vi "mainui.vi"() -> ()   [LabVIEW 2011]
uses:
  <vilib>/Platform/TimedLoop/XDataNode/timing_clust.ctl
  <vilib>/Platform/TimedLoop/XDataNode/nitl_modes.ctl
  <vilib>/Platform/TimedLoop/XDataNode/wakeup.ctl
  <vilib>/Utility/config.llb/Read Key (Double).vi
  <vilib>/Utility/config.llb/Read Key (I32).vi
  <vilib>/Utility/config.llb/Read Key (String).vi
  <vilib>/Utility/config.llb/Write Key (Double).vi
  <vilib>/Utility/config.llb/Write Key (I32).vi
  <vilib>/Utility/config.llb/Write Key (String).vi
  <vilib>/Platform/TimedLoop/XDataNode/XDataNode.xnode
  API/API DYM.lvlib
  <vilib>/Platform/TimedLoop/XDataNode/XDNodeRunTimeDep.lvlib
  <vilib>/Utility/config.llb/NI_LVConfig.lvlib
  API/ColorSensorlib.lvlib
panel:
  in  "Color_String":string
  out "Plat2CurrentY_Adv":i32
  out "Plat2CurrentX_Adv":i32
  out "Plat3CurrentY_Adv":i32
  out "Plat3CurrentX_Adv":i32
  out "while-control":bool
  out "Sensor array output":i32[](array[numeric])
  out "Plat2CurrentY":i32
  out "Plat2CurrentX":i32
  out "platformStatue0 output":i32[](array[numeric])
  out "platformStatue1 output":i32[](array[numeric])
  out "platformStatue2 output":i32[](array[numeric])
  out "CurrentPosY":i32
  out "CurrentPosX":i32
  out "motor statue array output":i32[](array[numeric])
  out "solenstatue output":i32[](array[numeric])
  in  "选项卡控件Next":T1(tab)
  in  "BaseBtn":bool
  in  "MotinAdv":bool
  in  "restartbtn":bool
  in  "No1Btn":bool
  in  "No2Btn":bool
  in  "No3Btn":bool
  in  "TogStartBtn":bool
  in  "TogReturnBtn":bool
  in  "TogStopBtn":bool
  in  "Plat1StopBtn":bool
  in  "Plat1ReturnBtn":bool
  in  "Plat1Btn":bool
  in  "Plat2Btn":bool
  in  "Plat2ReturnBtn":bool
  in  "Plat2StopBtn":bool
  in  "Plat3GetMegBtn":bool
  in  "Plat3MulitBtn":bool
  in  "Plat3ReturnBtn":bool
  in  "Plat3StopBtn":bool
  in  "Plat3Btn":bool
  in  "Sensor":bool
  in  "选项卡控件":T2(tab)
  out "Blue":i32
  out "Green":i32
  out "红外计数":dbl
  out "电涡流计数":dbl
  out "红外电平":i32
  out "电涡流电平":i32
  out "电容1":i32
  out "电容2":i32
  out "电容3":i32
  out "电桥电平":dbl
  out "电桥称重":dbl
  out "Waveform Chart":dynamicdata(graph)
  in  "颜色盒":u32(colorbox)
  out "Red":i32
  out "Red_Last":i32
  out "Green_Last":i32
  out "Blue_Last":i32
  in  "Collection_Color":u32(colorbox)
  out "Property_T":string
  out "M1":bool
  out "M2":bool
  out "M3":bool
  out "M4":bool
  out "M5":bool
  out "M6":bool
  out "Plat3IO1":bool
  out "Plat3IO2":bool
  out "Plat3IO3":bool
  out "Plat3IO4":bool
  out "Plat3IO5":bool
  out "Plat3IO6":bool
  out "Plat3IO7":bool
  out "Plat3IO8":bool
  out "Plat2IO1":bool
  out "Plat2IO2":bool
  out "Plat2IO3":bool
  out "Plat2IO4":bool
  out "Plat2IO5":bool
  out "Plat2IO6":bool
  out "Plat2IO7":bool
  out "Plat2IO8":bool
  out "Solen48":bool
  out "Solen47":bool
  out "Solen46":bool
  out "Solen45":bool
  out "Solen44":bool
  out "Solen43":bool
  out "Solen42":bool
  out "Solen41":bool
  out "Solen40":bool
  out "Solen39":bool
  out "Solen38":bool
  out "Solen37":bool
  out "Solen36":bool
  out "Solen35":bool
  out "Solen34":bool
  out "Solen33":bool
  out "Solen32":bool
  out "Solen31":bool
  out "Solen30":bool
  out "Solen29":bool
  out "Solen28":bool
  out "Solen27":bool
  out "Solen26":bool
  out "Solen25":bool
  out "Solen24":bool
  out "Solen23":bool
  out "Solen22":bool
  out "Solen21":bool
  out "Solen20":bool
  out "Solen19":bool
  out "Solen18":bool
  out "Solen17":bool
  out "Solen16":bool
  out "Solen15":bool
  out "Solen14":bool
  out "Solen13":bool
  out "Solen12":bool
  out "Solen11":bool
  out "Solen10":bool
  out "Solen9":bool
  out "Solen8":bool
  out "Solen7":bool
  out "Solen6":bool
  out "Solen5":bool
  out "Solen4":bool
  out "Solen3":bool
  out "Solen2":bool
  out "Solen1":bool
  out "Plat1IO1":bool
  out "Plat1IO2":bool
  out "Plat1IO3":bool
  out "Plat1IO4":bool
  out "Plat1IO5":bool
  out "Plat1IO6":bool
  out "Plat1IO7":bool
  out "Plat1IO8":bool
  in  "SensorWait":i32=1666
  in  "2to3Pos":i32=1666
  in  "1to2pos":i32=1666
  in  "Plat1_FeedMotorSpeed":i32=1666
  in  "Plat1SelectPolic1":string(combo)
  in  "Plat1SelectPolic2":string(combo)
  in  "Plat1SaveConfig":bool
  in  "Plat1SetResetConfig":bool
  in  "Plat2SendY":i32
  in  "Plat2RecvY":i32
  in  "Plat2SendX":i32
  in  "Plat2RecvX":i32
  in  "Plat2SelectPolicy":enum32{"使用最短路径算法", "使用最短时间算法", "使用默认速度算法"}(radio)
  in  "Plat2SaveConfig":bool
  in  "Plat2SetResetConfig":bool
  out "MaxSpeed 2":i32
  out "MinSpeed 2":i32
  in  "FirstPosX":i32
  in  "FirstPosZ":i32
  out "MinSpeed":i32
  out "MaxSpeed":i32
  in  "Horizontal4":i32
  in  "Horizontal3":i32
  in  "Horizontal2":i32
  in  "Horizontal1":i32
  in  "Vax4":i32
  in  "Vax3":i32
  in  "Vax2":i32
  in  "Vax1":i32
  in  "SaveParam":bool
  in  "CalcKB":bool
  out "BCalcd":dbl
  out "KCalcd":dbl
  out "Stog":dbl
  in  "Set2":bool
  in  "Set1":bool
  out "电桥电平_Event":dbl
  out "Volt2":dbl
  out "Volt1":dbl
  in  "X2":dbl
  in  "X1":dbl
  out "BCurrent":dbl
  out "KCurrent":dbl
  in  "SelectPolicy":enum32{"使用最短路径算法", "使用最短时间算法", "使用默认速度算法"}(radio)
  in  "ComboPolicy":string(combo)
  in  "ShowImg":bool
  in  "SaveConfigXZ":bool
  in  "SetReset":bool
  in  "MotorSpeed":i32=1
  in  "MotorSpeedNum":i32=1 min=1 max=6 step=1
  in  "SetMotorSpeed":bool
  out "Motor6Pos":i32
  out "Motor5Pos":i32
  out "Motor4Pos":i32
  out "Motor3Pos":i32
  out "Motor2Pos":i32
  out "Motor1Pos":i32
  in  "ClearPos6":bool
  in  "ClearPos5":bool
  in  "ClearPos4":bool
  in  "ClearPos3":bool
  in  "ClearPos2":bool
  in  "ClearPos1":bool
  in  "StopMotorNum":i32=1 min=1 max=6 step=1
  in  "StepNum":i32=1 min=1 max=20000 step=1
  in  "Directon":string(combo)
  in  "MotorNum":i32=1 min=1 max=6 step=1
  in  "SolenPlatStatue_Event":string(combo)
  in  "SolenPlat_Event":i32 min=0 max=2 step=1
  in  "SolenStatue_Event":string(combo)
  in  "SolenNum_Event":i32 min=0 max=47 step=1
  in  "MotorStop":bool
  in  "MotorStart":bool
  in  "FeedMotorStop":bool
  in  "FeedMotorStart":bool
  in  "SolenAdvance":bool
  in  "SolenAction":bool
  out "指令数":i32
  out "Statue":bool
  in  "start":bool
  in  "stop":bool
  in  "statuebtn":bool
  in  "no3btn":bool
  in  "no2btn":bool
  in  "no1btn":bool
  # "连接状态"
  # "待执行指令"
  # "红外计数"
  # "电涡流计数"
  # "电桥物体称重"
  # "检测到物体属性"
  # "检测到颜色"
  # "红外传感器电平"
  # "电涡流传感器电平"
  # "电容式传感器1电平"
  # "电容式传感器2电平"
  # "电容式传感器3电平"
  # "电桥传感器电平"
  # "颜色传感器"
  # "继电器状态"
  # "输入口状态"
  # "电机运行状态"
  # "进料电机速度"
  # "脉冲/S"
  # "1号选料槽选取性质"
  # "1号传感器→2号传感器相对位移"
  # "步"
  # "2号选料槽选取性质"
  # "2号传感器→3号传感器相对位移"
  # "步"
  # "传感器检测时间"
  # "毫秒"
  # "点位控制参数"
  # "平台接料点定位坐标X"
  # "平台接料点定位坐标Y"
  # "平台捡料点定位坐标X"
  # "平台捡料点定位坐标Y"
  # "电机参数"
  # "电机最大速度"
  # "电机最小速度"
  # "脉冲/S"
  # "脉冲/S"
  # "电机联动算法"
  # "当前电桥传感器矫正参数"
  # "g"
  # "K值"
  # "B值"
  # "当前传感器电压"
  # "mv"
  # "当前转换重量"
  # "电桥传感器参数标定"
  # "K值"
  # "B值"
  # "g"
  # "砝码重量1"
  # "对应电压"
  # "mv"
  # "砝码重量2"
  # "对应电压"
  # "g"
  # "mv"
  # "立体仓库坐标参数"
  # "放料点坐标Z轴"
  # "放料点坐标X轴"
  # "第一行定位坐标Z轴"
  # "第一列定位坐标X轴"
  # "第二行定位坐标Z轴"
  # "第二列定位坐标X轴"
  # "第三行定位坐标Z轴"
  # "第三列定位坐标X轴"
  # "第四行定位坐标Z轴"
  # "第四列定位坐标X轴"
  # "电机参数"
  # "放置策略"
  # "电机最大速度"
  # "电机最小速度"
  # "策略选择"
  # "脉冲/S"
  # "脉冲/S"
  # "电机联动算法"
  # "继电器状态"
  # "继电器编号"
  # "继电器状态"
  # "平台编号"
  # "(进料电机运行)"
  # "电机速度"
  # "电机编号"
  # "脉冲/S"
  # "(进料电机停止)"
  # "电机编号"
  # "方向"
  # "步数"
  # "(1-20000)"
  # "电机编号"
  # "1号电机位置值:"
  # "4号电机位置值:"
  # "2号电机位置值:"
  # "5号电机位置值:"
  # "3号电机位置值:"
  # "6号电机位置值:"
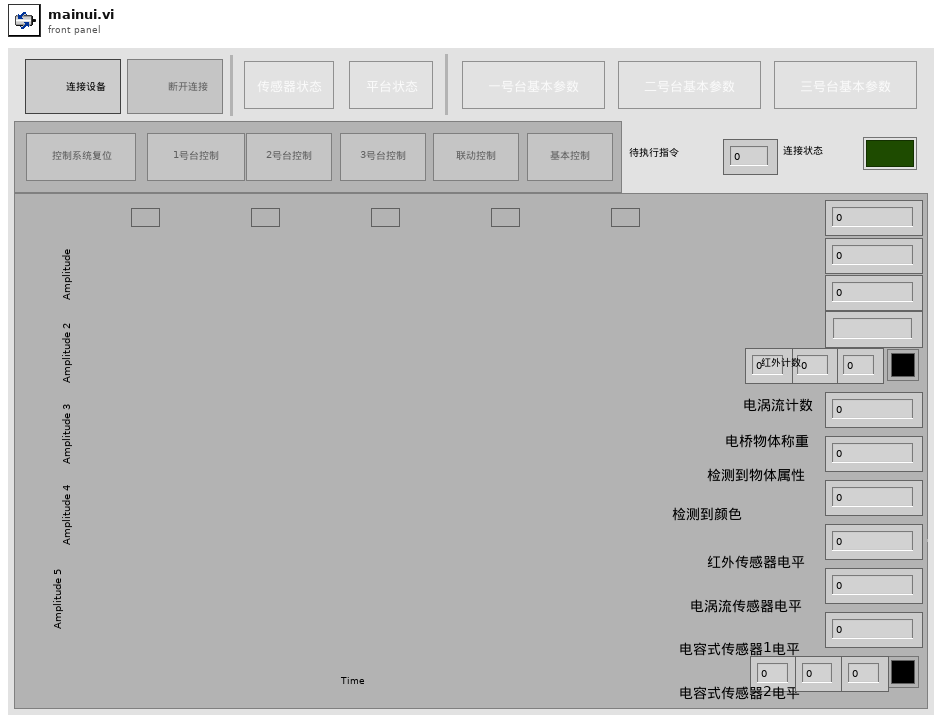
[diagram p1: front panel]
types:
  T1 = enum32{"选项卡 1", "选项卡 2", "选项卡 3", "选项卡 4", "选项卡 5"}
  T2 = enum32{"选项卡 1", "选项卡 2", "选项卡 3", "选项卡 4", "选项卡 5", "选项卡 6"}
  T3 = enum8{"Enabled", "Disabled", "Disabled and Grayed Out"}
  T4 = enum16{"None", "GetSensorStatue", "GetSensorAD", "GetSolenStatue", "GetPaltformStatue", "GetMotorStatue", "FeedMotorStart", "FeedMotorStop", "MotorStart", "MotorRestart", "MotorStop", "SolenAction", "SolenAdv", "RcvDataInit", "SetMotorSpeed", "Delay"}
  T5 = typedef "NI_LVConfig.lvlib/Config Data RefNum.ctl" = refnum<k1>
  T6 = enum32{"选项卡 1", "选项卡 2", "选项卡 3", "选项卡 4", "选项卡 5", "选项卡 6", "选项卡 7"}
  T7 = enum16{"None", "GetSensorStatue", "GetSensorAD", "GetSolenStatue", "GetPaltformStatue", "GetMotorStatue", "FeedMotorStart", "FeedMotorStop", "MotorStart", "MotorRestart", "MotorStop", "SolenAction", "SolenAdv"}
  T8 = enum16{"None", "GetSensorStatue", "GetSensorAD", "GetSolenStatue", "GetPaltformStatue", "GetMotorStatue", "FeedMotorStart", "FeedMotorStop", "MotorStart", "MotorRestart", "MotorStop", "SolenAction", "SolenAdv", "RcvDataInit", "SetMotorSpeed"}
  T9 = enum16{"初始化选择器", "1号料槽选料", "2号料槽选料", "取料动作", "Stop"}
  T10 = enum16{"None", "GetSensorStatue", "GetSensorAD", "GetSolenStatue", "GetPaltformStatue", "GetMotorStatue", "FeedMotorStart", "FeedMotorStop", "MotorStart", "MotorRestart", "MotorStop", "SolenAction", "SolenAdv", "RcvDataInit"}
  T11 = typedef "XDNodeRunTimeDep.lvlib/timing_clust.ctl" = cluster{"Expected End [f-1]":u64, "Actual End [f-1]":u64, "Finished Late? [f-1]":bool, "Expected End [i-1]":u64, "Actual End [i-1]":u64, "Finished Late? [i-1]":bool, "Expected Start [i]":u64, "Actual Start [i]":u64, "Expected Start [f]":u64, "Actual Start [f]":u64, "Source Name":string, "Structure Name":string, "Period":i64, "Deadline":i64, "Offset":i64, "Start":i64, "Priority":i32, "Timeout":i32, "Mode":T12, "Wakeup Reason":T13, "Error":errorcluster, "Source Type":string, "Secondary Source Type":string, "Global End Time":u64, "Global Start Time":u64, "Frame Duration":u64, "Iteration Duration":u64, "Assigned CPU":i32, "I/O Scan Engine Mode":u32}
  T12 = typedef "XDNodeRunTimeDep.lvlib/nitl_modes.ctl" = enum32{"No Change", "Process missed periods, maintain original phase", "Discard missed periods, maintain original phase", "Process missed periods, ignore original phase", "Discard missed periods, ignore original phase"}
  T13 = typedef "XDNodeRunTimeDep.lvlib/wakeup.ctl" = enum32{"Normal", "Aborted", "Asynchronous wakeup", "Timing source error", "Timed loop error", "Timeout"}
  T14 = enum16{"1号台推料检测", "1号台取料", "1号台放料", "检测策略选择", "使能取料槽1", "使能取料槽2"}
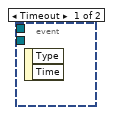
[diagram p2: hidden frame]
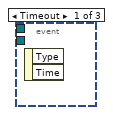
[diagram p3: hidden frame]
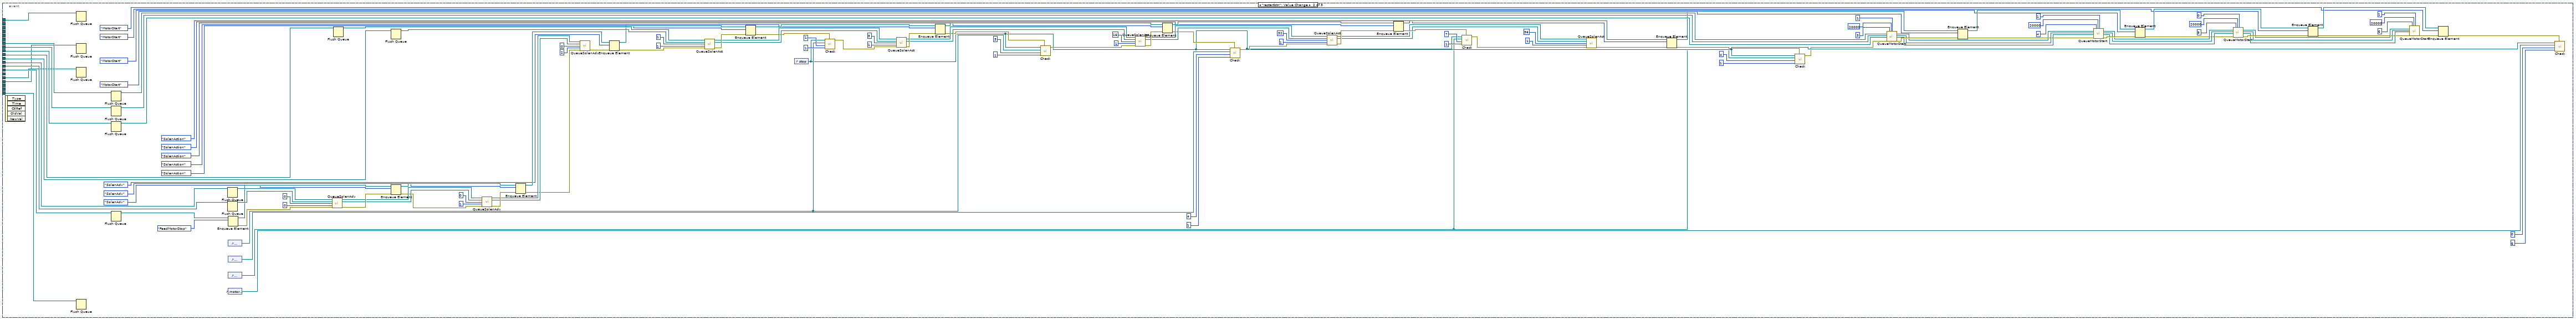
[diagram p4: hidden frame]
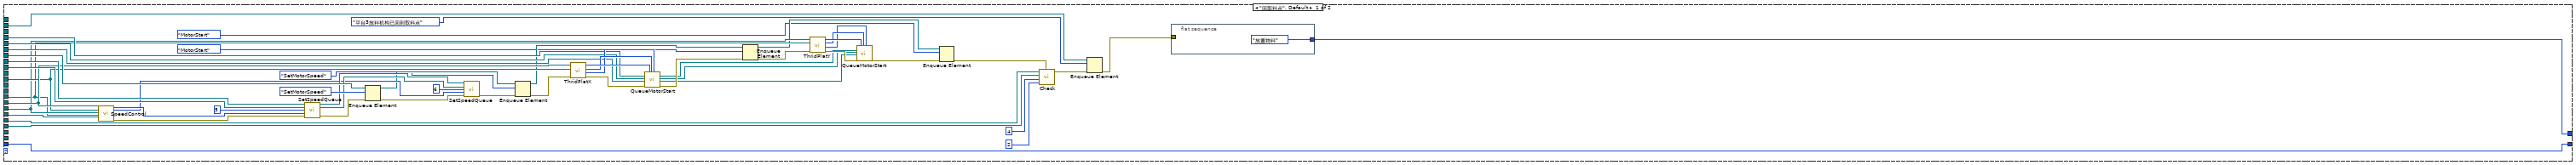
[diagram p5: hidden frame]
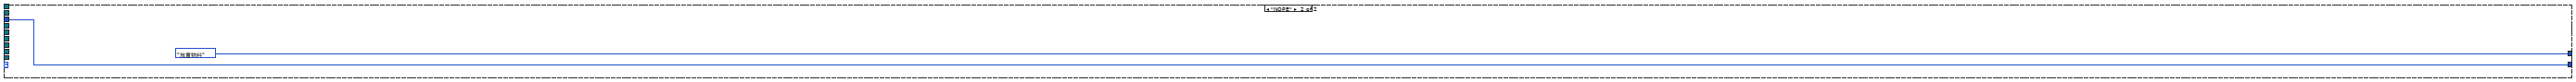
[diagram p7: hidden frame]
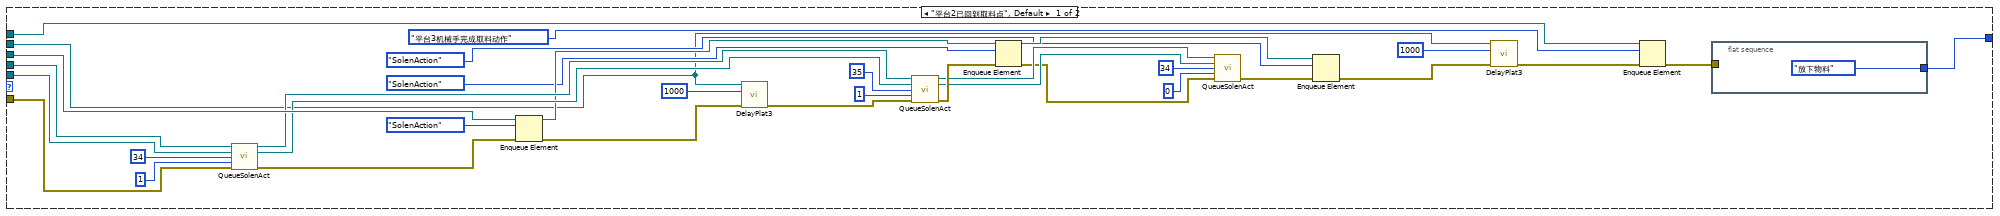
[diagram p8: hidden frame]
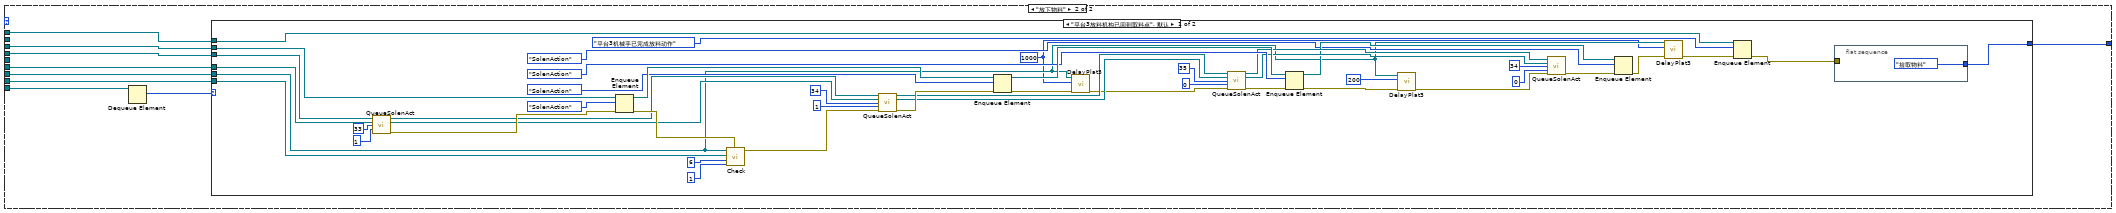
[diagram p9: hidden frame]
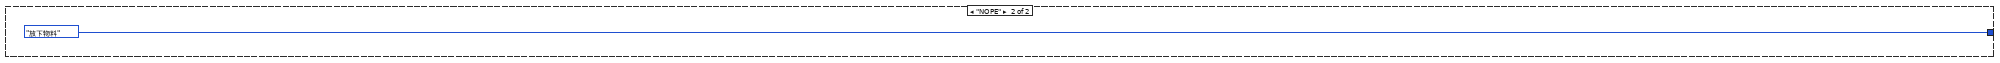
[diagram p10: hidden frame]
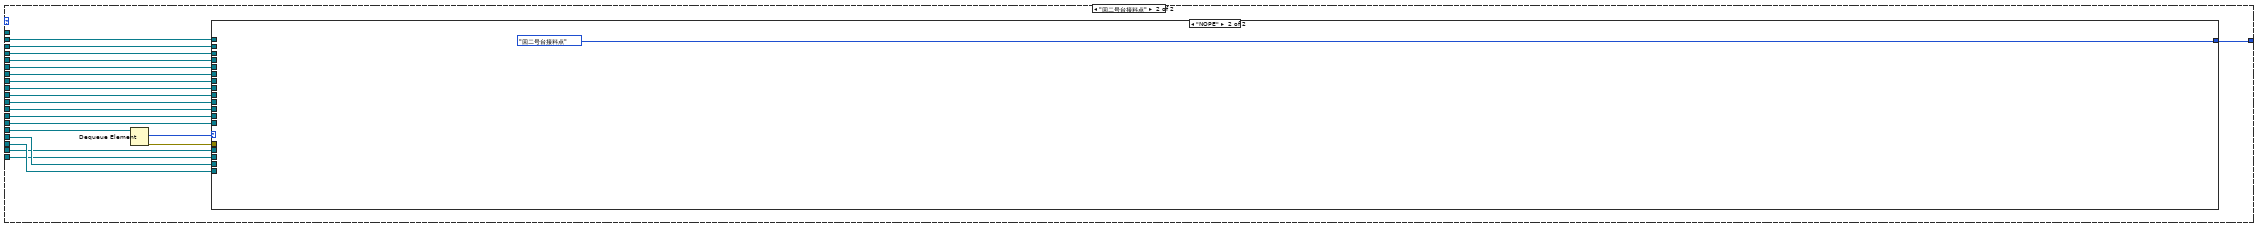
[diagram p11: hidden frame]
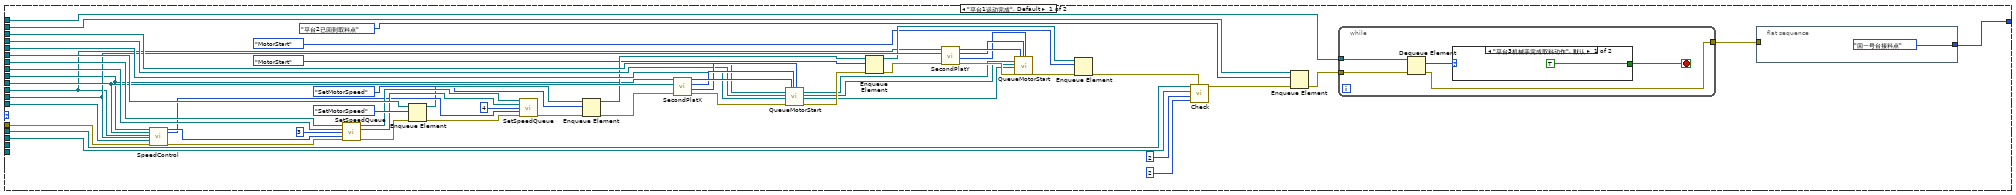
[diagram p12: hidden frame]
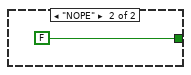
[diagram p13: hidden frame]
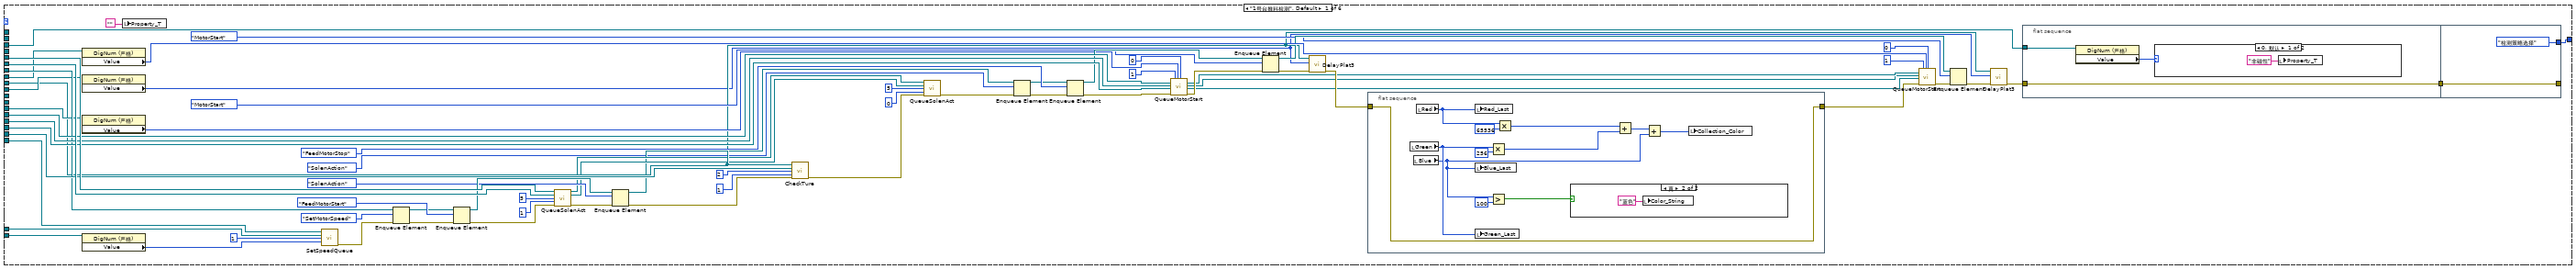
[diagram p14: hidden frame]
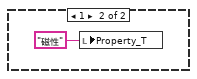
[diagram p15: hidden frame]
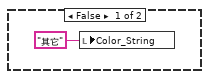
[diagram p16: hidden frame]
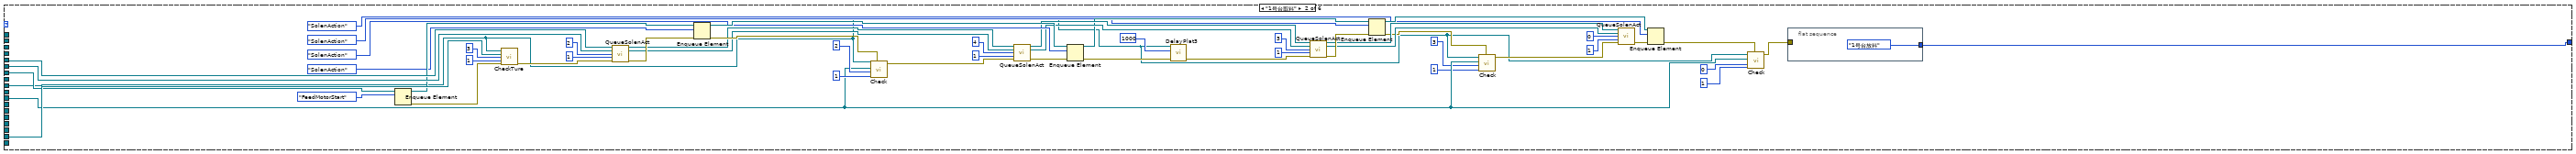
[diagram p17: hidden frame]
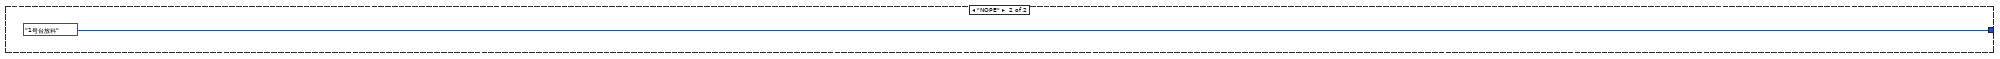
[diagram p18: hidden frame]
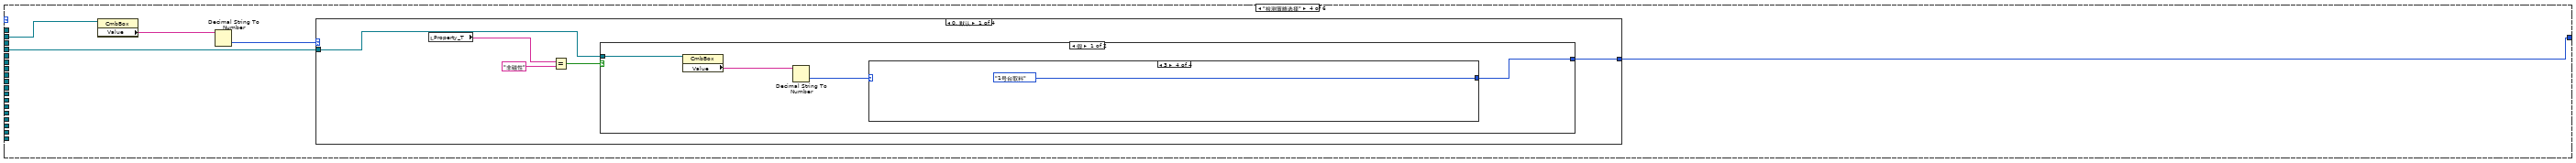
[diagram p19: hidden frame]
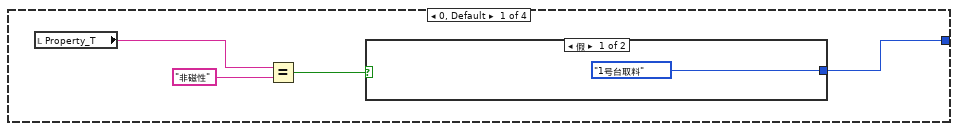
[diagram p20: hidden frame]
diagram:
  w55 = "FirstPlat" ("section")
  w110 = "SecondPlat" ("section")
  w146 = "ThridPlat" ("section")
  w297 = 0 ("Motor1Pos")
  w312 = 0
  w339 = 0
  w358 = 0.0
  n1 = while {
    stop <- FALSE stop-if-true
    n2 = event shown="[6] \"BaseBtn\": 值改变" {
      selector: _ -> [_ _ _ _ _ _ _]
      dyn-events: _ -> [_ _ _ _ _ _ _]
      timeout: _ -> [_ _ _ _ _ _ _]
      event Timeout {
        n3 = event-data() -> ()  [unwired: 1 in, 2 out]
      }
      event "statuebtn": Value Change {
        n4 = event-data() -> ()  [unwired: 1 in, 5 out]
        n5 = property on="选项卡控件" class="TabCtl (严格)"("Value"=T2."选项卡 2" ("选项卡控件")) -> ()  [unwired: 2 in, 2 out]
      }
      event "no1btn": Value Change {
        n6 = event-data() -> ()  [unwired: 1 in, 5 out]
        n7 = property on="选项卡控件" class="TabCtl (严格)"("Value"=T2."选项卡 3" ("选项卡控件")) -> ()  [unwired: 2 in, 2 out]
      }
      event "no2btn": Value Change {
        n8 = event-data() -> ()  [unwired: 1 in, 5 out]
        n9 = property on="选项卡控件" class="TabCtl (严格)"("Value"=T2."选项卡 4" ("选项卡控件")) -> ()  [unwired: 2 in, 2 out]
      }
      event "no3btn": Value Change {
        n10 = event-data() -> ()  [unwired: 1 in, 5 out]
        n11 = property on="选项卡控件" class="TabCtl (严格)"("Value"=T2."选项卡 5" ("选项卡控件")) -> ()  [unwired: 2 in, 2 out]
      }
      event "Sensor": Value Change {
        n12 = event-data() -> ()  [unwired: 1 in, 5 out]
        n13 = property on="选项卡控件" class="TabCtl (严格)"("Value"=T2."选项卡 1" ("选项卡控件")) -> ()  [unwired: 2 in, 2 out]
      }
      event "BaseBtn": Value Change {
        n14 = event-data() -> ()  [unwired: 1 in, 5 out]
        n15 = property on="选项卡控件" class="TabCtl (严格)"("Value"=T2."选项卡 6" ("选项卡控件")) -> ()  [unwired: 2 in, 2 out]
      }
    }
  }
  n16 = property on="MotorNum" class="DigNum (严格)"("Value"=1 ("MotorNum")) -> (error out=w303:errorcluster)  [unwired: 2 in, 1 out]
  n17 = Current VI's Path() -> (path=w291:path)
  n18 = property on="StepNum" class="DigNum (严格)"(error in=w303, "Value"=2000 ("StepNum")) -> (error out=w306:errorcluster)  [unwired: 1 in, 1 out]
  n19 = Build Path(base path=w291, name or relative path="..\\Config.ini" ("名称或相对路径")) -> (appended path=w289:path)
  n20 = call <vilib>:"Open Config Data.vi"("create file if necessary (T)"=TRUE, "configuration file path"=w289) -> ("error out"=w286:errorcluster, "refnum"=w287:T5)  [unwired: 7 in, 1 out]
  n21 = property on="Directon" class="CmbBox"(error in=w306, "Value"="1" ("Directon")) -> (error out=w307:errorcluster)  [unwired: 1 in, 1 out]
  n22 = property on="StopMotorNum" class="DigNum (严格)"(error in=w307, "Value"=1 ("StopMotorNum")) -> (error out=w309:errorcluster)  [unwired: 1 in, 1 out]
  n23 = call-poly <vilib>:"Read Key.vi"("section"=w146, "error in (no error)"=w286, "key"="KValue", "refnum"=w287) -> ("error out"=w282:errorcluster, "value"=w283:dbl, "found?"=w284:bool, "refnum out"=w281:T5)  [unwired: 4 in]
  n24 = case shown="真" w284 {
    tunnel: w283 -> [_ w378]
    tunnel: w282 -> [w373 w377]
    tunnel: [w373 w376] -> w279
    tunnel: [w374 w375] -> w280
    tunnel: w281 -> [w374 w375]
    frame False {
    }
    frame True {
      n25 = property on="KCurrent" class="DigNum (严格)"(error in=w377, "Value"=w378) -> (error out=w376:errorcluster)  [unwired: 1 in, 1 out]
    }
  }
  n26 = property on="SolenPlatStatue_Event" class="CmbBox"(error in=w309, "Value"="1" ("SolenPlatStatue_Event")) -> (error out=w315:errorcluster)  [unwired: 1 in, 1 out]
  n27 = call-poly <vilib>:"Read Key.vi"("section"=w146, "error in (no error)"=w279, "key"="BValue", "refnum"=w280) -> ("error out"=w275:errorcluster, "value"=w274:dbl, "found?"=w277:bool, "refnum out"=w276:T5)  [unwired: 4 in]
  n28 = property on="Motor1Pos" class="DigNum (严格)"("Value"=w297) -> (error out=w301:errorcluster)  [unwired: 2 in, 1 out]
  n29 = case shown="真" w277 {
    tunnel: [w380 w384] -> w273
    tunnel: w276 -> [w380 w384]
    tunnel: w275 -> [w379 w383]
    tunnel: [w379 w382] -> w272
    tunnel: w274 -> [_ w381]
    frame False {
    }
    frame True {
      n30 = property on="BCurrent" class="DigNum (严格)"(error in=w383, "Value"=w381) -> (error out=w382:errorcluster)  [unwired: 1 in, 1 out]
    }
  }
  n31 = property on="SolenPlat_Event" class="DigNum (严格)"(error in=w315, "Value"=0 ("SolenPlat_Event")) -> (error out=w317:errorcluster)  [unwired: 1 in, 1 out]
  n32 = property on="Motor2Pos" class="DigNum (严格)"(error in=w301, "Value"=w297) -> (error out=w302:errorcluster)  [unwired: 1 in, 1 out]
  n33 = property on="Motor3Pos" class="DigNum (严格)"(error in=w302, "Value"=w297) -> (error out=w300:errorcluster)  [unwired: 1 in, 1 out]
  n34 = call-poly <vilib>:"Read Key.vi"("section"=w146, "error in (no error)"=w272, "key"="Z1Pos", "refnum"=w273) -> ("error out"=w268:errorcluster, "value"=w267:i32, "found?"=w270:bool, "refnum out"=w269:T5)  [unwired: 4 in]
  n35 = property on="SolenStatue_Event" class="CmbBox"(error in=w317, "Value"="1" ("SolenStatue_Event")) -> (error out=w321:errorcluster)  [unwired: 1 in, 1 out]
  n36 = case shown="真" w270 {
    tunnel: [w386 w390] -> w266
    tunnel: w269 -> [w386 w390]
    tunnel: w268 -> [w385 w389]
    tunnel: [w385 w388] -> w265
    tunnel: w267 -> [_ w387]
    frame False {
    }
    frame True {
      n37 = property on="Vax1" class="DigNum (严格)"(error in=w389, "Value"=w387) -> (error out=w388:errorcluster)  [unwired: 1 in, 1 out]
    }
  }
  n38 = property on="MotorSpeedNum" class="DigNum (严格)"("Value"=1 ("MotorSpeedNum")) -> (error out=w213:errorcluster)  [unwired: 2 in, 1 out]
  n39 = property on="Motor4Pos" class="DigNum (严格)"(error in=w300, "Value"=w297) -> (error out=w299:errorcluster)  [unwired: 1 in, 1 out]
  n40 = control-ref of="本VI"() -> (w357:refnum<vi>)
  n41 = property on="电桥电平" class="DigNum (严格)"("Value"=w358) -> ()  [unwired: 2 in, 2 out]
  n42 = property on="红外电平" class="DigNum (严格)"("Value"=w358) -> ()  [unwired: 2 in, 2 out]
  n43 = property on="电容1" class="DigNum (严格)"("Value"=w358) -> ()  [unwired: 2 in, 2 out]
  n44 = property on="电容2" class="DigNum (严格)"("Value"=w358) -> ()  [unwired: 2 in, 2 out]
  n45 = property on="电容3" class="DigNum (严格)"("Value"=w358) -> ()  [unwired: 2 in, 2 out]
  n46 = property on="电涡流电平" class="DigNum (严格)"("Value"=w358) -> ()  [unwired: 2 in, 2 out]
  n47 = property on="电涡流计数" class="DigNum (严格)"("Value"=w358) -> ()  [unwired: 2 in, 2 out]
  n48 = call-poly <vilib>:"Read Key.vi"("section"=w146, "error in (no error)"=w265, "key"="Z2Pos", "refnum"=w266) -> ("error out"=w261:errorcluster, "value"=w260:i32, "found?"=w263:bool, "refnum out"=w262:T5)  [unwired: 4 in]
  n49 = property on="Motor5Pos" class="DigNum (严格)"(error in=w299, "Value"=w297) -> (error out=w298:errorcluster)  [unwired: 1 in, 1 out]
  n50 = case shown="真" w263 {
    tunnel: w262 -> [w392 w396]
    tunnel: [w392 w396] -> w259
    tunnel: w261 -> [w391 w394]
    tunnel: w260 -> [_ w395]
    tunnel: [w391 w393] -> w258
    frame False {
    }
    frame True {
      n51 = property on="Vax2" class="DigNum (严格)"(error in=w394, "Value"=w395) -> (error out=w393:errorcluster)  [unwired: 1 in, 1 out]
    }
  }
  n52 = property class="VI"(reference=w357, "Front Panel.Open"=TRUE ("前面板窗口:打开")) -> (reference out=w355:refnum<vi>, error out=w354:errorcluster)  [unwired: 1 in]
  n53 = control-ref of="Vax1"() -> (w160:refnum<vi>)
  n54 = control-ref of="Vax2"() -> (w159:refnum<vi>)
  n55 = control-ref of="Vax3"() -> (w158:refnum<vi>)
  n56 = control-ref of="Vax4"() -> (w157:refnum<vi>)
  n57 = control-ref of="Horizontal1"() -> (w164:refnum<vi>)
  n58 = control-ref of="Horizontal2"() -> (w163:refnum<vi>)
  n59 = control-ref of="Horizontal3"() -> (w162:refnum<vi>)
  n60 = control-ref of="Horizontal4"() -> (w161:refnum<vi>)
  n61 = call-poly <vilib>:"Read Key.vi"("section"=w146, "error in (no error)"=w258, "key"="Z3Pos", "refnum"=w259) -> ("error out"=w254:errorcluster, "value"=w253:i32, "found?"=w256:bool, "refnum out"=w255:T5)  [unwired: 4 in]
  n62 = case shown="真" w256 {
    tunnel: w255 -> [w398 w402]
    tunnel: [w398 w402] -> w252
    tunnel: w254 -> [w397 w400]
    tunnel: w253 -> [_ w401]
    tunnel: [w397 w399] -> w251
    frame False {
    }
    frame True {
      n63 = property on="Vax3" class="DigNum (严格)"(error in=w400, "Value"=w401) -> (error out=w399:errorcluster)  [unwired: 1 in, 1 out]
    }
  }
  n64 = property on="SolenNum_Event" class="DigNum (严格)"(error in=w321, "Value"=0 ("SolenNum_Event")) -> (error out=w323:errorcluster)  [unwired: 1 in, 1 out]
  n65 = property on="Waveform Chart" class="WFChart (严格)"("History Data"=dynamicdata[] [] ("历史数据")) -> (error out=w363:errorcluster)  [unwired: 2 in, 1 out]
  n66 = property on="选项卡控件Next" class="TabCtl (严格)"("Value"=enum32{"选项卡 1", "选项卡 2"}."选项卡 1" ("选项卡控件Next")) -> (error out=w171:errorcluster)  [unwired: 2 in, 1 out]
  n67 = property on="MotorSpeed" class="DigNum (严格)"(error in=w213, "Value"=100 ("MotorSpeed")) -> (error out=w212:errorcluster)  [unwired: 1 in, 1 out]
  n68 = property on="Motor6Pos" class="DigNum (严格)"(error in=w298, "Value"=w297) -> (error out=w296:errorcluster)  [unwired: 1 in, 1 out]
  n69 = property class="VI"(reference=w355, error in=w354, "Front Panel.IsFrontmost"=TRUE ("前面板窗口:在最前")) -> (reference out=w353:refnum<vi>, error out=w352:errorcluster)
  n70 = property on="TogStopBtn" class="Bool (严格)"("Value"=FALSE ("TogStopBtn")) -> (error out=w1:errorcluster)  [unwired: 2 in, 1 out]
  n71 = property on="restartbtn" class="Bool"("DisabledEnum"=T3."Disabled and Grayed Out" ("禁用")) -> (error out=w347:errorcluster)  [unwired: 2 in, 1 out]
  n72 = property on="选项卡控件" class="TabCtl (严格)"("Value"=T2."选项卡 1" ("选项卡控件")) -> (error out=w334:errorcluster)  [unwired: 2 in, 1 out]
  n73 = Build Array(w160, w159, w158, w157) -> (w10:refnum<vi>[])
  n74 = Build Array(w164, w163, w162, w161) -> (w9:refnum<vi>[])
  n75 = property on="start" class="Bool"("DisabledEnum"=T3."Enabled" ("禁用")) -> (error out=w362:errorcluster)  [unwired: 2 in, 1 out]
  n76 = property on="stop" class="Bool (严格)"("DisabledEnum"=T3."Disabled and Grayed Out" ("禁用")) -> (error out=w361:errorcluster)  [unwired: 2 in, 1 out]
  n77 = property on="No1Btn" class="Bool"("DisabledEnum"=T3."Disabled and Grayed Out" ("禁用")) -> (error out=w333:errorcluster)  [unwired: 2 in, 1 out]
  n78 = property on="No2Btn" class="Bool"("DisabledEnum"=T3."Disabled and Grayed Out" ("禁用")) -> (error out=w331:errorcluster)  [unwired: 2 in, 1 out]
  n79 = property on="No3Btn" class="Bool"("DisabledEnum"=T3."Disabled and Grayed Out" ("禁用")) -> (error out=w330:errorcluster)  [unwired: 2 in, 1 out]
  n80 = property on="BaseBtn" class="Bool"("DisabledEnum"=T3."Disabled and Grayed Out" ("禁用")) -> (error out=w327:errorcluster)  [unwired: 2 in, 1 out]
  n81 = property on="MotinAdv" class="Bool"("DisabledEnum"=T3."Disabled and Grayed Out" ("禁用")) -> (error out=w325:errorcluster)  [unwired: 2 in, 1 out]
  n82 = property on="红外计数" class="DigNum (严格)"("Value"=w358) -> (error out=w365:errorcluster)  [unwired: 2 in, 1 out]
  n83 = property on="Statue" class="Bool (严格)"("Value"=FALSE ("Statue")) -> (error out=w349:errorcluster)  [unwired: 2 in, 1 out]
  n84 = property on="stop" class="Bool (严格)"("Value"=FALSE ("stop")) -> (error out=w343:errorcluster)  [unwired: 2 in, 1 out]
  n85 = Obtain Queue(name (unnamed)="3号台_仓库2维运动队列" ("名称（未命名）"), element data type=enum16{"仓库2维运动完成", "NOPE"}."NOPE") -> (queue out=w43:refnum<queue>, error out=w38:errorcluster)  [unwired: 3 in, 1 out]
  n86 = Obtain Queue(name (unnamed)="3号台_机械手队列" ("名称（未命名）"), element data type=enum16{"机械手动作完成", "NOPE"}."NOPE") -> (queue out=w42:refnum<queue>, error out=w39:errorcluster)  [unwired: 3 in, 1 out]
  n87 = Obtain Queue(name (unnamed)="平台2与平台3机械手通讯" ("名称（未命名）"), element data type=enum16{"平台2已回到取料点", "NOPE"}."NOPE") -> (queue out=w6:refnum<queue>)  [unwired: 3 in, 2 out]
  n88 = Obtain Queue(name (unnamed)="平台3机械手与平台2通讯" ("名称（未命名）"), element data type=enum16{"平台3机械手完成取料动作", "NOPE"}."NOPE") -> (queue out=w5:refnum<queue>)  [unwired: 3 in, 2 out]
  n89 = Obtain Queue(name (unnamed)="平台1与平台2通讯" ("名称（未命名）"), element data type=enum16{"平台1运动完成", "NOPE"}."NOPE") -> (queue out=w8:refnum<queue>)  [unwired: 3 in, 2 out]
  n90 = Obtain Queue(name (unnamed)="平台2与平台1通讯" ("名称（未命名）"), element data type=enum16{"平台2已回到接料点", "NOPE"}."NOPE") -> (queue out=w7:refnum<queue>)  [unwired: 3 in, 2 out]
  n91 = Obtain Queue(name (unnamed)="平台3放料机构与平台3机械手通讯" ("名称（未命名）"), element data type=enum16{"平台3放料机构已回到取料点", "NOPE"}."NOPE") -> (queue out=w3:refnum<queue>)  [unwired: 3 in, 2 out]
  n92 = Obtain Queue(name (unnamed)="平台3机械手与平台3放料机构通讯" ("名称（未命名）"), element data type=enum16{"平台3机械手已完成放料动作", "NOPE"}."NOPE") -> (queue out=w4:refnum<queue>)  [unwired: 3 in, 2 out]
  n93 = Obtain Queue(name (unnamed)="SolenAction_Num" ("名称（未命名）"), element data type=w312) -> (queue out=w33:refnum<queue>, error out=w319:errorcluster)  [unwired: 3 in, 1 out]
  n94 = Obtain Queue(name (unnamed)="SolenAction_Statue" ("名称（未命名）"), element data type=w312) -> (queue out=w32:refnum<queue>, error out=w318:errorcluster)  [unwired: 3 in, 1 out]
  n95 = Obtain Queue(name (unnamed)="MotorNum" ("名称（未命名）"), element data type=w339) -> (queue out=w36:refnum<queue>, error out=w311:errorcluster)  [unwired: 3 in, 1 out]
  n96 = Obtain Queue(name (unnamed)="StopMotor_Num" ("名称（未命名）"), element data type=w312) -> (queue out=w37:refnum<queue>, error out=w165:errorcluster)  [unwired: 3 in, 1 out]
  n97 = Obtain Queue(name (unnamed)="SolenAdv_PlatNum" ("名称（未命名）"), element data type=w312) -> (queue out=w30:refnum<queue>, error out=w169:errorcluster)  [unwired: 3 in, 1 out]
  n98 = Obtain Queue(name (unnamed)="SolenAdv_Statue" ("名称（未命名）"), element data type=w312) -> (queue out=w31:refnum<queue>, error out=w168:errorcluster)  [unwired: 3 in, 1 out]
  n99 = Obtain Queue(name (unnamed)="Direction" ("名称（未命名）"), element data type=w339) -> (queue out=w34:refnum<queue>, error out=w166:errorcluster)  [unwired: 3 in, 1 out]
  n100 = Obtain Queue(name (unnamed)="Delay_Time" ("名称（未命名）"), element data type=u32 0) -> (queue out=w26:refnum<queue>, error out=w139:errorcluster)  [unwired: 3 in, 1 out]
  n101 = Obtain Queue(name (unnamed)="SetSpeed_MotorNum" ("名称（未命名）"), element data type=0) -> (queue out=w28:refnum<queue>, error out=w205:errorcluster)  [unwired: 3 in, 1 out]
  n102 = Obtain Queue(name (unnamed)="SetSpeed_SpeedValue" ("名称（未命名）"), element data type=0) -> (queue out=w27:refnum<queue>, error out=w204:errorcluster)  [unwired: 3 in, 1 out]
  n103 = Obtain Queue(name (unnamed)="Step" ("名称（未命名）"), element data type=w339) -> (queue out=w35:refnum<queue>, error out=w167:errorcluster)  [unwired: 3 in, 1 out]
  n104 = Obtain Queue(name (unnamed)="Cmd" ("名称（未命名）"), element data type=T4."None") -> (queue out=w29:refnum<queue>, error out=w170:errorcluster)  [unwired: 3 in, 1 out]
  n105 = call-poly <vilib>:"Read Key.vi"("section"=w146, "error in (no error)"=w251, "key"="Z4Pos", "refnum"=w252) -> ("error out"=w247:errorcluster, "value"=w246:i32, "found?"=w249:bool, "refnum out"=w248:T5)  [unwired: 4 in]
  n106 = case shown="真" w249 {
    tunnel: w248 -> [w404 w408]
    tunnel: w247 -> [w403 w406]
    tunnel: [w404 w408] -> w245
    tunnel: w246 -> [_ w407]
    tunnel: [w403 w405] -> w244
    frame False {
    }
    frame True {
      n107 = property on="Vax4" class="DigNum (严格)"(error in=w406, "Value"=w407) -> (error out=w405:errorcluster)  [unwired: 1 in, 1 out]
    }
  }
  n108 = call-poly <vilib>:"Read Key.vi"("section"=w146, "error in (no error)"=w244, "key"="X1Pos", "refnum"=w245) -> ("error out"=w241:errorcluster, "value"=w240:i32, "found?"=w239:bool, "refnum out"=w242:T5)  [unwired: 4 in]
  n109 = case shown="真" w239 {
    tunnel: w242 -> [w410 w414]
    tunnel: w241 -> [w409 w412]
    tunnel: [w410 w414] -> w238
    tunnel: w240 -> [_ w413]
    tunnel: [w409 w411] -> w237
    frame False {
    }
    frame True {
      n110 = property on="Horizontal1" class="DigNum (严格)"(error in=w412, "Value"=w413) -> (error out=w411:errorcluster)  [unwired: 1 in, 1 out]
    }
  }
  n111 = call-poly <vilib>:"Read Key.vi"("section"=w146, "error in (no error)"=w237, "key"="X2Pos", "refnum"=w238) -> ("error out"=w231:errorcluster, "value"=w230:i32, "found?"=w233:bool, "refnum out"=w232:T5)  [unwired: 4 in]
  n112 = while {
    tunnel: w170 -> [w431]
    tunnel: w29 -> [w432]
    tunnel: w35 -> [w430]
    tunnel: w167 -> [w429]
    tunnel: w34 -> [w428]
    tunnel: w166 -> [w427]
    tunnel: w36 -> [w426]
    tunnel: w311 -> [w425]
    tunnel: w33 -> [w424]
    tunnel: w32 -> [w423]
    tunnel: w30 -> [w422]
    tunnel: w31 -> [w421]
    tunnel: w319 -> [w420]
    tunnel: w318 -> [w419]
    tunnel: w169 -> [w418]
    tunnel: w168 -> [w417]
    tunnel: w37 -> [w416]
    tunnel: w165 -> [w415]
    stop <- FALSE stop-if-true
    n113 = event shown="[4] \"MotinAdv\": 值改变" {
      selector: _ -> [_ _ _ _ _ _ _ _ _]
      dyn-events: _ -> [_ _ _ _ _ _ _ _ _]
      timeout: _ -> [_ _ _ _ _ _ _ _ _]
      tunnel: w432 -> [_ _ _ _ _ _ _ _ _]
      tunnel: w431 -> [_ _ _ _ _ _ _ _ _]
      tunnel: w430 -> [_ _ _ _ _ _ _ _ _]
      tunnel: w429 -> [_ _ _ _ _ _ _ _ _]
      tunnel: w428 -> [_ _ _ _ _ _ _ _ _]
      tunnel: w427 -> [_ _ _ _ _ _ _ _ _]
      tunnel: w426 -> [_ _ _ _ _ _ _ _ _]
      tunnel: w425 -> [_ _ _ _ _ _ _ _ _]
      tunnel: w424 -> [_ _ _ _ _ _ _ _ _]
      tunnel: w423 -> [_ _ _ _ _ _ _ _ _]
      tunnel: w422 -> [_ _ _ _ _ _ _ _ _]
      tunnel: w421 -> [_ _ _ _ _ _ _ _ _]
      tunnel: w420 -> [_ _ _ _ _ _ _ _ _]
      tunnel: w419 -> [_ _ _ _ _ _ _ _ _]
      tunnel: w418 -> [_ _ _ _ _ _ _ _ _]
      tunnel: w417 -> [_ _ _ _ _ _ _ _ _]
      tunnel: w416 -> [_ _ _ _ _ _ _ _ _]
      tunnel: w415 -> [_ _ _ _ _ _ _ _ _]
      event Timeout {
        n114 = event-data() -> ()  [unwired: 1 in, 2 out]
      }
      event "No1Btn": Value Change {
        n115 = event-data() -> ()  [unwired: 1 in, 5 out]
        n116 = property on="选项卡控件Next" class="TabCtl (严格)"("Value"=T2."选项卡 3" ("选项卡控件Next")) -> ()  [unwired: 2 in, 2 out]
      }
      event "No2Btn": Value Change {
        n117 = event-data() -> ()  [unwired: 1 in, 5 out]
        n118 = property on="选项卡控件Next" class="TabCtl (严格)"("Value"=T2."选项卡 4" ("选项卡控件Next")) -> ()  [unwired: 2 in, 2 out]
      }
      event "No3Btn": Value Change {
        n119 = event-data() -> ()  [unwired: 1 in, 5 out]
        n120 = property on="选项卡控件Next" class="TabCtl (严格)"("Value"=T2."选项卡 5" ("选项卡控件Next")) -> ()  [unwired: 2 in, 2 out]
      }
      event "MotinAdv": Value Change {
        n121 = event-data() -> ()  [unwired: 1 in, 5 out]
        n122 = property on="选项卡控件Next" class="TabCtl (严格)"("Value"=T2."选项卡 2" ("选项卡控件Next")) -> ()  [unwired: 2 in, 2 out]
      }
      event "TogReturnBtn": Value Change {
        n123 = event-data() -> ()  [unwired: 1 in, 5 out]
        n124 = property on="选项卡控件Next" class="TabCtl (严格)"("Value"=T6."选项卡 1" ("选项卡控件Next")) -> ()  [unwired: 2 in, 2 out]
      }
      event "Plat3ReturnBtn": Value Change {
        n125 = event-data() -> ()  [unwired: 1 in, 5 out]
        n126 = property on="选项卡控件Next" class="TabCtl (严格)"("Value"=T2."选项卡 1" ("选项卡控件Next")) -> ()  [unwired: 2 in, 2 out]
      }
      event "Plat2ReturnBtn": Value Change {
        n127 = event-data() -> ()  [unwired: 1 in, 5 out]
        n128 = property on="选项卡控件Next" class="TabCtl (严格)"("Value"=T2."选项卡 1" ("选项卡控件Next")) -> ()  [unwired: 2 in, 2 out]
      }
      event "Plat1ReturnBtn": Value Change {
        n129 = event-data() -> ()  [unwired: 1 in, 5 out]
        n130 = property on="选项卡控件Next" class="TabCtl (严格)"("Value"=T2."选项卡 1" ("选项卡控件Next")) -> ()  [unwired: 2 in, 2 out]
      }
    }
  }
  n131 = while {
    tunnel: w8 -> [w447]
    tunnel: w7 -> [w446]
    tunnel: w6 -> [w445]
    tunnel: w5 -> [w444]
    tunnel: w4 -> [w443]
    tunnel: w3 -> [w442]
    tunnel: w1 -> [_]
    stop <- FALSE stop-if-true
    n132 = event shown="[1] \"TogStopBtn\": 值改变" {
      selector: _ -> [_ _]
      dyn-events: _ -> [_ _]
      timeout: _ -> [_ _]
      tunnel: w447 -> [_ w455]
      tunnel: w446 -> [_ w454]
      tunnel: w445 -> [_ w453]
      tunnel: w444 -> [_ w452]
      tunnel: w443 -> [_ w451]
      tunnel: w442 -> [_ w450]
      event Timeout {
        n133 = event-data() -> ()  [unwired: 1 in, 2 out]
      }
      event "TogStopBtn": Value Change {
        n134 = event-data() -> ()  [unwired: 1 in, 5 out]
        n135 = Stop(stop? (T)=TRUE ("停止？(T)")) -> ()
        n136 = Enqueue Element(queue=w451, element=enum16{"平台3机械手已完成放料动作", "NOPE"}."NOPE" ("元素")) -> ()  [unwired: 2 in, 3 out]
        n137 = Enqueue Element(queue=w453, element=enum16{"平台2已回到取料点", "NOPE"}."NOPE" ("元素")) -> ()  [unwired: 2 in, 3 out]
        n138 = Enqueue Element(queue=w454, element=enum16{"平台2已回到接料点", "NOPE"}."NOPE" ("元素")) -> ()  [unwired: 2 in, 3 out]
        n139 = Enqueue Element(queue=w452, element=enum16{"平台3机械手完成取料动作", "NOPE"}."NOPE" ("元素")) -> ()  [unwired: 2 in, 3 out]
        n140 = Enqueue Element(queue=w455, element=enum16{"平台1运动完成", "NOPE"}."NOPE" ("元素")) -> ()  [unwired: 2 in, 3 out]
        n141 = Enqueue Element(queue=w450, element=enum16{"平台3放料机构已回到取料点", "NOPE"}."NOPE" ("元素")) -> ()  [unwired: 2 in, 3 out]
      }
    }
  }
  n142 = while {
    tunnel: w323 -> [_]
    tunnel: w29 -> [w483]
    tunnel: w170 -> [w482]
    tunnel: w33 -> [w481]
    tunnel: w319 -> [w480]
    tunnel: w32 -> [w479]
    tunnel: w318 -> [w478]
    tunnel: w30 -> [w477]
    tunnel: w169 -> [w476]
    tunnel: w31 -> [w475]
    tunnel: w168 -> [w474]
    tunnel: w37 -> [w473]
    tunnel: w165 -> [w472]
    tunnel: w35 -> [w471]
    tunnel: w167 -> [w470]
    tunnel: w34 -> [w469]
    tunnel: w166 -> [w468]
    tunnel: w36 -> [w467]
    tunnel: w311 -> [w466]
    tunnel: w296 -> [_]
    tunnel: w212 -> [_]
    tunnel: w28 -> [w465]
    tunnel: w205 -> [w464]
    tunnel: w27 -> [w463]
    tunnel: w204 -> [w462]
    stop <- FALSE stop-if-true
    n143 = event shown="[2] \"MotorStart\": 值改变" {
      selector: _ -> [_ _ _ _ _ _ _ _ _ _ _ _ _ _]
      dyn-events: _ -> [_ _ _ _ _ _ _ _ _ _ _ _ _ _]
      timeout: _ -> [_ _ _ _ _ _ _ _ _ _ _ _ _ _]
      tunnel: w483 -> [_ w500 w527 w556 w573 w582 w587 _ _ _ _ _ _ w608]
      tunnel: w482 -> [_ w499 w526 w555 w572 w581 w586 _ _ _ _ _ _ w607]
      tunnel: w481 -> [_ w498 _ _ _ _ _ _ _ _ _ _ _ _]
      tunnel: w480 -> [_ w497 _ _ _ _ _ _ _ _ _ _ _ _]
      tunnel: w479 -> [_ w496 _ _ _ _ _ _ _ _ _ _ _ _]
      tunnel: w478 -> [_ w495 _ _ _ _ _ _ _ _ _ _ _ _]
      tunnel: w477 -> [_ _ _ _ w577 _ _ _ _ _ _ _ _ _]
      tunnel: w476 -> [_ _ _ _ w576 _ _ _ _ _ _ _ _ _]
      tunnel: w475 -> [_ _ _ _ w575 _ _ _ _ _ _ _ _ _]
      tunnel: w474 -> [_ _ _ _ w574 _ _ _ _ _ _ _ _ _]
      tunnel: w473 -> [_ _ _ w561 _ _ _ _ _ _ _ _ _ _]
      tunnel: w472 -> [_ _ _ w560 _ _ _ _ _ _ _ _ _ _]
      tunnel: w471 -> [_ _ w525 _ _ _ _ _ _ _ _ _ _ _]
      tunnel: w470 -> [_ _ w524 _ _ _ _ _ _ _ _ _ _ _]
      tunnel: w469 -> [_ _ w523 _ _ _ _ _ _ _ _ _ _ _]
      tunnel: w468 -> [_ _ w522 _ _ _ _ _ _ _ _ _ _ _]
      tunnel: w467 -> [_ _ w521 _ _ _ _ _ _ _ _ _ _ _]
      tunnel: w466 -> [_ _ w520 _ _ _ _ _ _ _ _ _ _ _]
      tunnel: w465 -> [_ _ _ _ _ _ _ _ _ _ _ _ _ w606]
      tunnel: w464 -> [_ _ _ _ _ _ _ _ _ _ _ _ _ w605]
      tunnel: w463 -> [_ _ _ _ _ _ _ _ _ _ _ _ _ w604]
      tunnel: w462 -> [_ _ _ _ _ _ _ _ _ _ _ _ _ w603]
      event Timeout {
        n144 = event-data() -> ()  [unwired: 1 in, 2 out]
      }
      event "SolenAction": Value Change {
        n145 = event-data() -> ()  [unwired: 1 in, 5 out]
        n146 = Flush Queue(queue=w500, error in (no error)=w499) -> (queue out=w491:refnum<queue>)  [unwired: 2 out]
        n147 = Flush Queue(queue=w498, error in (no error)=w497) -> (queue out=w490:refnum<queue>)  [unwired: 2 out]
        n148 = Flush Queue(queue=w496, error in (no error)=w495) -> (queue out=w489:refnum<queue>, error out=w494:errorcluster)  [unwired: 1 out]
        n149 = property on="SolenNum_Event" class="DigNum (严格)"() -> ("Value"=w486:i32)  [unwired: 2 in, 2 out]
        n150 = property on="SolenStatue_Event" class="CmbBox"() -> ("Value"=w488:string)  [unwired: 2 in, 2 out]
        n151 = Decimal String To Number(string=w488) -> (number=w487:i32)  [unwired: 2 in, 1 out]
        n152 = Enqueue Element(queue=w489, element=w487, error in (no error)=w494) -> (error out=w493:errorcluster)  [unwired: 1 in, 2 out]
        n153 = Enqueue Element(queue=w490, element=w486, error in (no error)=w493) -> (error out=w492:errorcluster)  [unwired: 1 in, 2 out]
        n154 = Enqueue Element(queue=w491, element=T7."SolenAction" ("元素"), error in (no error)=w492) -> ()  [unwired: 1 in, 3 out]
      }
      event "MotorStart": Value Change {
        n155 = event-data() -> ()  [unwired: 1 in, 5 out]
        n156 = Flush Queue(queue=w527, error in (no error)=w526) -> (queue out=w512:refnum<queue>)  [unwired: 2 out]
        n157 = Flush Queue(queue=w525, error in (no error)=w524) -> (queue out=w516:refnum<queue>)  [unwired: 2 out]
        n158 = Flush Queue(queue=w523, error in (no error)=w522) -> (queue out=w515:refnum<queue>)  [unwired: 2 out]
        n159 = Flush Queue(queue=w521, error in (no error)=w520) -> (queue out=w514:refnum<queue>, error out=w519:errorcluster)  [unwired: 1 out]
        n160 = property on="Motor1Pos" class="DigNum (严格)"() -> ("Value"=w507:i32)  [unwired: 2 in, 2 out]
        n161 = property on="Motor2Pos" class="DigNum (严格)"() -> ("Value"=w506:i32)  [unwired: 2 in, 2 out]
        n162 = property on="Motor3Pos" class="DigNum (严格)"() -> ("Value"=w505:i32)  [unwired: 2 in, 2 out]
        n163 = property on="Motor4Pos" class="DigNum (严格)"() -> ("Value"=w504:i32)  [unwired: 2 in, 2 out]
        n164 = property on="Motor5Pos" class="DigNum (严格)"() -> ("Value"=w503:i32)  [unwired: 2 in, 2 out]
        n165 = property on="Directon" class="CmbBox"() -> ("Value"=w501:string)  [unwired: 2 in, 2 out]
        n166 = property on="Motor6Pos" class="DigNum (严格)"() -> ("Value"=w502:i32)  [unwired: 2 in, 2 out]
        n167 = property on="StepNum" class="DigNum (严格)"() -> ("Value"=w508:i32)  [unwired: 2 in, 2 out]
        n168 = property on="MotorNum" class="DigNum (严格)"() -> ("Value"=w509:i32)  [unwired: 2 in, 2 out]
        n169 = case shown="1, 默认" w509 {
          tunnel: w508 -> [w530 w534 w537 w540 w545 w548]
          tunnel: w507 -> [w531 _ _ _ _ _]
          tunnel: w506 -> [_ w533 _ _ _ _]
          tunnel: w505 -> [_ _ w536 _ _ _]
          tunnel: w504 -> [_ _ _ w541 _ _]
          tunnel: w503 -> [_ _ _ _ w546 _]
          tunnel: w502 -> [_ _ _ _ _ w549]
          tunnel: w501 -> [w529 w535 w539 w543 w547 w551]
          frame 1, Default {
            n170 = call "calcupposfunc.vi"("Step"=w530, "Pos"=w531, "Directon"=w529) -> ("Pos_Out"=w528:i32)  [unwired: 8 in]
            n171 = property on="Motor1Pos" class="DigNum (严格)"("Value"=w528) -> ()  [unwired: 2 in, 2 out]
          }
          frame 2 {
            n172 = call "calcupposfunc.vi"("Step"=w534, "Pos"=w533, "Directon"=w535) -> ("Pos_Out"=w532:i32)  [unwired: 8 in]
            n173 = property on="Motor2Pos" class="DigNum (严格)"("Value"=w532) -> ()  [unwired: 2 in, 2 out]
          }
          frame 3 {
            n174 = call "calcupposfunc.vi"("Step"=w537, "Pos"=w536, "Directon"=w539) -> ("Pos_Out"=w538:i32)  [unwired: 8 in]
            n175 = property on="Motor3Pos" class="DigNum (严格)"("Value"=w538) -> ()  [unwired: 2 in, 2 out]
          }
          frame 4 {
            n176 = call "calcupposfunc.vi"("Step"=w540, "Pos"=w541, "Directon"=w543) -> ("Pos_Out"=w542:i32)  [unwired: 8 in]
            n177 = property on="Motor4Pos" class="DigNum (严格)"("Value"=w542) -> ()  [unwired: 2 in, 2 out]
          }
          frame 5 {
            n178 = call "calcupposfunc.vi"("Step"=w545, "Pos"=w546, "Directon"=w547) -> ("Pos_Out"=w544:i32)  [unwired: 8 in]
            n179 = property on="Motor5Pos" class="DigNum (严格)"("Value"=w544) -> ()  [unwired: 2 in, 2 out]
          }
          frame 6 {
            n180 = call "calcupposfunc.vi"("Step"=w548, "Pos"=w549, "Directon"=w551) -> ("Pos_Out"=w550:i32)  [unwired: 8 in]
            n181 = property on="Motor6Pos" class="DigNum (严格)"("Value"=w550) -> ()  [unwired: 2 in, 2 out]
          }
        }
        n182 = Enqueue Element(queue=w514, element=w509, error in (no error)=w519) -> (error out=w518:errorcluster)  [unwired: 1 in, 2 out]
        n183 = Decimal String To Number(string=w501) -> (number=w511:i32)  [unwired: 2 in, 1 out]
        n184 = Enqueue Element(queue=w515, element=w511, error in (no error)=w518) -> (error out=w517:errorcluster)  [unwired: 1 in, 2 out]
        n185 = Enqueue Element(queue=w516, element=w508, error in (no error)=w517) -> (error out=w513:errorcluster)  [unwired: 1 in, 2 out]
        n186 = Enqueue Element(queue=w512, element=T7."MotorStart" ("元素"), error in (no error)=w513) -> ()  [unwired: 1 in, 3 out]
      }
      event "MotorStop": Value Change {
        n187 = event-data() -> ()  [unwired: 1 in, 5 out]
        n188 = Flush Queue(queue=w556, error in (no error)=w555) -> (queue out=w554:refnum<queue>)  [unwired: 2 out]
        n189 = Flush Queue(queue=w561, error in (no error)=w560) -> (queue out=w559:refnum<queue>, error out=w558:errorcluster)  [unwired: 1 out]
        n190 = property on="StopMotorNum" class="DigNum (严格)"() -> ("Value"=w557:i32)  [unwired: 2 in, 2 out]
        n191 = Enqueue Element(queue=w559, element=w557, error in (no error)=w558) -> (error out=w553:errorcluster)  [unwired: 1 in, 2 out]
        n192 = Enqueue Element(queue=w554, element=T7."MotorStop" ("元素"), error in (no error)=w553) -> ()  [unwired: 1 in, 3 out]
      }
      event "SolenAdvance": Value Change {
        n193 = event-data() -> ()  [unwired: 1 in, 5 out]
        n194 = Flush Queue(queue=w573, error in (no error)=w572) -> (queue out=w568:refnum<queue>)  [unwired: 2 out]
        n195 = Flush Queue(queue=w577, error in (no error)=w576) -> (queue out=w567:refnum<queue>)  [unwired: 2 out]
        n196 = Flush Queue(queue=w575, error in (no error)=w574) -> (queue out=w566:refnum<queue>, error out=w571:errorcluster)  [unwired: 1 out]
        n197 = property on="SolenPlat_Event" class="DigNum (严格)"() -> ("Value"=w565:i32)  [unwired: 2 in, 2 out]
        n198 = property on="SolenPlatStatue_Event" class="CmbBox"() -> ("Value"=w564:string)  [unwired: 2 in, 2 out]
        n199 = Decimal String To Number(string=w564) -> (number=w563:i32)  [unwired: 2 in, 1 out]
        n200 = Enqueue Element(queue=w566, element=w563, error in (no error)=w571) -> (error out=w570:errorcluster)  [unwired: 1 in, 2 out]
        n201 = Enqueue Element(queue=w567, element=w565, error in (no error)=w570) -> (error out=w569:errorcluster)  [unwired: 1 in, 2 out]
        n202 = Enqueue Element(queue=w568, element=T7."SolenAdv" ("元素"), error in (no error)=w569) -> ()  [unwired: 1 in, 3 out]
      }
      event "FeedMotorStart": Value Change {
        n203 = event-data() -> ()  [unwired: 1 in, 5 out]
        n204 = Flush Queue(queue=w582, error in (no error)=w581) -> (queue out=w580:refnum<queue>, error out=w579:errorcluster)  [unwired: 1 out]
        n205 = Enqueue Element(queue=w580, element=T7."FeedMotorStart" ("元素"), error in (no error)=w579) -> ()  [unwired: 1 in, 3 out]
      }
      event "FeedMotorStop": Value Change {
        n206 = event-data() -> ()  [unwired: 1 in, 5 out]
        n207 = Flush Queue(queue=w587, error in (no error)=w586) -> (queue out=w585:refnum<queue>, error out=w584:errorcluster)  [unwired: 1 out]
        n208 = Enqueue Element(queue=w585, element=T7."FeedMotorStop" ("元素"), error in (no error)=w584) -> ()  [unwired: 1 in, 3 out]
      }
      event "ClearPos1": Value Change {
        n209 = event-data() -> ()  [unwired: 1 in, 5 out]
        n210 = property on="Motor1Pos" class="DigNum (严格)"("Value"=0 ("Motor1Pos")) -> ()  [unwired: 2 in, 2 out]
      }
      event "ClearPos2": Value Change {
        n211 = event-data() -> ()  [unwired: 1 in, 5 out]
        n212 = property on="Motor2Pos" class="DigNum (严格)"("Value"=0 ("Motor2Pos")) -> ()  [unwired: 2 in, 2 out]
      }
      event "ClearPos3": Value Change {
        n213 = event-data() -> ()  [unwired: 1 in, 5 out]
        n214 = property on="Motor3Pos" class="DigNum (严格)"("Value"=0 ("Motor3Pos")) -> ()  [unwired: 2 in, 2 out]
      }
      event "ClearPos4": Value Change {
        n215 = event-data() -> ()  [unwired: 1 in, 5 out]
        n216 = property on="Motor4Pos" class="DigNum (严格)"("Value"=0 ("Motor4Pos")) -> ()  [unwired: 2 in, 2 out]
      }
      event "ClearPos5": Value Change {
        n217 = event-data() -> ()  [unwired: 1 in, 5 out]
        n218 = property on="Motor5Pos" class="DigNum (严格)"("Value"=0 ("Motor5Pos")) -> ()  [unwired: 2 in, 2 out]
      }
      event "ClearPos6": Value Change {
        n219 = event-data() -> ()  [unwired: 1 in, 5 out]
        n220 = property on="Motor6Pos" class="DigNum (严格)"("Value"=0 ("Motor6Pos")) -> ()  [unwired: 2 in, 2 out]
      }
      event "SetMotorSpeed": Value Change {
        n221 = event-data() -> ()  [unwired: 1 in, 5 out]
        n222 = Flush Queue(queue=w608, error in (no error)=w607) -> (queue out=w598:refnum<queue>)  [unwired: 2 out]
        n223 = Flush Queue(queue=w604, error in (no error)=w603) -> (queue out=w600:refnum<queue>)  [unwired: 2 out]
        n224 = Flush Queue(queue=w606, error in (no error)=w605) -> (queue out=w602:refnum<queue>, error out=w601:errorcluster)  [unwired: 1 out]
        n225 = property on="MotorSpeed" class="DigNum (严格)"() -> ("Value"=w595:i32)  [unwired: 2 in, 2 out]
        n226 = property on="MotorSpeedNum" class="DigNum (严格)"() -> ("Value"=w596:i32)  [unwired: 2 in, 2 out]
        n227 = Enqueue Element(queue=w602, element=w596, error in (no error)=w601) -> (error out=w599:errorcluster)  [unwired: 1 in, 2 out]
        n228 = Enqueue Element(queue=w600, element=w595, error in (no error)=w599) -> (error out=w597:errorcluster)  [unwired: 1 in, 2 out]
        n229 = Enqueue Element(queue=w598, element=T8."SetMotorSpeed" ("元素"), error in (no error)=w597) -> ()  [unwired: 1 in, 3 out]
      }
    }
  }
  n230 = while {
    tunnel: w29 -> [w631]
    tunnel: w170 -> [w632]
    tunnel: w35 -> [w630]
    tunnel: w167 -> [w629]
    tunnel: w34 -> [w628]
    tunnel: w166 -> [w627]
    tunnel: w36 -> [w626]
    tunnel: w311 -> [w625]
    tunnel: w33 -> [w624]
    tunnel: w319 -> [w623]
    tunnel: w32 -> [w622]
    tunnel: w318 -> [w621]
    tunnel: w30 -> [w620]
    tunnel: w169 -> [w619]
    tunnel: w31 -> [w618]
    tunnel: w168 -> [w617]
    tunnel: w37 -> [w616]
    tunnel: w165 -> [w615]
    tunnel: w28 -> [w614]
    tunnel: w205 -> [w613]
    tunnel: w27 -> [w612]
    tunnel: w204 -> [w611]
    tunnel: w26 -> [w610]
    tunnel: w139 -> [w609]
    stop <- FALSE stop-if-true
    n231 = event shown="[1] \"start\": 值改变" {
      selector: _ -> [_ _]
      dyn-events: _ -> [_ _]
      timeout: _ -> [_ _]
      tunnel: w632 -> [_ w657]
      tunnel: w631 -> [_ w656]
      tunnel: w630 -> [_ w655]
      tunnel: w629 -> [_ w654]
      tunnel: w628 -> [_ w653]
      tunnel: w627 -> [_ w652]
      tunnel: w626 -> [_ w651]
      tunnel: w625 -> [_ w650]
      tunnel: w624 -> [_ w649]
      tunnel: w623 -> [_ w648]
      tunnel: w622 -> [_ w647]
      tunnel: w621 -> [_ w646]
      tunnel: w620 -> [_ w645]
      tunnel: w619 -> [_ w644]
      tunnel: w618 -> [_ w643]
      tunnel: w617 -> [_ w642]
      tunnel: w616 -> [_ w641]
      tunnel: w615 -> [_ w640]
      tunnel: w614 -> [_ w639]
      tunnel: w613 -> [_ w638]
      tunnel: w612 -> [_ w637]
      tunnel: w611 -> [_ w636]
      tunnel: w610 -> [_ w635]
      tunnel: w609 -> [_ w634]
      event Timeout {
        n232 = event-data() -> ()  [unwired: 1 in, 2 out]
      }
      event "start": Value Change {
        n233 = event-data() -> ()  [unwired: 1 in, 5 out]
        n234 = while {
          tunnel: w657 -> [w680]
          tunnel: w656 -> [w681]
          tunnel: w655 -> [w675]
          tunnel: w654 -> [w674]
          tunnel: w653 -> [w677]
          tunnel: w652 -> [w676]
          tunnel: w651 -> [w679]
          tunnel: w650 -> [w678]
          tunnel: w649 -> [w673]
          tunnel: w648 -> [w672]
          tunnel: w647 -> [w671]
          tunnel: w646 -> [w670]
          tunnel: w645 -> [w669]
          tunnel: w644 -> [w668]
          tunnel: w643 -> [w667]
          tunnel: w642 -> [w666]
          tunnel: w641 -> [w665]
          tunnel: w640 -> [w664]
          tunnel: w639 -> [w663]
          tunnel: w638 -> [w662]
          tunnel: w637 -> [w661]
          tunnel: w636 -> [w660]
          tunnel: w635 -> [w659]
          tunnel: w634 -> [w658]
          stop <- w684 stop-if-true
          n235 = Dequeue Element(queue=w681, error in (no error)=w680) -> (queue out=w682:refnum<queue>, element=w685:T4, error out=w683:errorcluster)  [unwired: 1 in, 1 out]
          n236 = case shown="无错误" w683 {
            selector: w683 -> [w714 _]
            tunnel: w685 -> [w716 _]
            tunnel: [w694 TRUE] -> w684
            tunnel: w682 -> [w715 _]
            tunnel: w679 -> [w711 _]
            tunnel: w678 -> [w710 _]
            tunnel: w677 -> [w709 _]
            tunnel: w676 -> [w708 _]
            tunnel: w675 -> [w707 _]
            tunnel: w674 -> [w706 _]
            tunnel: w673 -> [w705 _]
            tunnel: w672 -> [w704 _]
            tunnel: w671 -> [w703 _]
            tunnel: w670 -> [w702 _]
            tunnel: w669 -> [w701 _]
            tunnel: w668 -> [w700 _]
            tunnel: w667 -> [w699 _]
            tunnel: w666 -> [w698 _]
            tunnel: w665 -> [w693 _]
            tunnel: w664 -> [w692 _]
            tunnel: w663 -> [w691 _]
            tunnel: w662 -> [w689 _]
            tunnel: w661 -> [w690 _]
            tunnel: w660 -> [w688 _]
            tunnel: w659 -> [w687 _]
            tunnel: w658 -> [w686 _]
            frame No Error {
              n237 = case shown="\"SetMotorSpeed\"" w716 {
                tunnel: w711 -> [_ _ _ _ _ _ _ _ w809 _ _ _ _ _ _ _]
                tunnel: w710 -> [_ _ _ _ _ _ _ _ w808 _ _ _ _ _ _ _]
                tunnel: w709 -> [_ _ _ _ _ _ _ _ w812 _ _ _ _ _ _ _]
                tunnel: w708 -> [_ _ _ _ _ _ _ _ w811 _ _ _ _ _ _ _]
                tunnel: w707 -> [_ _ _ _ _ _ _ _ w815 _ _ _ _ _ _ _]
                tunnel: w706 -> [_ _ _ _ _ _ _ _ w814 _ _ _ _ _ _ _]
                tunnel: w705 -> [_ _ _ _ _ _ _ _ _ _ _ w824 _ _ _ _]
                tunnel: w704 -> [_ _ _ _ _ _ _ _ _ _ _ w823 _ _ _ _]
                tunnel: w703 -> [_ _ _ _ _ _ _ _ _ _ _ w822 _ _ _ _]
                tunnel: w702 -> [_ _ _ _ _ _ _ _ _ _ _ w821 _ _ _ _]
                tunnel: w701 -> [_ _ _ _ _ _ _ _ _ _ _ _ w830 _ _ _]
                tunnel: w700 -> [_ _ _ _ _ _ _ _ _ _ _ _ w829 _ _ _]
                tunnel: w699 -> [_ _ _ _ _ _ _ _ _ _ _ _ w828 _ _ _]
                tunnel: w698 -> [_ _ _ _ _ _ _ _ _ _ _ _ w827 _ _ _]
                tunnel: w693 -> [_ _ _ _ _ _ _ _ _ _ w818 _ _ _ _ _]
                tunnel: w692 -> [_ _ _ _ _ _ _ _ _ _ w817 _ _ _ _ _]
                tunnel: w691 -> [_ _ _ _ _ _ _ _ _ _ _ _ _ _ w841 _]
                tunnel: w690 -> [_ _ _ _ _ _ _ _ _ _ _ _ _ _ w839 _]
                tunnel: w689 -> [_ _ _ _ _ _ _ _ _ _ _ _ _ _ w840 _]
                tunnel: w688 -> [_ _ _ _ _ _ _ _ _ _ _ _ _ _ w838 _]
                tunnel: w687 -> [_ _ _ _ _ _ _ _ _ _ _ _ _ _ _ w844]
                tunnel: w686 -> [_ _ _ _ _ _ _ _ _ _ _ _ _ _ _ w843]
                frame "None", Default {
                }
                frame "GetSensorStatue" {
                  n238 = Initialize Array(0 ("元素"), 8 ("维数大小")) -> (w719:i32[])
                  n239 = call "API get Sensor Statue.vi"("array input"=w719) -> ("array output"=w725:i32[])  [unwired: 9 in, 1 out]
                  "Sensor array output" <- w725
                  n240 = Index Array(array=w725, index=2 ("索引")) -> (element=w733:i32)
                  n241 = Index Array(array=w725, index=1 ("索引")) -> (element=w732:i32)
                  n242 = Index Array(array=w725, index=4 ("索引")) -> (element=w734:i32)
                  n243 = Index Array(array=w725, index=5 ("索引")) -> (element=w735:i32)
                  n244 = Index Array(array=w725, index=3 ("索引")) -> (element=w736:i32)
                  n245 = property on="红外电平" class="DigNum (严格)"("Value"=w733) -> ()  [unwired: 2 in, 2 out]
                  n246 = property on="电涡流电平" class="DigNum (严格)"("Value"=w732) -> ()  [unwired: 2 in, 2 out]
                  n247 = property on="电容1" class="DigNum (严格)"("Value"=w734) -> ()  [unwired: 2 in, 2 out]
                  n248 = property on="电容2" class="DigNum (严格)"("Value"=w735) -> ()  [unwired: 2 in, 2 out]
                  n249 = property on="电容3" class="DigNum (严格)"("Value"=w736) -> ()  [unwired: 2 in, 2 out]
                  n250 = Merge Signals(w732) -> (w731:dynamicdata)
                  n251 = Merge Signals(w733) -> (w730:dynamicdata)
                  n252 = Merge Signals(w734) -> (w726:dynamicdata)
                  n253 = Merge Signals(w735) -> (w728:dynamicdata)
                  n254 = Merge Signals(w736) -> (w727:dynamicdata)
                  n255 = Merge Signals(w730, w731, w726, w728, w727) -> (→"Waveform Chart":dynamicdata)
                }
                frame "GetSensorAD" {
                  n256 = call "API get Sensor AD.vi"("SensorADValueIN"=0.0) -> ("SensorADValueOut"=w737:dbl)  [unwired: 3 in, 1 out]
                  n257 = property on="电桥电平" class="DigNum (严格)"("Value"=w737) -> ()  [unwired: 2 in, 2 out]
                  n258 = property on="电桥电平_Event" class="DigNum (严格)"("Value"=w737) -> ()  [unwired: 2 in, 2 out]
                }
                frame "GetSolenStatue" {
                  n259 = Initialize Array(0 ("元素"), 48 ("维数大小")) -> (w740:i32[])
                  n260 = call "API get solen statue.vi"("solenstatue input"=w740) -> ("solenstatue output"=w739:i32[])  [unwired: 10 in]
                  "solenstatue output" <- w739
                  n261 = for {
                    tunnel: w739 -> [w746] mode=indexing
                    i -> [w749]
                    n262 = Not Equal To 0?(x=w746) -> (x != 0?=w747:bool)
                    n263 = Increment(x=w749) -> (x+1=w751:i32)
                    n264 = Number To Decimal String(number=w751) -> (decimal integer string=w750:string)  [unwired: 1 in]
                    n265 = To Variant(anything=w747) -> (Variant=w744:variant)
                    n266 = Concatenate Strings("Solen" ("字符串"), w750) -> (w743:string)
                    n267 = control-ref of="本VI"() -> (w745:refnum<vi>)
                    n268 = invoke class="VI" method="Ctrl Val.Set"(reference=w745, "Control Name"=w743, "Value"=w744) -> ()  [unwired: 2 in, 5 out]
                  }
                }
                frame "GetPaltformStatue" {
                  n269 = Initialize Array(0 ("元素"), 8 ("维数大小")) -> (w760:i32[])
                  n270 = Initialize Array(0 ("元素"), 8 ("维数大小")) -> (w758:i32[])
                  n271 = Initialize Array(0 ("元素"), 8 ("维数大小")) -> (w763:i32[])
                  n272 = call "API get platform statue.vi"("platformStatue input"=w760, "PlatformNum"=2) -> ("platformStatue output"=w754:i32[])  [unwired: 8 in, 1 out]
                  "platformStatue2 output" <- w754
                  n273 = call "API get platform statue.vi"("platformStatue input"=w758, "PlatformNum"=1) -> ("platformStatue output"=w753:i32[])  [unwired: 8 in, 1 out]
                  "platformStatue1 output" <- w753
                  n274 = call "API get platform statue.vi"("platformStatue input"=w763, "PlatformNum"=0) -> ("platformStatue output"=w752:i32[])  [unwired: 8 in, 1 out]
                  "platformStatue0 output" <- w752
                  n275 = for {
                    tunnel: w754 -> [w788] mode=indexing
                    i -> [w791]
                    n276 = Not Equal To 0?(x=w788) -> (x != 0?=w789:bool)
                    n277 = Increment(x=w791) -> (x+1=w793:i32)
                    n278 = Number To Decimal String(number=w793) -> (decimal integer string=w792:string)  [unwired: 1 in]
                    n279 = To Variant(anything=w789) -> (Variant=w786:variant)
                    n280 = Concatenate Strings("Plat3IO" ("字符串"), w792) -> (w785:string)
                    n281 = control-ref of="本VI"() -> (w787:refnum<vi>)
                    n282 = invoke class="VI" method="Ctrl Val.Set"(reference=w787, "Control Name"=w785, "Value"=w786) -> ()  [unwired: 2 in, 5 out]
                  }
                  n283 = for {
                    tunnel: w753 -> [w779] mode=indexing
                    i -> [w782]
                    n284 = Not Equal To 0?(x=w779) -> (x != 0?=w780:bool)
                    n285 = Increment(x=w782) -> (x+1=w784:i32)
                    n286 = Number To Decimal String(number=w784) -> (decimal integer string=w783:string)  [unwired: 1 in]
                    n287 = To Variant(anything=w780) -> (Variant=w777:variant)
                    n288 = Concatenate Strings("Plat2IO" ("字符串"), w783) -> (w776:string)
                    n289 = control-ref of="本VI"() -> (w778:refnum<vi>)
                    n290 = invoke class="VI" method="Ctrl Val.Set"(reference=w778, "Control Name"=w776, "Value"=w777) -> ()  [unwired: 2 in, 5 out]
                  }
                  n291 = for {
                    tunnel: w752 -> [w770] mode=indexing
                    i -> [w773]
                    n292 = Not Equal To 0?(x=w770) -> (x != 0?=w771:bool)
                    n293 = Increment(x=w773) -> (x+1=w775:i32)
                    n294 = Number To Decimal String(number=w775) -> (decimal integer string=w774:string)  [unwired: 1 in]
                    n295 = To Variant(anything=w771) -> (Variant=w768:variant)
                    n296 = Concatenate Strings("Plat1IO" ("字符串"), w774) -> (w767:string)
                    n297 = control-ref of="本VI"() -> (w769:refnum<vi>)
                    n298 = invoke class="VI" method="Ctrl Val.Set"(reference=w769, "Control Name"=w767, "Value"=w768) -> ()  [unwired: 2 in, 5 out]
                  }
                }
                frame "GetMotorStatue" {
                  n299 = Initialize Array(0 ("元素"), 6 ("维数大小")) -> (w797:i32[])
                  n300 = call "API get motor statue.vi"("motor statue array input"=w797) -> ("motor statue array output"=w794:i32[])  [unwired: 9 in, 1 out]
                  "motor statue array output" <- w794
                  n301 = for {
                    tunnel: w794 -> [w801] mode=indexing
                    i -> [w804]
                    n302 = Not Equal To 0?(x=w801) -> (x != 0?=w802:bool)
                    n303 = Increment(x=w804) -> (x+1=w806:i32)
                    n304 = Number To Decimal String(number=w806) -> (decimal integer string=w805:string)  [unwired: 1 in]
                    n305 = To Variant(anything=w802) -> (Variant=w799:variant)
                    n306 = Concatenate Strings("M" ("字符串"), w805) -> (w798:string)
                    n307 = control-ref of="本VI"() -> (w800:refnum<vi>)
                    n308 = invoke class="VI" method="Ctrl Val.Set"(reference=w800, "Control Name"=w798, "Value"=w799) -> ()  [unwired: 2 in, 5 out]
                  }
                }
                frame "FeedMotorStart" {
                  n309 = call "API Feed Motor START.vi"() -> ()  [unwired: 11 in, 1 out]
                }
                frame "FeedMotorStop" {
                  n310 = call "API Feed Motor Stop.vi"() -> ()  [unwired: 11 in, 1 out]
                }
                frame "MotorStart" {
                  n311 = Dequeue Element(queue=w809, error in (no error)=w808) -> (element=w807:i32)  [unwired: 1 in, 3 out]
                  n312 = Dequeue Element(queue=w812, error in (no error)=w811) -> (element=w810:i32)  [unwired: 1 in, 3 out]
                  n313 = Dequeue Element(queue=w815, error in (no error)=w814) -> (element=w813:i32)  [unwired: 1 in, 3 out]
                  n314 = call "API Motor Start.vi"("stepNum"=w813, "direction"=w810, "motorNum"=w807) -> ()  [unwired: 8 in, 1 out]
                }
                frame "MotorRestart" {
                }
                frame "MotorStop" {
                  n315 = Dequeue Element(queue=w818, error in (no error)=w817) -> (element=w816:i32)  [unwired: 1 in, 3 out]
                  n316 = call "API Motor Stop.vi"("motorNum"=w816) -> ()  [unwired: 10 in, 1 out]
                }
                frame "SolenAction" {
                  n317 = Dequeue Element(queue=w824, error in (no error)=w823) -> (element=w820:i32)  [unwired: 1 in, 3 out]
                  n318 = Dequeue Element(queue=w822, error in (no error)=w821) -> (element=w819:i32)  [unwired: 1 in, 3 out]
                  n319 = call "API Solen Action.vi"("statue"=w819, "solenNum"=w820) -> ()  [unwired: 9 in, 1 out]
                }
                frame "SolenAdv" {
                  n320 = Dequeue Element(queue=w830, error in (no error)=w829) -> (element=w826:i32)  [unwired: 1 in, 3 out]
                  n321 = Dequeue Element(queue=w828, error in (no error)=w827) -> (element=w825:i32)  [unwired: 1 in, 3 out]
                  n322 = call "API Solen Advance.vi"("statue"=w825, "platformNum"=w826) -> ()  [unwired: 9 in, 1 out]
                }
                frame "RcvDataInit" {
                  n323 = call "API Rcv Data Init.vi"() -> ()  [unwired: 2 in, 2 out]
                }
                frame "SetMotorSpeed" {
                  n324 = Dequeue Element(queue=w841, error in (no error)=w840) -> (element=w837:i32)  [unwired: 1 in, 3 out]
                  n325 = Dequeue Element(queue=w839, error in (no error)=w838) -> (element=w835:i32)  [unwired: 1 in, 3 out]
                  n326 = Multiply(x=2, y=w835) -> (x*y=w833:i32)
                  n327 = Divide(x=6000000, y=w833) -> (x/y=w832:dbl)
                  n328 = To Long Integer(number=w832) -> (32bit integer=w831:i32)
                  n329 = call "API Set Motor Speed.vi"("motorSpeed"=w831, "motorNum"=w837) -> ()  [unwired: 9 in, 1 out]
                }
                frame "Delay" {
                  n330 = Dequeue Element(queue=w844, error in (no error)=w843) -> (element=w842:u32)  [unwired: 1 in, 3 out]
                  n331 = Wait (ms)(milliseconds to wait=w842) -> ()  [unwired: 1 out]
                }
              }
              n332 = Get Queue Status(queue=w715, error in (no error)=w714) -> (# elements in queue=w697:i32)  [unwired: 1 in, 7 out]
              "指令数" <- w697
              n333 = local read "stop"() -> (w712:bool)
              n334 = And(x=w712, y=TRUE) -> (x .and. y?=w696:bool)
              n335 = Equal To 0?(x=w697) -> (x = 0?=w695:bool)
              n336 = And(x=w696, y=w695) -> (x .and. y?=w694:bool)
            }
            frame Error {
            }
          }
        }
      }
    }
  }
  n337 = while "Plat3-While循环" {
    tunnel: w29 -> [w869]
    tunnel: w30 -> [w867]
    tunnel: w170 -> [w868]
    tunnel: w169 -> [w866]
    tunnel: w31 -> [w865]
    tunnel: w168 -> [w864]
    tunnel: w36 -> [w863]
    tunnel: w165 -> [w862]
    tunnel: w35 -> [w861]
    tunnel: w167 -> [w860]
    tunnel: w34 -> [w859]
    tunnel: w166 -> [w858]
    tunnel: w37 -> [w857]
    tunnel: w33 -> [w856]
    tunnel: w32 -> [w855]
    tunnel: w9 -> [w853]
    tunnel: w10 -> [w852]
    tunnel: w26 -> [w851]
    tunnel: w139 -> [w850]
    tunnel: w27 -> [w848]
    tunnel: w28 -> [w849]
    tunnel: w43 -> [w846]
    tunnel: w42 -> [w847]
    tunnel: w39 -> [_]
    tunnel: w38 -> [_]
    stop <- FALSE stop-if-true
    n338 = event shown="[2] \"Plat3GetMegBtn\": 值改变" {
      selector: _ -> [_ _ _ _ _]
      dyn-events: _ -> [_ _ _ _ _]
      timeout: _ -> [_ _ _ _ _]
      tunnel: w869 -> [_ w969 w1333 w1703 w2083]
      tunnel: w868 -> [_ w968 w1332 _ w2082]
      tunnel: w867 -> [_ w967 w1331 w1704 w2077]
      tunnel: w866 -> [_ w966 w1330 _ _]
      tunnel: w865 -> [_ w948 w1312 w1700 w2076]
      tunnel: w864 -> [_ w947 w1311 _ _]
      tunnel: w863 -> [_ w964 w1328 w1707 _]
      tunnel: w862 -> [_ w963 w1327 _ _]
      tunnel: w861 -> [_ w962 w1326 w1706 _]
      tunnel: w860 -> [_ w961 w1325 _ _]
      tunnel: w859 -> [_ w960 w1324 w1705 _]
      tunnel: w858 -> [_ w959 w1323 _ _]
      tunnel: w857 -> [_ _ _ w1711 w2081]
      tunnel: w856 -> [_ w924 w1288 w1702 _]
      tunnel: w855 -> [_ w923 w1287 w1701 _]
      tunnel: w853 -> [_ w920 w1284 w1610 _]
      tunnel: w852 -> [_ w919 w1283 w1611 _]
      tunnel: w851 -> [_ w894 w1258 w1710 _]
      tunnel: w850 -> [_ w893 w1257 _ _]
      tunnel: w849 -> [_ w873 w1237 w1709 _]
      tunnel: w848 -> [_ w872 w1236 w1708 _]
      tunnel: w847 -> [_ _ _ w1606 _]
      tunnel: w846 -> [_ _ _ w1604 _]
      event Timeout {
        n339 = event-data() -> ()  [unwired: 1 in, 2 out]
      }
      event "Plat3Btn": Value Change {
        n340 = event-data() -> ()  [unwired: 1 in, 5 out]
        n341 = Flush Queue(queue=w964, error in (no error)=w963) -> (queue out=w941:refnum<queue>)  [unwired: 2 out]
        n342 = Flush Queue(queue=w962, error in (no error)=w961) -> (queue out=w940:refnum<queue>)  [unwired: 2 out]
        n343 = Flush Queue(queue=w960, error in (no error)=w959) -> (queue out=w939:refnum<queue>)  [unwired: 2 out]
        n344 = Flush Queue(queue=w967, error in (no error)=w966) -> (queue out=w927:refnum<queue>)  [unwired: 2 out]
        n345 = Flush Queue(queue=w969, error in (no error)=w968) -> (queue out=w899:refnum<queue>)  [unwired: 2 out]
        n346 = Flush Queue(queue=w894, error in (no error)=w893) -> (queue out=w892:refnum<queue>)  [unwired: 2 out]
        n347 = Flush Queue(queue=w873) -> (queue out=w871:refnum<queue>)  [unwired: 1 in, 2 out]
        n348 = Flush Queue(queue=w872) -> (queue out=w870:refnum<queue>)  [unwired: 1 in, 2 out]
        n349 = Flush Queue(queue=w924) -> (queue out=w904:refnum<queue>)  [unwired: 1 in, 2 out]
        n350 = Flush Queue(queue=w923) -> (queue out=w903:refnum<queue>)  [unwired: 1 in, 2 out]
        n351 = Flush Queue(queue=w948, error in (no error)=w947) -> (queue out=w926:refnum<queue>, error out=w905:errorcluster)  [unwired: 1 out]
        n352 = control-ref of="ComboPolicy"() -> (w912:refnum<vi>)
        n353 = control-ref of="CurrentPosX"() -> (w918:refnum<vi>)
        n354 = control-ref of="CurrentPosY"() -> (w913:refnum<vi>)
        n355 = control-ref of="Plat3StopBtn"() -> (w876:refnum<vi>)
        n356 = control-ref of="SelectPolicy"() -> (w874:refnum<vi>)
        n357 = property class="CmbBox"(reference=w912) -> ("Value"=w911:string)  [unwired: 1 in, 2 out]
        n358 = call "QueueSolenAct.vi"("SolenNum_IN"=w904, "SolenStatue_IN"=w903, "SolenNum_Value"=32, "SolenStatue_Value"=1, "错误输入（无错误）"=w905) -> ("SolenNum_OUT"=w887:refnum<queue>, "SolenStatue_OUT"=w885:refnum<queue>, "错误输出"=w900:errorcluster)  [unwired: 8 in]
        n359 = control-ref of="solenstatue output"() -> (w922:refnum<vi>)
        n360 = Decimal String To Number(string=w911) -> (number=w910:i32)  [unwired: 2 in, 1 out]
        n361 = Enqueue Element(queue=w899, element=T8."SolenAction" ("元素"), error in (no error)=w900) -> (queue out=w891:refnum<queue>, error out=w897:errorcluster)  [unwired: 1 in, 1 out]
        n362 = control-ref of="platformStatue2 output"() -> (w875:refnum<vi>)
        n363 = control-ref of="motor statue array output"() -> (w907:refnum<vi>)
        n364 = call "Check.vi"("错误输入（无错误）"=w897, "长度"=1, "索引"=7, "Array引用"=w875, "Bool引用"=w876) -> ("错误输出"=w889:errorcluster)  [unwired: 6 in]
        n365 = call "QueueSolenAct.vi"("SolenNum_IN"=w887, "SolenStatue_IN"=w885, "SolenNum_Value"=36, "SolenStatue_Value"=1, "错误输入（无错误）"=w889) -> ("SolenNum_OUT"=w886:refnum<queue>, "SolenStatue_OUT"=w884:refnum<queue>, "错误输出"=w888:errorcluster)  [unwired: 8 in]
        n366 = Enqueue Element(queue=w891, element=T4."SolenAction" ("元素"), error in (no error)=w888) -> (queue out=w890:refnum<queue>, error out=w880:errorcluster)  [unwired: 1 in, 1 out]
        n367 = call "Check.vi"("错误输入（无错误）"=w880, "长度"=1, "索引"=4, "Array引用"=w875, "Bool引用"=w876) -> ("错误输出"=w879:errorcluster)  [unwired: 6 in]
        n368 = call "QueueSolenAdv.vi"("Statue_IN"=w926, "PlatNum_IN"=w927, "Statue_Value"=0 ("元素"), "PlatNum_Value"=2 ("元素"), "错误输入（无错误）"=w879) -> ("错误输出"=w925:errorcluster)  [unwired: 8 in, 2 out]
        n369 = Enqueue Element(queue=w890, element=T8."SolenAdv" ("元素"), error in (no error)=w925) -> (queue out=w952:refnum<queue>, error out=w955:errorcluster)  [unwired: 1 in, 1 out]
        n370 = call "Check.vi"("错误输入（无错误）"=w955, "长度"=16, "索引"=32, "Array引用"=w922, "Bool引用"=w876) -> ("错误输出"=w945:errorcluster)  [unwired: 6 in]
        n371 = call "QueueMotorStart.vi"("MotorNum"=w941, "Step"=w940, "Direction"=w939, "错误输入（无错误）"=w945, "MotorNum_Int"=5 ("元素"), "Step_Int"=20000 ("元素"), "Direction_Int"=0 ("元素")) -> ("MotorNum_OUT"=w935:refnum<queue>, "Step_OUT"=w934:refnum<queue>, "Direction_OUT"=w933:refnum<queue>, "错误输出"=w938:errorcluster)  [unwired: 9 in]
        n372 = Enqueue Element(queue=w952, element=T8."MotorStart" ("元素"), error in (no error)=w938) -> (queue out=w957:refnum<queue>, error out=w937:errorcluster)  [unwired: 1 in, 1 out]
        n373 = call "QueueMotorStart.vi"("MotorNum"=w935, "Step"=w934, "Direction"=w933, "错误输入（无错误）"=w937, "MotorNum_Int"=6 ("元素"), "Step_Int"=20000 ("元素"), "Direction_Int"=1 ("元素")) -> ("MotorNum_OUT"=w915:refnum<queue>, "Step_OUT"=w916:refnum<queue>, "Direction_OUT"=w917:refnum<queue>, "错误输出"=w936:errorcluster)  [unwired: 9 in]
        n374 = Enqueue Element(queue=w957, element=T8."MotorStart" ("元素"), error in (no error)=w936) -> (queue out=w914:refnum<queue>, error out=w951:errorcluster)  [unwired: 1 in, 1 out]
        n375 = call "Check.vi"("错误输入（无错误）"=w951, "长度"=2, "索引"=4, "Array引用"=w907, "Bool引用"=w876) -> ("错误输出"=w946:errorcluster)  [unwired: 6 in]
        n376 = flat-sequence {
          tunnel: w946 -> [w1232]
          tunnel: [w1232] -> w906
          frame #0 {
            w1233 = 0
            n377 = property on="CurrentPosY" class="DigNum (严格)"("Value"=w1233) -> ()  [unwired: 2 in, 2 out]
            n378 = property on="CurrentPosX" class="DigNum (严格)"("Value"=w1233) -> ()  [unwired: 2 in, 2 out]
          }
        }
        n379 = control-ref of="FirstPosZ"() -> (w908:refnum<vi>)
        n380 = control-ref of="FirstPosX"() -> (w909:refnum<vi>)
        n381 = for {
          N: 16 -> [_]
          shift-right: [w990] -> _
          shift-left: w920 -> [w990]
          shift-right: [w989] -> _
          shift-left: w919 -> [w989]
          tunnel: w918 -> [w983]
          tunnel: w917 -> [w979]
          tunnel: w916 -> [w980]
          tunnel: w915 -> [w981]
          tunnel: w914 -> [w976]
          tunnel: w913 -> [w977]
          tunnel: w876 -> [w974]
          tunnel: w907 -> [w975]
          tunnel: w886 -> [w987]
          tunnel: w884 -> [w986]
          tunnel: w875 -> [w985]
          tunnel: w910 -> [w988]
          tunnel: w909 -> [w984]
          tunnel: w908 -> [w978]
          tunnel: w906 -> [w982]
          tunnel: w892 -> [_]
          tunnel: w874 -> [w972]
          tunnel: w871 -> [w971]
          tunnel: w870 -> [w970]
          i -> [w991]
          n382 = property on="Plat3StopBtn" class="Bool (严格)"() -> ("Value"=w973:bool)  [unwired: 2 in, 2 out]
          n383 = case shown="假" w973 {
            tunnel: w991 -> [w1204 _]
            tunnel: w990 -> [w1202 _]
            tunnel: w989 -> [w1201 _]
            tunnel: w988 -> [w1145 _]
            tunnel: w987 -> [w1141 _]
            tunnel: w986 -> [w1140 _]
            tunnel: w985 -> [w1037 _]
            tunnel: w984 -> [w1035 _]
            tunnel: w983 -> [w1015 _]
            tunnel: w982 -> [w1036 _]
            tunnel: w981 -> [w1079 _]
            tunnel: w980 -> [w1078 _]
            tunnel: w979 -> [w1077 _]
            tunnel: w978 -> [w992 _]
            tunnel: w977 -> [w1013 _]
            tunnel: w976 -> [w1025 _]
            tunnel: w975 -> [w1057 _]
            tunnel: w974 -> [w1039 _]
            tunnel: w972 -> [w1012 _]
            tunnel: w971 -> [w1029 _]
            tunnel: w970 -> [w1028 _]
            frame False {
              n384 = call "SpeedControl.vi"("XPos"=w1035, "CurrentX"=w1015, "YPos"=w992, "CurrentY"=w1013, "SelectPol"=w1012, "错误输入（无错误）"=w1036) -> ("1轴速度"=w1034:i32, "2轴速度"=w1027:i32, "错误输出"=w1032:errorcluster)  [unwired: 11 in]
              n385 = Quotient & Remainder(x=w1204, y=4) -> (x-y*floor(x/y)=w1146:i32, floor(x/y)=w1144:i32)
              n386 = case shown="1, 默认" w1145 {
                tunnel: w1146 -> [w1221 w1223]
                tunnel: w1144 -> [w1220 w1222]
                tunnel: [w1221 w1222] -> w1142
                tunnel: [w1220 w1223] -> w1143
                frame 1, Default {
                }
                frame 2 {
                }
              }
              n387 = call "SetSpeedQueue.vi"("MotorNum队列"=w1029, "MotorSpeed队列"=w1028, "MotorNum元素"=5, "MotorSpeed元素"=w1034, "错误输入（无错误）"=w1032) -> ("MotorNum队列输出"=w1031:refnum<queue>, "MotorSpeed队列输出"=w1030:refnum<queue>, "错误输出"=w1020:errorcluster)  [unwired: 8 in]
              n388 = Enqueue Element(queue=w1025, element=T4."SetMotorSpeed" ("元素"), error in (no error)=w1020) -> (queue out=w1022:refnum<queue>, error out=w1019:errorcluster)  [unwired: 1 in, 1 out]
              n389 = Index Array(array=w1201, index=w1143) -> (element=w1014:refnum<vi>)
              n390 = Index Array(array=w1202, index=w1142) -> (element=w1016:refnum<vi>)
              n391 = call "SetSpeedQueue.vi"("MotorNum队列"=w1031, "MotorSpeed队列"=w1030, "MotorNum元素"=6, "MotorSpeed元素"=w1027, "错误输入（无错误）"=w1019) -> ("MotorNum队列输出"=w996:refnum<queue>, "MotorSpeed队列输出"=w995:refnum<queue>, "错误输出"=w1024:errorcluster)  [unwired: 8 in]
              n392 = Enqueue Element(queue=w1022, element=T4."SetMotorSpeed" ("元素"), error in (no error)=w1024) -> (queue out=w1021:refnum<queue>, error out=w1023:errorcluster)  [unwired: 1 in, 1 out]
              n393 = call "ThridPlatX.vi"("错误输入（无错误）"=w1023, "CurrentX引用"=w1015, "X引用"=w1035) -> ("错误输出"=w1083:errorcluster, "Direction"=w1080:i32, "Step"=w1081:i32, "MotorNum"=w1082:i32)  [unwired: 5 in]
              n394 = call "QueueMotorStart.vi"("MotorNum"=w1079, "Step"=w1078, "Direction"=w1077, "错误输入（无错误）"=w1083, "MotorNum_Int"=w1082, "Step_Int"=w1081, "Direction_Int"=w1080) -> ("MotorNum_OUT"=w1070:refnum<queue>, "Step_OUT"=w1069:refnum<queue>, "Direction_OUT"=w1068:refnum<queue>, "错误输出"=w1076:errorcluster)  [unwired: 9 in]
              n395 = Enqueue Element(queue=w1021, element=T4."MotorStart" ("元素"), error in (no error)=w1076) -> (queue out=w1064:refnum<queue>, error out=w1075:errorcluster)  [unwired: 1 in, 1 out]
              n396 = call "ThridPlatY.vi"("错误输入（无错误）"=w1075, "CurrentY引用"=w1013, "Y引用"=w992) -> ("错误输出"=w1074:errorcluster, "Direction"=w1065:i32, "Step"=w1066:i32, "MotorNum"=w1067:i32)  [unwired: 5 in]
              n397 = call "QueueMotorStart.vi"("MotorNum"=w1070, "Step"=w1069, "Direction"=w1068, "错误输入（无错误）"=w1074, "MotorNum_Int"=w1067, "Step_Int"=w1066, "Direction_Int"=w1065) -> ("MotorNum_OUT"=w1060:refnum<queue>, "Step_OUT"=w1059:refnum<queue>, "Direction_OUT"=w1058:refnum<queue>, "错误输出"=w1073:errorcluster)  [unwired: 9 in]
              n398 = Enqueue Element(queue=w1064, element=T4."MotorStart" ("元素"), error in (no error)=w1073) -> (queue out=w1063:refnum<queue>, error out=w1072:errorcluster)  [unwired: 1 in, 1 out]
              n399 = call "Check.vi"("错误输入（无错误）"=w1072, "长度"=2, "索引"=4, "Array引用"=w1057, "Bool引用"=w1039) -> ("错误输出"=w1071:errorcluster)  [unwired: 6 in]
              n400 = call "QueueSolenAct.vi"("SolenNum_IN"=w1141, "SolenStatue_IN"=w1140, "SolenNum_Value"=34, "SolenStatue_Value"=1, "错误输入（无错误）"=w1071) -> ("SolenNum_OUT"=w1134:refnum<queue>, "SolenStatue_OUT"=w1133:refnum<queue>, "错误输出"=w1136:errorcluster)  [unwired: 8 in]
              n401 = Enqueue Element(queue=w1063, element=T8."SolenAction" ("元素"), error in (no error)=w1136) -> (queue out=w1048:refnum<queue>, error out=w1050:errorcluster)  [unwired: 1 in, 1 out]
              n402 = call "DelayPlat3.vi"("error In"=w1050, "DelayTime"=u32 1000, "Bool"=w1039) -> ("error Out"=w1049:errorcluster)  [unwired: 8 in]
              n403 = call "QueueSolenAct.vi"("SolenNum_IN"=w1134, "SolenStatue_IN"=w1133, "SolenNum_Value"=35, "SolenStatue_Value"=1, "错误输入（无错误）"=w1049) -> ("SolenNum_OUT"=w1129:refnum<queue>, "SolenStatue_OUT"=w1128:refnum<queue>, "错误输出"=w1135:errorcluster)  [unwired: 8 in]
              n404 = Enqueue Element(queue=w1048, element=T8."SolenAction" ("元素"), error in (no error)=w1135) -> (queue out=w1044:refnum<queue>, error out=w1046:errorcluster)  [unwired: 1 in, 1 out]
              n405 = call "DelayPlat3.vi"("error In"=w1046, "DelayTime"=u32 1000, "Bool"=w1039) -> ("error Out"=w1045:errorcluster)  [unwired: 8 in]
              n406 = call "QueueSolenAct.vi"("SolenNum_IN"=w1129, "SolenStatue_IN"=w1128, "SolenNum_Value"=34, "SolenStatue_Value"=0, "错误输入（无错误）"=w1045) -> ("SolenNum_OUT"=w1123:refnum<queue>, "SolenStatue_OUT"=w1122:refnum<queue>, "错误输出"=w1125:errorcluster)  [unwired: 8 in]
              n407 = Enqueue Element(queue=w1044, element=T8."SolenAction" ("元素"), error in (no error)=w1125) -> (queue out=w1117:refnum<queue>, error out=w1121:errorcluster)  [unwired: 1 in, 1 out]
              n408 = call "QueueSolenAct.vi"("SolenNum_IN"=w1123, "SolenStatue_IN"=w1122, "SolenNum_Value"=33, "SolenStatue_Value"=1, "错误输入（无错误）"=w1121) -> ("SolenNum_OUT"=w1114:refnum<queue>, "SolenStatue_OUT"=w1113:refnum<queue>, "错误输出"=w1118:errorcluster)  [unwired: 8 in]
              n409 = Enqueue Element(queue=w1117, element=T8."SolenAction" ("元素"), error in (no error)=w1118) -> (queue out=w1108:refnum<queue>, error out=w1115:errorcluster)  [unwired: 1 in, 1 out]
              n410 = flat-sequence {
                tunnel: [w1218] -> w1112
                tunnel: w1115 -> [w1219]
                tunnel: w1039 -> [w1217]
                tunnel: w1037 -> [w1216]
                frame #0 {
                  n411 = call "Check.vi"("错误输入（无错误）"=w1219, "长度"=1, "索引"=6, "Array引用"=w1216, "Bool引用"=w1217) -> ("错误输出"=w1218:errorcluster)  [unwired: 6 in]
                }
              }
              n412 = call "QueueSolenAct.vi"("SolenNum_IN"=w1114, "SolenStatue_IN"=w1113, "SolenNum_Value"=34, "SolenStatue_Value"=1, "错误输入（无错误）"=w1112) -> ("SolenNum_OUT"=w1106:refnum<queue>, "SolenStatue_OUT"=w1105:refnum<queue>, "错误输出"=w1109:errorcluster)  [unwired: 8 in]
              n413 = Enqueue Element(queue=w1108, element=T8."SolenAction" ("元素"), error in (no error)=w1109) -> (queue out=w1040:refnum<queue>, error out=w1042:errorcluster)  [unwired: 1 in, 1 out]
              n414 = call "DelayPlat3.vi"("error In"=w1042, "DelayTime"=u32 1000, "Bool"=w1039) -> ("error Out"=w1041:errorcluster)  [unwired: 8 in]
              n415 = call "QueueSolenAct.vi"("SolenNum_IN"=w1106, "SolenStatue_IN"=w1105, "SolenNum_Value"=35, "SolenStatue_Value"=0, "错误输入（无错误）"=w1041) -> ("SolenNum_OUT"=w1100:refnum<queue>, "SolenStatue_OUT"=w1099:refnum<queue>, "错误输出"=w1102:errorcluster)  [unwired: 8 in]
              n416 = Enqueue Element(queue=w1040, element=T8."SolenAction" ("元素"), error in (no error)=w1102) -> (queue out=w1095:refnum<queue>, error out=w1096:errorcluster)  [unwired: 1 in, 1 out]
              n417 = call "QueueSolenAct.vi"("SolenNum_IN"=w1100, "SolenStatue_IN"=w1099, "SolenNum_Value"=34, "SolenStatue_Value"=0, "错误输入（无错误）"=w1096) -> ("SolenNum_OUT"=w1092:refnum<queue>, "SolenStatue_OUT"=w1091:refnum<queue>, "错误输出"=w1094:errorcluster)  [unwired: 8 in]
              n418 = Enqueue Element(queue=w1095, element=T8."SolenAction" ("元素"), error in (no error)=w1094) -> (queue out=w1054:refnum<queue>, error out=w1053:errorcluster)  [unwired: 1 in, 1 out]
              n419 = flat-sequence {
                tunnel: w1053 -> [w1205]
                tunnel: [w1207] -> w1052
                tunnel: w1054 -> [w1207]
                tunnel: [w1205] -> w1051
                frame #0 {
                  n420 = Wait (ms)(milliseconds to wait=u32 1000 ("等待时间（毫秒）")) -> ()  [unwired: 1 out]
                }
              }
              n421 = call "QueueSolenAct.vi"("SolenNum_IN"=w1092, "SolenStatue_IN"=w1091, "SolenNum_Value"=32, "SolenStatue_Value"=1, "错误输入（无错误）"=w1051) -> ("SolenNum_OUT"=w1085:refnum<queue>, "SolenStatue_OUT"=w1084:refnum<queue>, "错误输出"=w1088:errorcluster)  [unwired: 8 in]
              n422 = Enqueue Element(queue=w1052, element=T8."SolenAction" ("元素"), error in (no error)=w1088) -> (queue out=w1001:refnum<queue>, error out=w1086:errorcluster)  [unwired: 1 in, 1 out]
              n423 = flat-sequence {
                tunnel: w1086 -> [w1213]
                tunnel: [w1212] -> w1011
                tunnel: w1039 -> [w1211]
                tunnel: w1037 -> [w1210]
                frame #0 {
                  n424 = call "Check.vi"("错误输入（无错误）"=w1213, "长度"=1, "索引"=7, "Array引用"=w1210, "Bool引用"=w1211) -> ("错误输出"=w1212:errorcluster)  [unwired: 6 in]
                }
              }
              n425 = call "SpeedControl.vi"("XPos"=w1016, "CurrentX"=w1015, "YPos"=w1014, "CurrentY"=w1013, "SelectPol"=w1012, "错误输入（无错误）"=w1011) -> ("1轴速度"=w1010:i32, "2轴速度"=w1004:i32, "错误输出"=w1009:errorcluster)  [unwired: 11 in]
              n426 = call "SetSpeedQueue.vi"("MotorNum队列"=w996, "MotorSpeed队列"=w995, "MotorNum元素"=5, "MotorSpeed元素"=w1010, "错误输入（无错误）"=w1009) -> ("MotorNum队列输出"=w994:refnum<queue>, "MotorSpeed队列输出"=w993:refnum<queue>, "错误输出"=w1008:errorcluster)  [unwired: 8 in]
              n427 = Enqueue Element(queue=w1001, element=T4."SetMotorSpeed" ("元素"), error in (no error)=w1008) -> (queue out=w1000:refnum<queue>, error out=w1007:errorcluster)  [unwired: 1 in, 1 out]
              n428 = call "SetSpeedQueue.vi"("MotorNum队列"=w994, "MotorSpeed队列"=w993, "MotorNum元素"=6, "MotorSpeed元素"=w1004, "错误输入（无错误）"=w1007) -> ("错误输出"=w1006:errorcluster)  [unwired: 8 in, 2 out]
              n429 = Enqueue Element(queue=w1000, element=T4."SetMotorSpeed" ("元素"), error in (no error)=w1006) -> (queue out=w999:refnum<queue>, error out=w1005:errorcluster)  [unwired: 1 in, 1 out]
              n430 = call "ThridPlatX.vi"("错误输入（无错误）"=w1005, "CurrentX引用"=w1015, "X引用"=w1016) -> ("错误输出"=w1200:errorcluster, "Direction"=w1197:i32, "Step"=w1198:i32, "MotorNum"=w1199:i32)  [unwired: 5 in]
              n431 = call "QueueMotorStart.vi"("MotorNum"=w1060, "Step"=w1059, "Direction"=w1058, "错误输入（无错误）"=w1200, "MotorNum_Int"=w1199, "Step_Int"=w1198, "Direction_Int"=w1197) -> ("MotorNum_OUT"=w1193:refnum<queue>, "Step_OUT"=w1192:refnum<queue>, "Direction_OUT"=w1191:refnum<queue>, "错误输出"=w1195:errorcluster)  [unwired: 9 in]
              n432 = Enqueue Element(queue=w999, element=T8."MotorStart" ("元素"), error in (no error)=w1195) -> (queue out=w1185:refnum<queue>, error out=w1194:errorcluster)  [unwired: 1 in, 1 out]
              n433 = call "ThridPlatY.vi"("错误输入（无错误）"=w1194, "CurrentY引用"=w1013, "Y引用"=w1014) -> ("错误输出"=w1190:errorcluster, "Direction"=w1187:i32, "Step"=w1188:i32, "MotorNum"=w1189:i32)  [unwired: 5 in]
              n434 = call "QueueMotorStart.vi"("MotorNum"=w1193, "Step"=w1192, "Direction"=w1191, "错误输入（无错误）"=w1190, "MotorNum_Int"=w1189, "Step_Int"=w1188, "Direction_Int"=w1187) -> ("MotorNum_OUT"=w1170:refnum<queue>, "Step_OUT"=w1169:refnum<queue>, "Direction_OUT"=w1168:refnum<queue>, "错误输出"=w1186:errorcluster)  [unwired: 9 in]
              n435 = Enqueue Element(queue=w1185, element=T8."MotorStart" ("元素"), error in (no error)=w1186) -> (queue out=w1176:refnum<queue>, error out=w1181:errorcluster)  [unwired: 1 in, 1 out]
              n436 = call "Check.vi"("错误输入（无错误）"=w1181, "长度"=2, "索引"=4, "Array引用"=w1057, "Bool引用"=w1039) -> ("错误输出"=w1180:errorcluster)  [unwired: 6 in]
              n437 = call "QueueSolenAct.vi"("SolenNum_IN"=w1085, "SolenStatue_IN"=w1084, "SolenNum_Value"=37, "SolenStatue_Value"=1, "错误输入（无错误）"=w1180) -> ("SolenNum_OUT"=w1156:refnum<queue>, "SolenStatue_OUT"=w1155:refnum<queue>, "错误输出"=w1177:errorcluster)  [unwired: 8 in]
              n438 = Enqueue Element(queue=w1176, element=T8."SolenAction" ("元素"), error in (no error)=w1177) -> (queue out=w1164:refnum<queue>, error out=w1172:errorcluster)  [unwired: 1 in, 1 out]
              n439 = call "Check.vi"("错误输入（无错误）"=w1172, "长度"=1, "索引"=5, "Array引用"=w1037, "Bool引用"=w1039) -> ("错误输出"=w1171:errorcluster)  [unwired: 6 in]
              n440 = call "QueueMotorStart.vi"("MotorNum"=w1170, "Step"=w1169, "Direction"=w1168, "错误输入（无错误）"=w1171, "MotorNum_Int"=6, "Step_Int"=500, "Direction_Int"=1) -> ("错误输出"=w1148:errorcluster)  [unwired: 9 in, 3 out]
              n441 = flat-sequence {
                tunnel: w1148 -> [w1227]
                tunnel: [w1225] -> w1147
                tunnel: w1013 -> [w1228]
                frame #0 {
                  n442 = property class="DigNum (严格)"(reference=w1228, error in=w1227) -> (reference out=w1224:refnum<vi>, error out=w1226:errorcluster, "Value"=w1231:i32)
                  n443 = Add(x=w1231, y=500) -> (x+y=w1229:i32)
                  n444 = property class="DigNum (严格)"(reference=w1224, error in=w1226, "Value"=w1229) -> (error out=w1225:errorcluster)  [unwired: 1 out]
                }
              }
              n445 = Enqueue Element(queue=w1164, element=T8."MotorStart" ("元素"), error in (no error)=w1147) -> (queue out=w1151:refnum<queue>, error out=w1162:errorcluster)  [unwired: 1 in, 1 out]
              n446 = call "Check.vi"("错误输入（无错误）"=w1162, "长度"=1, "索引"=5, "Array引用"=w1057, "Bool引用"=w1039) -> ("错误输出"=w1157:errorcluster)  [unwired: 6 in]
              n447 = call "QueueSolenAct.vi"("SolenNum_IN"=w1156, "SolenStatue_IN"=w1155, "SolenNum_Value"=36, "SolenStatue_Value"=1, "错误输入（无错误）"=w1157) -> ("错误输出"=w1152:errorcluster)  [unwired: 8 in, 2 out]
              n448 = Enqueue Element(queue=w1151, element=T8."SolenAction" ("元素"), error in (no error)=w1152) -> (error out=w1149:errorcluster)  [unwired: 1 in, 2 out]
              n449 = call "Check.vi"("错误输入（无错误）"=w1149, "长度"=1, "索引"=4, "Array引用"=w1037, "Bool引用"=w1039) -> ()  [unwired: 6 in, 1 out]
            }
            frame True {
            }
          }
        }
      }
      event "Plat3GetMegBtn": Value Change {
        n450 = event-data() -> ()  [unwired: 1 in, 5 out]
        n451 = Flush Queue(queue=w1328, error in (no error)=w1327) -> (queue out=w1305:refnum<queue>)  [unwired: 2 out]
        n452 = Flush Queue(queue=w1326, error in (no error)=w1325) -> (queue out=w1304:refnum<queue>)  [unwired: 2 out]
        n453 = Flush Queue(queue=w1324, error in (no error)=w1323) -> (queue out=w1303:refnum<queue>)  [unwired: 2 out]
        n454 = Flush Queue(queue=w1331, error in (no error)=w1330) -> (queue out=w1291:refnum<queue>)  [unwired: 2 out]
        n455 = Flush Queue(queue=w1333, error in (no error)=w1332) -> (queue out=w1263:refnum<queue>)  [unwired: 2 out]
        n456 = Flush Queue(queue=w1258, error in (no error)=w1257) -> (queue out=w1256:refnum<queue>)  [unwired: 2 out]
        n457 = Flush Queue(queue=w1237) -> (queue out=w1235:refnum<queue>)  [unwired: 1 in, 2 out]
        n458 = Flush Queue(queue=w1236) -> (queue out=w1234:refnum<queue>)  [unwired: 1 in, 2 out]
        n459 = Flush Queue(queue=w1288) -> (queue out=w1268:refnum<queue>)  [unwired: 1 in, 2 out]
        n460 = Flush Queue(queue=w1287) -> (queue out=w1267:refnum<queue>)  [unwired: 1 in, 2 out]
        n461 = Flush Queue(queue=w1312, error in (no error)=w1311) -> (queue out=w1290:refnum<queue>, error out=w1269:errorcluster)  [unwired: 1 out]
        n462 = control-ref of="ComboPolicy"() -> (w1276:refnum<vi>)
        n463 = control-ref of="CurrentPosX"() -> (w1282:refnum<vi>)
        n464 = control-ref of="CurrentPosY"() -> (w1277:refnum<vi>)
        n465 = control-ref of="Plat3StopBtn"() -> (w1240:refnum<vi>)
        n466 = control-ref of="SelectPolicy"() -> (w1238:refnum<vi>)
        n467 = property class="CmbBox"(reference=w1276) -> ("Value"=w1275:string)  [unwired: 1 in, 2 out]
        n468 = call "QueueSolenAct.vi"("SolenNum_IN"=w1268, "SolenStatue_IN"=w1267, "SolenNum_Value"=32, "SolenStatue_Value"=1, "错误输入（无错误）"=w1269) -> ("SolenNum_OUT"=w1251:refnum<queue>, "SolenStatue_OUT"=w1249:refnum<queue>, "错误输出"=w1264:errorcluster)  [unwired: 8 in]
        n469 = control-ref of="solenstatue output"() -> (w1286:refnum<vi>)
        n470 = Decimal String To Number(string=w1275) -> (number=w1274:i32)  [unwired: 2 in, 1 out]
        n471 = Enqueue Element(queue=w1263, element=T8."SolenAction" ("元素"), error in (no error)=w1264) -> (queue out=w1255:refnum<queue>, error out=w1261:errorcluster)  [unwired: 1 in, 1 out]
        n472 = control-ref of="platformStatue2 output"() -> (w1239:refnum<vi>)
        n473 = control-ref of="motor statue array output"() -> (w1271:refnum<vi>)
        n474 = call "Check.vi"("错误输入（无错误）"=w1261, "长度"=1, "索引"=7, "Array引用"=w1239, "Bool引用"=w1240) -> ("错误输出"=w1253:errorcluster)  [unwired: 6 in]
        n475 = call "QueueSolenAct.vi"("SolenNum_IN"=w1251, "SolenStatue_IN"=w1249, "SolenNum_Value"=36, "SolenStatue_Value"=1, "错误输入（无错误）"=w1253) -> ("SolenNum_OUT"=w1250:refnum<queue>, "SolenStatue_OUT"=w1248:refnum<queue>, "错误输出"=w1252:errorcluster)  [unwired: 8 in]
        n476 = Enqueue Element(queue=w1255, element=T4."SolenAction" ("元素"), error in (no error)=w1252) -> (queue out=w1254:refnum<queue>, error out=w1244:errorcluster)  [unwired: 1 in, 1 out]
        n477 = call "Check.vi"("错误输入（无错误）"=w1244, "长度"=1, "索引"=4, "Array引用"=w1239, "Bool引用"=w1240) -> ("错误输出"=w1243:errorcluster)  [unwired: 6 in]
        n478 = call "QueueSolenAdv.vi"("Statue_IN"=w1290, "PlatNum_IN"=w1291, "Statue_Value"=0 ("元素"), "PlatNum_Value"=2 ("元素"), "错误输入（无错误）"=w1243) -> ("错误输出"=w1289:errorcluster)  [unwired: 8 in, 2 out]
        n479 = Enqueue Element(queue=w1254, element=T8."SolenAdv" ("元素"), error in (no error)=w1289) -> (queue out=w1316:refnum<queue>, error out=w1319:errorcluster)  [unwired: 1 in, 1 out]
        n480 = call "Check.vi"("错误输入（无错误）"=w1319, "长度"=16, "索引"=32, "Array引用"=w1286, "Bool引用"=w1240) -> ("错误输出"=w1309:errorcluster)  [unwired: 6 in]
        n481 = call "QueueMotorStart.vi"("MotorNum"=w1305, "Step"=w1304, "Direction"=w1303, "错误输入（无错误）"=w1309, "MotorNum_Int"=5 ("元素"), "Step_Int"=20000 ("元素"), "Direction_Int"=0 ("元素")) -> ("MotorNum_OUT"=w1299:refnum<queue>, "Step_OUT"=w1298:refnum<queue>, "Direction_OUT"=w1297:refnum<queue>, "错误输出"=w1302:errorcluster)  [unwired: 9 in]
        n482 = Enqueue Element(queue=w1316, element=T8."MotorStart" ("元素"), error in (no error)=w1302) -> (queue out=w1321:refnum<queue>, error out=w1301:errorcluster)  [unwired: 1 in, 1 out]
        n483 = call "QueueMotorStart.vi"("MotorNum"=w1299, "Step"=w1298, "Direction"=w1297, "错误输入（无错误）"=w1301, "MotorNum_Int"=6 ("元素"), "Step_Int"=20000 ("元素"), "Direction_Int"=1 ("元素")) -> ("MotorNum_OUT"=w1279:refnum<queue>, "Step_OUT"=w1280:refnum<queue>, "Direction_OUT"=w1281:refnum<queue>, "错误输出"=w1300:errorcluster)  [unwired: 9 in]
        n484 = Enqueue Element(queue=w1321, element=T8."MotorStart" ("元素"), error in (no error)=w1300) -> (queue out=w1278:refnum<queue>, error out=w1315:errorcluster)  [unwired: 1 in, 1 out]
        n485 = call "Check.vi"("错误输入（无错误）"=w1315, "长度"=2, "索引"=4, "Array引用"=w1271, "Bool引用"=w1240) -> ("错误输出"=w1310:errorcluster)  [unwired: 6 in]
        n486 = flat-sequence {
          tunnel: w1310 -> [w1599]
          tunnel: [w1599] -> w1270
          frame #0 {
            w1600 = 0
            n487 = property on="CurrentPosY" class="DigNum (严格)"("Value"=w1600) -> ()  [unwired: 2 in, 2 out]
            n488 = property on="CurrentPosX" class="DigNum (严格)"("Value"=w1600) -> ()  [unwired: 2 in, 2 out]
          }
        }
        n489 = control-ref of="FirstPosZ"() -> (w1272:refnum<vi>)
        n490 = control-ref of="FirstPosX"() -> (w1273:refnum<vi>)
        n491 = for {
          N: 16 -> [_]
          shift-right: [w1354] -> _
          shift-left: w1284 -> [w1354]
          shift-right: [w1353] -> _
          shift-left: w1283 -> [w1353]
          tunnel: w1282 -> [w1347]
          tunnel: w1281 -> [w1343]
          tunnel: w1280 -> [w1344]
          tunnel: w1279 -> [w1345]
          tunnel: w1278 -> [w1340]
          tunnel: w1277 -> [w1341]
          tunnel: w1240 -> [w1338]
          tunnel: w1271 -> [w1339]
          tunnel: w1250 -> [w1351]
          tunnel: w1248 -> [w1350]
          tunnel: w1239 -> [w1349]
          tunnel: w1274 -> [w1352]
          tunnel: w1273 -> [w1348]
          tunnel: w1272 -> [w1342]
          tunnel: w1270 -> [w1346]
          tunnel: w1256 -> [_]
          tunnel: w1238 -> [w1336]
          tunnel: w1235 -> [w1335]
          tunnel: w1234 -> [w1334]
          i -> [w1355]
          n492 = property on="Plat3StopBtn" class="Bool (严格)"() -> ("Value"=w1337:bool)  [unwired: 2 in, 2 out]
          n493 = case shown="假" w1337 {
            tunnel: w1355 -> [w1569 _]
            tunnel: w1354 -> [w1567 _]
            tunnel: w1353 -> [w1566 _]
            tunnel: w1352 -> [w1510 _]
            tunnel: w1351 -> [w1506 _]
            tunnel: w1350 -> [w1505 _]
            tunnel: w1349 -> [w1403 _]
            tunnel: w1348 -> [w1401 _]
            tunnel: w1347 -> [w1381 _]
            tunnel: w1346 -> [w1402 _]
            tunnel: w1345 -> [w1444 _]
            tunnel: w1344 -> [w1443 _]
            tunnel: w1343 -> [w1442 _]
            tunnel: w1342 -> [w1358 _]
            tunnel: w1341 -> [w1379 _]
            tunnel: w1340 -> [w1391 _]
            tunnel: w1339 -> [w1422 _]
            tunnel: w1338 -> [w1405 _]
            tunnel: w1336 -> [w1378 _]
            tunnel: w1335 -> [w1395 _]
            tunnel: w1334 -> [w1394 _]
            frame False {
              n494 = call "SpeedControl.vi"("XPos"=w1401, "CurrentX"=w1381, "YPos"=w1358, "CurrentY"=w1379, "SelectPol"=w1378, "错误输入（无错误）"=w1402) -> ("1轴速度"=w1400:i32, "2轴速度"=w1393:i32, "错误输出"=w1398:errorcluster)  [unwired: 11 in]
              n495 = Quotient & Remainder(x=w1569, y=4) -> (x-y*floor(x/y)=w1511:i32, floor(x/y)=w1509:i32)
              n496 = case shown="1, 默认" w1510 {
                tunnel: w1511 -> [w1588 w1590]
                tunnel: w1509 -> [w1587 w1589]
                tunnel: [w1588 w1589] -> w1507
                tunnel: [w1587 w1590] -> w1508
                frame 1, Default {
                }
                frame 2 {
                }
              }
              n497 = call "SetSpeedQueue.vi"("MotorNum队列"=w1395, "MotorSpeed队列"=w1394, "MotorNum元素"=5, "MotorSpeed元素"=w1400, "错误输入（无错误）"=w1398) -> ("MotorNum队列输出"=w1397:refnum<queue>, "MotorSpeed队列输出"=w1396:refnum<queue>, "错误输出"=w1386:errorcluster)  [unwired: 8 in]
              n498 = Enqueue Element(queue=w1391, element=T4."SetMotorSpeed" ("元素"), error in (no error)=w1386) -> (queue out=w1388:refnum<queue>, error out=w1385:errorcluster)  [unwired: 1 in, 1 out]
              n499 = Index Array(array=w1566, index=w1508) -> (element=w1380:refnum<vi>)
              n500 = Index Array(array=w1567, index=w1507) -> (element=w1382:refnum<vi>)
              n501 = call "SetSpeedQueue.vi"("MotorNum队列"=w1397, "MotorSpeed队列"=w1396, "MotorNum元素"=6, "MotorSpeed元素"=w1393, "错误输入（无错误）"=w1385) -> ("MotorNum队列输出"=w1362:refnum<queue>, "MotorSpeed队列输出"=w1361:refnum<queue>, "错误输出"=w1390:errorcluster)  [unwired: 8 in]
              n502 = Enqueue Element(queue=w1388, element=T4."SetMotorSpeed" ("元素"), error in (no error)=w1390) -> (queue out=w1387:refnum<queue>, error out=w1389:errorcluster)  [unwired: 1 in, 1 out]
              n503 = call "ThridPlatX.vi"("错误输入（无错误）"=w1389, "CurrentX引用"=w1381, "X引用"=w1401) -> ("错误输出"=w1448:errorcluster, "Direction"=w1445:i32, "Step"=w1446:i32, "MotorNum"=w1447:i32)  [unwired: 5 in]
              n504 = call "QueueMotorStart.vi"("MotorNum"=w1444, "Step"=w1443, "Direction"=w1442, "错误输入（无错误）"=w1448, "MotorNum_Int"=w1447, "Step_Int"=w1446, "Direction_Int"=w1445) -> ("MotorNum_OUT"=w1435:refnum<queue>, "Step_OUT"=w1434:refnum<queue>, "Direction_OUT"=w1433:refnum<queue>, "错误输出"=w1441:errorcluster)  [unwired: 9 in]
              n505 = Enqueue Element(queue=w1387, element=T4."MotorStart" ("元素"), error in (no error)=w1441) -> (queue out=w1429:refnum<queue>, error out=w1440:errorcluster)  [unwired: 1 in, 1 out]
              n506 = call "ThridPlatY.vi"("错误输入（无错误）"=w1440, "CurrentY引用"=w1379, "Y引用"=w1358) -> ("错误输出"=w1439:errorcluster, "Direction"=w1430:i32, "Step"=w1431:i32, "MotorNum"=w1432:i32)  [unwired: 5 in]
              n507 = call "QueueMotorStart.vi"("MotorNum"=w1435, "Step"=w1434, "Direction"=w1433, "错误输入（无错误）"=w1439, "MotorNum_Int"=w1432, "Step_Int"=w1431, "Direction_Int"=w1430) -> ("MotorNum_OUT"=w1425:refnum<queue>, "Step_OUT"=w1424:refnum<queue>, "Direction_OUT"=w1423:refnum<queue>, "错误输出"=w1438:errorcluster)  [unwired: 9 in]
              n508 = Enqueue Element(queue=w1429, element=T4."MotorStart" ("元素"), error in (no error)=w1438) -> (queue out=w1428:refnum<queue>, error out=w1437:errorcluster)  [unwired: 1 in, 1 out]
              n509 = call "Check.vi"("错误输入（无错误）"=w1437, "长度"=2, "索引"=4, "Array引用"=w1422, "Bool引用"=w1405) -> ("错误输出"=w1436:errorcluster)  [unwired: 6 in]
              n510 = call "QueueSolenAct.vi"("SolenNum_IN"=w1506, "SolenStatue_IN"=w1505, "SolenNum_Value"=34, "SolenStatue_Value"=1, "错误输入（无错误）"=w1436) -> ("SolenNum_OUT"=w1499:refnum<queue>, "SolenStatue_OUT"=w1498:refnum<queue>, "错误输出"=w1501:errorcluster)  [unwired: 8 in]
              n511 = Enqueue Element(queue=w1428, element=T8."SolenAction" ("元素"), error in (no error)=w1501) -> (queue out=w1414:refnum<queue>, error out=w1415:errorcluster)  [unwired: 1 in, 1 out]
              n512 = call "DelayPlat3.vi"("error In"=w1415, "DelayTime"=u32 1000, "Bool"=w1405) -> ("error Out"=w1357:errorcluster)  [unwired: 8 in]
              n513 = flat-sequence {
                tunnel: w1357 -> [w1570]
                tunnel: [w1570] -> w1356
                frame #0 {
                  n514 = local read "Stog"() -> (w1571:dbl)
                  n515 = local write "电桥称重"(w1571) -> ()
                }
              }
              n516 = call "QueueSolenAct.vi"("SolenNum_IN"=w1499, "SolenStatue_IN"=w1498, "SolenNum_Value"=35, "SolenStatue_Value"=1, "错误输入（无错误）"=w1356) -> ("SolenNum_OUT"=w1494:refnum<queue>, "SolenStatue_OUT"=w1493:refnum<queue>, "错误输出"=w1500:errorcluster)  [unwired: 8 in]
              n517 = Enqueue Element(queue=w1414, element=T8."SolenAction" ("元素"), error in (no error)=w1500) -> (queue out=w1410:refnum<queue>, error out=w1412:errorcluster)  [unwired: 1 in, 1 out]
              n518 = call "DelayPlat3.vi"("error In"=w1412, "DelayTime"=u32 1000, "Bool"=w1405) -> ("error Out"=w1411:errorcluster)  [unwired: 8 in]
              n519 = call "QueueSolenAct.vi"("SolenNum_IN"=w1494, "SolenStatue_IN"=w1493, "SolenNum_Value"=34, "SolenStatue_Value"=0, "错误输入（无错误）"=w1411) -> ("SolenNum_OUT"=w1488:refnum<queue>, "SolenStatue_OUT"=w1487:refnum<queue>, "错误输出"=w1490:errorcluster)  [unwired: 8 in]
              n520 = Enqueue Element(queue=w1410, element=T8."SolenAction" ("元素"), error in (no error)=w1490) -> (queue out=w1482:refnum<queue>, error out=w1486:errorcluster)  [unwired: 1 in, 1 out]
              n521 = call "QueueSolenAct.vi"("SolenNum_IN"=w1488, "SolenStatue_IN"=w1487, "SolenNum_Value"=33, "SolenStatue_Value"=1, "错误输入（无错误）"=w1486) -> ("SolenNum_OUT"=w1479:refnum<queue>, "SolenStatue_OUT"=w1478:refnum<queue>, "错误输出"=w1483:errorcluster)  [unwired: 8 in]
              n522 = Enqueue Element(queue=w1482, element=T8."SolenAction" ("元素"), error in (no error)=w1483) -> (queue out=w1473:refnum<queue>, error out=w1480:errorcluster)  [unwired: 1 in, 1 out]
              n523 = flat-sequence {
                tunnel: [w1585] -> w1477
                tunnel: w1480 -> [w1586]
                tunnel: w1405 -> [w1584]
                tunnel: w1403 -> [w1583]
                frame #0 {
                  n524 = call "Check.vi"("错误输入（无错误）"=w1586, "长度"=1, "索引"=6, "Array引用"=w1583, "Bool引用"=w1584) -> ("错误输出"=w1585:errorcluster)  [unwired: 6 in]
                }
              }
              n525 = call "QueueSolenAct.vi"("SolenNum_IN"=w1479, "SolenStatue_IN"=w1478, "SolenNum_Value"=34, "SolenStatue_Value"=1, "错误输入（无错误）"=w1477) -> ("SolenNum_OUT"=w1471:refnum<queue>, "SolenStatue_OUT"=w1470:refnum<queue>, "错误输出"=w1474:errorcluster)  [unwired: 8 in]
              n526 = Enqueue Element(queue=w1473, element=T8."SolenAction" ("元素"), error in (no error)=w1474) -> (queue out=w1406:refnum<queue>, error out=w1408:errorcluster)  [unwired: 1 in, 1 out]
              n527 = call "DelayPlat3.vi"("error In"=w1408, "DelayTime"=u32 1000, "Bool"=w1405) -> ("error Out"=w1407:errorcluster)  [unwired: 8 in]
              n528 = call "QueueSolenAct.vi"("SolenNum_IN"=w1471, "SolenStatue_IN"=w1470, "SolenNum_Value"=35, "SolenStatue_Value"=0, "错误输入（无错误）"=w1407) -> ("SolenNum_OUT"=w1465:refnum<queue>, "SolenStatue_OUT"=w1464:refnum<queue>, "错误输出"=w1467:errorcluster)  [unwired: 8 in]
              n529 = Enqueue Element(queue=w1406, element=T8."SolenAction" ("元素"), error in (no error)=w1467) -> (queue out=w1460:refnum<queue>, error out=w1461:errorcluster)  [unwired: 1 in, 1 out]
              n530 = call "QueueSolenAct.vi"("SolenNum_IN"=w1465, "SolenStatue_IN"=w1464, "SolenNum_Value"=34, "SolenStatue_Value"=0, "错误输入（无错误）"=w1461) -> ("SolenNum_OUT"=w1457:refnum<queue>, "SolenStatue_OUT"=w1456:refnum<queue>, "错误输出"=w1459:errorcluster)  [unwired: 8 in]
              n531 = Enqueue Element(queue=w1460, element=T8."SolenAction" ("元素"), error in (no error)=w1459) -> (queue out=w1419:refnum<queue>, error out=w1418:errorcluster)  [unwired: 1 in, 1 out]
              n532 = flat-sequence {
                tunnel: w1418 -> [w1572]
                tunnel: [w1574] -> w1417
                tunnel: w1419 -> [w1574]
                tunnel: [w1572] -> w1416
                frame #0 {
                  n533 = Wait (ms)(milliseconds to wait=u32 1000 ("等待时间（毫秒）")) -> ()  [unwired: 1 out]
                }
              }
              n534 = call "QueueSolenAct.vi"("SolenNum_IN"=w1457, "SolenStatue_IN"=w1456, "SolenNum_Value"=32, "SolenStatue_Value"=1, "错误输入（无错误）"=w1416) -> ("SolenNum_OUT"=w1450:refnum<queue>, "SolenStatue_OUT"=w1449:refnum<queue>, "错误输出"=w1453:errorcluster)  [unwired: 8 in]
              n535 = Enqueue Element(queue=w1417, element=T8."SolenAction" ("元素"), error in (no error)=w1453) -> (queue out=w1367:refnum<queue>, error out=w1451:errorcluster)  [unwired: 1 in, 1 out]
              n536 = flat-sequence {
                tunnel: w1451 -> [w1580]
                tunnel: [w1579] -> w1377
                tunnel: w1405 -> [w1578]
                tunnel: w1403 -> [w1577]
                frame #0 {
                  n537 = call "Check.vi"("错误输入（无错误）"=w1580, "长度"=1, "索引"=7, "Array引用"=w1577, "Bool引用"=w1578) -> ("错误输出"=w1579:errorcluster)  [unwired: 6 in]
                }
              }
              n538 = call "SpeedControl.vi"("XPos"=w1382, "CurrentX"=w1381, "YPos"=w1380, "CurrentY"=w1379, "SelectPol"=w1378, "错误输入（无错误）"=w1377) -> ("1轴速度"=w1376:i32, "2轴速度"=w1370:i32, "错误输出"=w1375:errorcluster)  [unwired: 11 in]
              n539 = call "SetSpeedQueue.vi"("MotorNum队列"=w1362, "MotorSpeed队列"=w1361, "MotorNum元素"=5, "MotorSpeed元素"=w1376, "错误输入（无错误）"=w1375) -> ("MotorNum队列输出"=w1360:refnum<queue>, "MotorSpeed队列输出"=w1359:refnum<queue>, "错误输出"=w1374:errorcluster)  [unwired: 8 in]
              n540 = Enqueue Element(queue=w1367, element=T4."SetMotorSpeed" ("元素"), error in (no error)=w1374) -> (queue out=w1366:refnum<queue>, error out=w1373:errorcluster)  [unwired: 1 in, 1 out]
              n541 = call "SetSpeedQueue.vi"("MotorNum队列"=w1360, "MotorSpeed队列"=w1359, "MotorNum元素"=6, "MotorSpeed元素"=w1370, "错误输入（无错误）"=w1373) -> ("错误输出"=w1372:errorcluster)  [unwired: 8 in, 2 out]
              n542 = Enqueue Element(queue=w1366, element=T4."SetMotorSpeed" ("元素"), error in (no error)=w1372) -> (queue out=w1365:refnum<queue>, error out=w1371:errorcluster)  [unwired: 1 in, 1 out]
              n543 = call "ThridPlatX.vi"("错误输入（无错误）"=w1371, "CurrentX引用"=w1381, "X引用"=w1382) -> ("错误输出"=w1565:errorcluster, "Direction"=w1562:i32, "Step"=w1563:i32, "MotorNum"=w1564:i32)  [unwired: 5 in]
              n544 = call "QueueMotorStart.vi"("MotorNum"=w1425, "Step"=w1424, "Direction"=w1423, "错误输入（无错误）"=w1565, "MotorNum_Int"=w1564, "Step_Int"=w1563, "Direction_Int"=w1562) -> ("MotorNum_OUT"=w1558:refnum<queue>, "Step_OUT"=w1557:refnum<queue>, "Direction_OUT"=w1556:refnum<queue>, "错误输出"=w1560:errorcluster)  [unwired: 9 in]
              n545 = Enqueue Element(queue=w1365, element=T8."MotorStart" ("元素"), error in (no error)=w1560) -> (queue out=w1550:refnum<queue>, error out=w1559:errorcluster)  [unwired: 1 in, 1 out]
              n546 = call "ThridPlatY.vi"("错误输入（无错误）"=w1559, "CurrentY引用"=w1379, "Y引用"=w1380) -> ("错误输出"=w1555:errorcluster, "Direction"=w1552:i32, "Step"=w1553:i32, "MotorNum"=w1554:i32)  [unwired: 5 in]
              n547 = call "QueueMotorStart.vi"("MotorNum"=w1558, "Step"=w1557, "Direction"=w1556, "错误输入（无错误）"=w1555, "MotorNum_Int"=w1554, "Step_Int"=w1553, "Direction_Int"=w1552) -> ("MotorNum_OUT"=w1535:refnum<queue>, "Step_OUT"=w1534:refnum<queue>, "Direction_OUT"=w1533:refnum<queue>, "错误输出"=w1551:errorcluster)  [unwired: 9 in]
              n548 = Enqueue Element(queue=w1550, element=T8."MotorStart" ("元素"), error in (no error)=w1551) -> (queue out=w1541:refnum<queue>, error out=w1546:errorcluster)  [unwired: 1 in, 1 out]
              n549 = call "Check.vi"("错误输入（无错误）"=w1546, "长度"=2, "索引"=4, "Array引用"=w1422, "Bool引用"=w1405) -> ("错误输出"=w1545:errorcluster)  [unwired: 6 in]
              n550 = call "QueueSolenAct.vi"("SolenNum_IN"=w1450, "SolenStatue_IN"=w1449, "SolenNum_Value"=37, "SolenStatue_Value"=1, "错误输入（无错误）"=w1545) -> ("SolenNum_OUT"=w1521:refnum<queue>, "SolenStatue_OUT"=w1520:refnum<queue>, "错误输出"=w1542:errorcluster)  [unwired: 8 in]
              n551 = Enqueue Element(queue=w1541, element=T8."SolenAction" ("元素"), error in (no error)=w1542) -> (queue out=w1529:refnum<queue>, error out=w1537:errorcluster)  [unwired: 1 in, 1 out]
              n552 = call "Check.vi"("错误输入（无错误）"=w1537, "长度"=1, "索引"=5, "Array引用"=w1403, "Bool引用"=w1405) -> ("错误输出"=w1536:errorcluster)  [unwired: 6 in]
              n553 = call "QueueMotorStart.vi"("MotorNum"=w1535, "Step"=w1534, "Direction"=w1533, "错误输入（无错误）"=w1536, "MotorNum_Int"=6, "Step_Int"=500, "Direction_Int"=1) -> ("错误输出"=w1513:errorcluster)  [unwired: 9 in, 3 out]
              n554 = flat-sequence {
                tunnel: w1513 -> [w1594]
                tunnel: [w1592] -> w1512
                tunnel: w1379 -> [w1595]
                frame #0 {
                  n555 = property class="DigNum (严格)"(reference=w1595, error in=w1594) -> (reference out=w1591:refnum<vi>, error out=w1593:errorcluster, "Value"=w1598:i32)
                  n556 = Add(x=w1598, y=500) -> (x+y=w1596:i32)
                  n557 = property class="DigNum (严格)"(reference=w1591, error in=w1593, "Value"=w1596) -> (error out=w1592:errorcluster)  [unwired: 1 out]
                }
              }
              n558 = Enqueue Element(queue=w1529, element=T8."MotorStart" ("元素"), error in (no error)=w1512) -> (queue out=w1516:refnum<queue>, error out=w1527:errorcluster)  [unwired: 1 in, 1 out]
              n559 = call "Check.vi"("错误输入（无错误）"=w1527, "长度"=1, "索引"=5, "Array引用"=w1422, "Bool引用"=w1405) -> ("错误输出"=w1522:errorcluster)  [unwired: 6 in]
              n560 = call "QueueSolenAct.vi"("SolenNum_IN"=w1521, "SolenStatue_IN"=w1520, "SolenNum_Value"=36, "SolenStatue_Value"=1, "错误输入（无错误）"=w1522) -> ("错误输出"=w1517:errorcluster)  [unwired: 8 in, 2 out]
              n561 = Enqueue Element(queue=w1516, element=T8."SolenAction" ("元素"), error in (no error)=w1517) -> (error out=w1514:errorcluster)  [unwired: 1 in, 2 out]
              n562 = call "Check.vi"("错误输入（无错误）"=w1514, "长度"=1, "索引"=4, "Array引用"=w1403, "Bool引用"=w1405) -> ()  [unwired: 6 in, 1 out]
            }
            frame True {
            }
          }
        }
      }
      event "Plat3MulitBtn": Value Change {
        n563 = event-data() -> ()  [unwired: 1 in, 5 out]
        n564 = Flush Queue(queue=w1711) -> (error out=w1697:errorcluster)  [unwired: 1 in, 2 out]
        n565 = Flush Queue(queue=w1604) -> (queue out=w1603:refnum<queue>)  [unwired: 1 in, 2 out]
        n566 = Flush Queue(queue=w1606) -> (queue out=w1605:refnum<queue>)  [unwired: 1 in, 2 out]
        n567 = property on="while-control" class="Bool (严格)"("Value"=FALSE ("while-control")) -> (error out=w1601:errorcluster)  [unwired: 2 in, 1 out]
        n568 = control-ref of="ComboPolicy"() -> (w1614:refnum<vi>)
        n569 = Flush Queue(queue=w1710, error in (no error)=w1697) -> (error out=w1696:errorcluster)  [unwired: 2 out]
        n570 = control-ref of="Plat3StopBtn"() -> (w1621:refnum<vi>)
        n571 = control-ref of="CurrentPosX"() -> (w1618:refnum<vi>)
        n572 = control-ref of="CurrentPosY"() -> (w1617:refnum<vi>)
        n573 = control-ref of="SelectPolicy"() -> (w1607:refnum<vi>)
        n574 = property class="CmbBox"(reference=w1614) -> ("Value"=w1613:string)  [unwired: 1 in, 2 out]
        n575 = Flush Queue(queue=w1709, error in (no error)=w1696) -> (queue out=w1608:refnum<queue>, error out=w1695:errorcluster)  [unwired: 1 out]
        n576 = control-ref of="solenstatue output"() -> (w1656:refnum<vi>)
        n577 = Decimal String To Number(string=w1613) -> (number=w1612:i32)  [unwired: 2 in, 1 out]
        n578 = Flush Queue(queue=w1708, error in (no error)=w1695) -> (queue out=w1609:refnum<queue>, error out=w1687:errorcluster)  [unwired: 1 out]
        n579 = control-ref of="platformStatue2 output"() -> (w1620:refnum<vi>)
        n580 = control-ref of="motor statue array output"() -> (w1619:refnum<vi>)
        n581 = Flush Queue(queue=w1707, error in (no error)=w1687) -> (queue out=w1636:refnum<queue>, error out=w1694:errorcluster)  [unwired: 1 out]
        n582 = Flush Queue(queue=w1706, error in (no error)=w1694) -> (queue out=w1634:refnum<queue>, error out=w1693:errorcluster)  [unwired: 1 out]
        n583 = Flush Queue(queue=w1705, error in (no error)=w1693) -> (queue out=w1635:refnum<queue>, error out=w1692:errorcluster)  [unwired: 1 out]
        n584 = Flush Queue(queue=w1704, error in (no error)=w1692) -> (queue out=w1663:refnum<queue>, error out=w1691:errorcluster)  [unwired: 1 out]
        n585 = Flush Queue(queue=w1703, error in (no error)=w1691) -> (queue out=w1684:refnum<queue>, error out=w1689:errorcluster)  [unwired: 1 out]
        n586 = Flush Queue(queue=w1702, error in (no error)=w1689) -> (queue out=w1682:refnum<queue>, error out=w1690:errorcluster)  [unwired: 1 out]
        n587 = Flush Queue(queue=w1701, error in (no error)=w1690) -> (queue out=w1681:refnum<queue>, error out=w1688:errorcluster)  [unwired: 1 out]
        n588 = Flush Queue(queue=w1700, error in (no error)=w1688) -> (queue out=w1662:refnum<queue>, error out=w1680:errorcluster)  [unwired: 1 out]
        n589 = call "QueueSolenAct.vi"("SolenNum_IN"=w1682, "SolenStatue_IN"=w1681, "SolenNum_Value"=32, "SolenStatue_Value"=1, "错误输入（无错误）"=w1680) -> ("SolenNum_OUT"=w1674:refnum<queue>, "SolenStatue_OUT"=w1673:refnum<queue>, "错误输出"=w1679:errorcluster)  [unwired: 8 in]
        n590 = Enqueue Element(queue=w1684, element=T4."SolenAction" ("元素"), error in (no error)=w1679) -> (queue out=w1672:refnum<queue>, error out=w1678:errorcluster)  [unwired: 1 in, 1 out]
        n591 = call "Check.vi"("错误输入（无错误）"=w1678, "长度"=1, "索引"=7, "Array引用"=w1620, "Bool引用"=w1621) -> ("错误输出"=w1675:errorcluster)  [unwired: 6 in]
        n592 = call "QueueSolenAct.vi"("SolenNum_IN"=w1674, "SolenStatue_IN"=w1673, "SolenNum_Value"=36, "SolenStatue_Value"=1, "错误输入（无错误）"=w1675) -> ("SolenNum_OUT"=w1627:refnum<queue>, "SolenStatue_OUT"=w1626:refnum<queue>, "错误输出"=w1671:errorcluster)  [unwired: 8 in]
        n593 = Enqueue Element(queue=w1672, element=T4."SolenAction" ("元素"), error in (no error)=w1671) -> (queue out=w1660:refnum<queue>, error out=w1669:errorcluster)  [unwired: 1 in, 1 out]
        n594 = call "Check.vi"("错误输入（无错误）"=w1669, "长度"=1, "索引"=4, "Array引用"=w1620, "Bool引用"=w1621) -> ("错误输出"=w1664:errorcluster)  [unwired: 6 in]
        n595 = call "QueueSolenAdv.vi"("Statue_IN"=w1662, "PlatNum_IN"=w1663, "Statue_Value"=0 ("元素"), "PlatNum_Value"=2 ("元素"), "错误输入（无错误）"=w1664) -> ("错误输出"=w1661:errorcluster)  [unwired: 8 in, 2 out]
        n596 = Enqueue Element(queue=w1660, element=T4."SolenAdv" ("元素"), error in (no error)=w1661) -> (queue out=w1651:refnum<queue>, error out=w1655:errorcluster)  [unwired: 1 in, 1 out]
        n597 = call "Check.vi"("错误输入（无错误）"=w1655, "长度"=16, "索引"=32, "Array引用"=w1656, "Bool引用"=w1621) -> ("错误输出"=w1637:errorcluster)  [unwired: 6 in]
        n598 = call "QueueMotorStart.vi"("MotorNum"=w1636, "Step"=w1634, "Direction"=w1635, "错误输入（无错误）"=w1637, "MotorNum_Int"=5 ("元素"), "Step_Int"=20000 ("元素"), "Direction_Int"=0 ("元素")) -> ("MotorNum_OUT"=w1646:refnum<queue>, "Step_OUT"=w1645:refnum<queue>, "Direction_OUT"=w1644:refnum<queue>, "错误输出"=w1643:errorcluster)  [unwired: 9 in]
        n599 = Enqueue Element(queue=w1651, element=T4."MotorStart" ("元素"), error in (no error)=w1643) -> (queue out=w1633:refnum<queue>, error out=w1642:errorcluster)  [unwired: 1 in, 1 out]
        n600 = call "QueueMotorStart.vi"("MotorNum"=w1646, "Step"=w1645, "Direction"=w1644, "错误输入（无错误）"=w1642, "MotorNum_Int"=6 ("元素"), "Step_Int"=20000 ("元素"), "Direction_Int"=1 ("元素")) -> ("MotorNum_OUT"=w1624:refnum<queue>, "Step_OUT"=w1623:refnum<queue>, "Direction_OUT"=w1622:refnum<queue>, "错误输出"=w1641:errorcluster)  [unwired: 9 in]
        n601 = Enqueue Element(queue=w1633, element=T4."MotorStart" ("元素"), error in (no error)=w1641) -> (queue out=w1625:refnum<queue>, error out=w1640:errorcluster)  [unwired: 1 in, 1 out]
        n602 = call "Check.vi"("错误输入（无错误）"=w1640, "长度"=2, "索引"=4, "Array引用"=w1619, "Bool引用"=w1621) -> ("错误输出"=w1631:errorcluster)  [unwired: 6 in]
        n603 = flat-sequence {
          tunnel: [w2068] -> w1629
          tunnel: w1631 -> [w2068]
          frame #0 {
            w2067 = 0
            n604 = property on="CurrentPosY" class="DigNum (严格)"("Value"=w2067) -> ()  [unwired: 2 in, 2 out]
            n605 = property on="CurrentPosX" class="DigNum (严格)"("Value"=w2067) -> ()  [unwired: 2 in, 2 out]
          }
        }
        n606 = property on="Plat3StopBtn" class="Bool (严格)"(error in=w1629) -> (error out=w1628:errorcluster, "Value"=w1630:bool)  [unwired: 1 in, 1 out]
        n607 = control-ref of="FirstPosX"() -> (w1616:refnum<vi>)
        n608 = control-ref of="FirstPosZ"() -> (w1615:refnum<vi>)
        n609 = case shown="假" w1630 {
          tunnel: w1628 -> [_ _]
          tunnel: w1627 -> [w1732 _]
          tunnel: w1626 -> [w1731 _]
          tunnel: w1625 -> [w1730 _]
          tunnel: w1624 -> [w1735 _]
          tunnel: w1623 -> [w1734 _]
          tunnel: w1622 -> [w1733 _]
          tunnel: w1621 -> [w1727 _]
          tunnel: w1620 -> [w1726 _]
          tunnel: w1619 -> [w1716 _]
          tunnel: w1618 -> [w1721 _]
          tunnel: w1617 -> [w1720 _]
          tunnel: w1616 -> [w1724 _]
          tunnel: w1615 -> [w1723 _]
          tunnel: w1607 -> [w1712 _]
          tunnel: w1612 -> [w1713 _]
          tunnel: w1611 -> [w1715 _]
          tunnel: w1610 -> [w1714 _]
          tunnel: w1609 -> [w1717 _]
          tunnel: w1608 -> [w1718 _]
          tunnel: w1607 -> [w1719 _]
          tunnel: w1605 -> [w1729 _]
          tunnel: w1603 -> [w1728 _]
          tunnel: w1601 -> [_ _]
          frame False {
            n610 = while {
              tunnel: w1735 -> [w1969]
              tunnel: w1734 -> [w1968]
              tunnel: w1733 -> [w1967]
              tunnel: w1730 -> [w1964]
              tunnel: w1732 -> [w1966]
              tunnel: w1731 -> [w1965]
              shift-right: [w1961] -> _
              shift-left: enum16{"机械手取料", "机械手放料"}."机械手取料" -> [w1970]
              tunnel: w1726 -> [w1963]
              tunnel: w1727 -> [w1962]
              tunnel: w1729 -> [w1960]
              tunnel: w1728 -> [w1959]
              stop <- w1956 stop-if-true
              n611 = case shown="\"机械手取料\", 默认" w1970 {
                tunnel: w1969 -> [_ _]
                tunnel: w1968 -> [_ _]
                tunnel: w1967 -> [_ _]
                tunnel: w1966 -> [w2011 w2019]
                tunnel: w1965 -> [w2010 w2018]
                tunnel: w1964 -> [w2006 w2017]
                tunnel: w1963 -> [w1973 w2015]
                tunnel: w1962 -> [w1974 w2016]
                tunnel: [w1972 w2020] -> w1961
                tunnel: w1960 -> [_ w2014]
                tunnel: w1959 -> [_ w2021]
                frame "机械手取料", Default {
                  (unwired) T4."SolenAction" ("元素")
                  n612 = call "QueueSolenAct.vi"("SolenNum_IN"=w2011, "SolenStatue_IN"=w2010, "SolenNum_Value"=32, "SolenStatue_Value"=1) -> ("SolenNum_OUT"=w2000:refnum<queue>, "SolenStatue_OUT"=w1999:refnum<queue>, "错误输出"=w2007:errorcluster)  [unwired: 9 in]
                  n613 = Enqueue Element(queue=w2006, element=T4."SolenAction" ("元素"), error in (no error)=w2007) -> (queue out=w1995:refnum<queue>, error out=w2004:errorcluster)  [unwired: 1 in, 1 out]
                  n614 = call "Check.vi"("错误输入（无错误）"=w2004, "长度"=1, "索引"=7, "Array引用"=w1973, "Bool引用"=w1974) -> ("错误输出"=w2001:errorcluster)  [unwired: 6 in]
                  n615 = call "QueueSolenAct.vi"("SolenNum_IN"=w2000, "SolenStatue_IN"=w1999, "SolenNum_Value"=34, "SolenStatue_Value"=1, "错误输入（无错误）"=w2001) -> ("SolenNum_OUT"=w1991:refnum<queue>, "SolenStatue_OUT"=w1990:refnum<queue>, "错误输出"=w1996:errorcluster)  [unwired: 8 in]
                  n616 = Enqueue Element(queue=w1995, element=T4."SolenAction" ("元素"), error in (no error)=w1996) -> (queue out=w1985:refnum<queue>, error out=w1993:errorcluster)  [unwired: 1 in, 1 out]
                  n617 = call "DelayPlat3.vi"("error In"=w1993, "DelayTime"=u32 1000, "Bool"=w1974) -> ("error Out"=w1989:errorcluster)  [unwired: 8 in]
                  n618 = call "QueueSolenAct.vi"("SolenNum_IN"=w1991, "SolenStatue_IN"=w1990, "SolenNum_Value"=35, "SolenStatue_Value"=1, "错误输入（无错误）"=w1989) -> ("SolenNum_OUT"=w1983:refnum<queue>, "SolenStatue_OUT"=w1982:refnum<queue>, "错误输出"=w1986:errorcluster)  [unwired: 8 in]
                  n619 = Enqueue Element(queue=w1985, element=T4."SolenAction" ("元素"), error in (no error)=w1986) -> (queue out=w1977:refnum<queue>, error out=w1981:errorcluster)  [unwired: 1 in, 1 out]
                  n620 = call "QueueSolenAct.vi"("SolenNum_IN"=w1983, "SolenStatue_IN"=w1982, "SolenNum_Value"=34, "SolenStatue_Value"=0, "错误输入（无错误）"=w1981) -> ("错误输出"=w1978:errorcluster)  [unwired: 8 in, 2 out]
                  n621 = Enqueue Element(queue=w1977, element=T4."SolenAction" ("元素"), error in (no error)=w1978) -> (error out=w1975:errorcluster)  [unwired: 1 in, 2 out]
                  n622 = call "DelayPlat3.vi"("error In"=w1975, "Bool"=w1974) -> ("error Out"=w1971:errorcluster)  [unwired: 9 in]
                  n623 = flat-sequence {
                    tunnel: [enum16{"机械手取料", "机械手放料"}."机械手放料"] -> w1972
                    tunnel: w1971 -> [_]
                    frame #0 {
                    }
                  }
                }
                frame "机械手放料" {
                  n624 = Dequeue Element(queue=w2021) -> (element=w2013:enum16{"仓库2维运动完成", "NOPE"})  [unwired: 2 in, 3 out]
                  n625 = case shown="\"仓库2维运动完成\"" w2013 {
                    tunnel: [w2038 enum16{"机械手取料", "机械手放料"}."机械手放料"] -> w2020
                    tunnel: w2019 -> [w2031 _]
                    tunnel: w2018 -> [w2030 _]
                    tunnel: w2017 -> [w2027 _]
                    tunnel: w2016 -> [w2024 _]
                    tunnel: w2015 -> [w2023 _]
                    tunnel: w2014 -> [w2042 _]
                    frame "仓库2维运动完成" {
                      n626 = call "QueueSolenAct.vi"("SolenNum_IN"=w2031, "SolenStatue_IN"=w2030, "SolenNum_Value"=33, "SolenStatue_Value"=1) -> ("SolenNum_OUT"=w2029:refnum<queue>, "SolenStatue_OUT"=w2028:refnum<queue>, "错误输出"=w2035:errorcluster)  [unwired: 9 in]
                      n627 = Enqueue Element(queue=w2027, element=T4."SolenAction" ("元素"), error in (no error)=w2035) -> (queue out=w2026:refnum<queue>, error out=w2034:errorcluster)  [unwired: 1 in, 1 out]
                      n628 = call "Check.vi"("错误输入（无错误）"=w2034, "长度"=1, "索引"=6, "Array引用"=w2023, "Bool引用"=w2024) -> ("错误输出"=w2025:errorcluster)  [unwired: 6 in]
                      n629 = call "QueueSolenAct.vi"("SolenNum_IN"=w2029, "SolenStatue_IN"=w2028, "SolenNum_Value"=34, "SolenStatue_Value"=1, "错误输入（无错误）"=w2025) -> ("SolenNum_OUT"=w2057:refnum<queue>, "SolenStatue_OUT"=w2056:refnum<queue>, "错误输出"=w2062:errorcluster)  [unwired: 8 in]
                      n630 = Enqueue Element(queue=w2026, element=T4."SolenAction" ("元素"), error in (no error)=w2062) -> (queue out=w2052:refnum<queue>, error out=w2060:errorcluster)  [unwired: 1 in, 1 out]
                      n631 = call "DelayPlat3.vi"("error In"=w2060, "DelayTime"=u32 1000, "Bool"=w2024) -> ("error Out"=w2058:errorcluster)  [unwired: 8 in]
                      n632 = call "QueueSolenAct.vi"("SolenNum_IN"=w2057, "SolenStatue_IN"=w2056, "SolenNum_Value"=35, "SolenStatue_Value"=0, "错误输入（无错误）"=w2058) -> ("SolenNum_OUT"=w2049:refnum<queue>, "SolenStatue_OUT"=w2048:refnum<queue>, "错误输出"=w2053:errorcluster)  [unwired: 8 in]
                      n633 = Enqueue Element(queue=w2052, element=T4."SolenAction" ("元素"), error in (no error)=w2053) -> (queue out=w2044:refnum<queue>, error out=w2050:errorcluster)  [unwired: 1 in, 1 out]
                      n634 = call "QueueSolenAct.vi"("SolenNum_IN"=w2049, "SolenStatue_IN"=w2048, "SolenNum_Value"=34, "SolenStatue_Value"=0, "错误输入（无错误）"=w2050) -> ("错误输出"=w2045:errorcluster)  [unwired: 8 in, 2 out]
                      n635 = Enqueue Element(queue=w2044, element=T4."SolenAction" ("元素"), error in (no error)=w2045) -> (error out=w2041:errorcluster)  [unwired: 1 in, 2 out]
                      n636 = Enqueue Element(queue=w2042, element=enum16{"机械手动作完成"}."机械手动作完成" ("元素"), error in (no error)=w2041) -> (error out=w2039:errorcluster)  [unwired: 1 in, 2 out]
                      n637 = flat-sequence {
                        tunnel: w2039 -> [_]
                        tunnel: [enum16{"机械手取料", "机械手放料"}."机械手取料"] -> w2038
                        frame #0 {
                        }
                      }
                    }
                    frame "NOPE", Default {
                    }
                  }
                }
              }
              n638 = property on="while-control" class="Bool (严格)"() -> ("Value"=w1958:bool)  [unwired: 2 in, 2 out]
              n639 = property on="Plat3StopBtn" class="Bool (严格)"() -> ("Value"=w1957:bool)  [unwired: 2 in, 2 out]
              n640 = Or(x=w1958, y=w1957) -> (x .or. y?=w1956:bool)
            }
            n641 = while {
              tunnel: w1735 -> [w1760]
              tunnel: w1734 -> [w1759]
              tunnel: w1733 -> [w1758]
              tunnel: w1732 -> [w1743]
              tunnel: w1731 -> [w1742]
              tunnel: w1730 -> [w1763]
              tunnel: w1729 -> [w1749]
              tunnel: w1728 -> [w1750]
              tunnel: w1727 -> [w1755]
              tunnel: w1726 -> [w1744]
              shift-right: [w1753] -> _
              shift-left: enum16{"回取料点", "放置物料"}."回取料点" -> [w1751]
              tunnel: w1724 -> [w1762]
              tunnel: w1723 -> [w1757]
              shift-right: [w1752] -> _
              shift-left: 0 -> [w1741]
              tunnel: w1721 -> [w1761]
              tunnel: w1720 -> [w1756]
              tunnel: w1719 -> [w1766]
              tunnel: w1718 -> [w1765]
              tunnel: w1717 -> [w1764]
              tunnel: w1716 -> [w1754]
              tunnel: w1715 -> [w1748]
              tunnel: w1714 -> [w1747]
              tunnel: w1713 -> [w1746]
              tunnel: w1712 -> [w1745]
              stop <- w1737 stop-if-true
              n642 = case shown="\"放置物料\"" w1751 {
                tunnel: w1766 -> [w1818 _]
                tunnel: w1765 -> [w1814 w1830]
                tunnel: w1764 -> [w1813 w1829]
                tunnel: w1763 -> [w1812 w1828]
                tunnel: w1762 -> [w1801 _]
                tunnel: w1761 -> [w1800 w1833]
                tunnel: w1760 -> [w1796 w1827]
                tunnel: w1759 -> [w1795 w1826]
                tunnel: w1758 -> [w1794 w1825]
                tunnel: w1757 -> [w1790 _]
                tunnel: w1756 -> [w1789 w1832]
                tunnel: w1755 -> [w1776 w1824]
                tunnel: w1754 -> [w1775 w1822]
                tunnel: [w1772 w1839] -> w1753
                tunnel: w1741 -> [w1771 w1838]
                tunnel: [w1771 w1837] -> w1752
                tunnel: w1750 -> [w1768 _]
                tunnel: w1749 -> [_ w1841]
                tunnel: w1748 -> [_ w1835]
                tunnel: w1747 -> [_ w1836]
                tunnel: w1746 -> [_ w1834]
                tunnel: w1745 -> [_ w1831]
                tunnel: w1744 -> [_ w1823]
                tunnel: w1743 -> [_ w1821]
                tunnel: w1742 -> [_ w1820]
                frame "回取料点", Default {
                  n643 = call "SpeedControl.vi"("XPos"=w1801, "CurrentX"=w1800, "YPos"=w1790, "CurrentY"=w1789, "SelectPol"=w1818) -> ("1轴速度"=w1817:i32, "2轴速度"=w1807:i32, "错误输出"=w1816:errorcluster)  [unwired: 12 in]
                  n644 = call "SetSpeedQueue.vi"("MotorNum队列"=w1814, "MotorSpeed队列"=w1813, "MotorNum元素"=5, "MotorSpeed元素"=w1817, "错误输入（无错误）"=w1816) -> ("MotorNum队列输出"=w1809:refnum<queue>, "MotorSpeed队列输出"=w1808:refnum<queue>, "错误输出"=w1811:errorcluster)  [unwired: 8 in]
                  n645 = Enqueue Element(queue=w1812, element=T4."SetMotorSpeed" ("元素"), error in (no error)=w1811) -> (queue out=w1805:refnum<queue>)  [unwired: 1 in, 2 out]
                  n646 = call "SetSpeedQueue.vi"("MotorNum队列"=w1809, "MotorSpeed队列"=w1808, "MotorNum元素"=6, "MotorSpeed元素"=w1807) -> ("错误输出"=w1804:errorcluster)  [unwired: 9 in, 2 out]
                  n647 = Enqueue Element(queue=w1805, element=T4."SetMotorSpeed" ("元素"), error in (no error)=w1804) -> (queue out=w1792:refnum<queue>, error out=w1802:errorcluster)  [unwired: 1 in, 1 out]
                  n648 = call "ThridPlatX.vi"("错误输入（无错误）"=w1802, "CurrentX引用"=w1800, "X引用"=w1801) -> ("Direction"=w1797:i32, "Step"=w1798:i32, "MotorNum"=w1799:i32)  [unwired: 5 in, 1 out]
                  n649 = call "QueueMotorStart.vi"("MotorNum"=w1796, "Step"=w1795, "Direction"=w1794, "MotorNum_Int"=w1799, "Step_Int"=w1798, "Direction_Int"=w1797) -> ("MotorNum_OUT"=w1783:refnum<queue>, "Step_OUT"=w1782:refnum<queue>, "Direction_OUT"=w1781:refnum<queue>, "错误输出"=w1793:errorcluster)  [unwired: 10 in]
                  n650 = Enqueue Element(queue=w1792, element=T4."MotorStart" ("元素"), error in (no error)=w1793) -> (queue out=w1780:refnum<queue>, error out=w1788:errorcluster)  [unwired: 1 in, 1 out]
                  n651 = call "ThridPlatY.vi"("错误输入（无错误）"=w1788, "CurrentY引用"=w1789, "Y引用"=w1790) -> ("错误输出"=w1784:errorcluster, "Direction"=w1785:i32, "Step"=w1786:i32, "MotorNum"=w1787:i32)  [unwired: 5 in]
                  n652 = call "QueueMotorStart.vi"("MotorNum"=w1783, "Step"=w1782, "Direction"=w1781, "错误输入（无错误）"=w1784, "MotorNum_Int"=w1787, "Step_Int"=w1786, "Direction_Int"=w1785) -> ("错误输出"=w1779:errorcluster)  [unwired: 9 in, 3 out]
                  n653 = Enqueue Element(queue=w1780, element=T4."MotorStart" ("元素"), error in (no error)=w1779) -> (error out=w1777:errorcluster)  [unwired: 1 in, 2 out]
                  n654 = call "Check.vi"("错误输入（无错误）"=w1777, "长度"=2, "索引"=4, "Array引用"=w1775, "Bool引用"=w1776) -> ("错误输出"=w1770:errorcluster)  [unwired: 6 in]
                  n655 = Enqueue Element(queue=w1768, element=enum16{"仓库2维运动完成", "NOPE"}."仓库2维运动完成" ("元素"), error in (no error)=w1770) -> (error out=w1769:errorcluster)  [unwired: 1 in, 2 out]
                  n656 = flat-sequence {
                    tunnel: [enum16{"回取料点", "放置物料"}."放置物料"] -> w1772
                    tunnel: w1769 -> [_]
                    frame #0 {
                    }
                  }
                }
                frame "放置物料" {
                  n657 = Dequeue Element(queue=w1841) -> (element=w1840:enum16{"机械手动作完成", "NOPE"})  [unwired: 2 in, 3 out]
                  n658 = case shown="\"机械手动作完成\", 默认" w1840 {
                    tunnel: [w1885 enum16{"回取料点", "放置物料"}."放置物料"] -> w1839
                    tunnel: w1838 -> [w1884 w1954]
                    tunnel: [w1883 w1954] -> w1837
                    tunnel: w1836 -> [w1932 _]
                    tunnel: w1835 -> [w1934 _]
                    tunnel: w1834 -> [w1938 _]
                    tunnel: w1833 -> [w1911 _]
                    tunnel: w1832 -> [w1861 _]
                    tunnel: w1831 -> [w1930 _]
                    tunnel: w1830 -> [w1926 _]
                    tunnel: w1829 -> [w1925 _]
                    tunnel: w1828 -> [w1924 _]
                    tunnel: w1827 -> [w1906 _]
                    tunnel: w1826 -> [w1905 _]
                    tunnel: w1825 -> [w1904 _]
                    tunnel: w1824 -> [w1850 _]
                    tunnel: w1823 -> [w1849 _]
                    tunnel: w1822 -> [w1858 _]
                    tunnel: w1821 -> [w1881 _]
                    tunnel: w1820 -> [w1880 _]
                    frame "机械手动作完成", Default {
                      w1860 = 500 ("Step_Int")
                      n659 = Quotient & Remainder(x=w1884, y=4) -> (x-y*floor(x/y)=w1936:i32, floor(x/y)=w1935:i32)
                      n660 = case shown="2" w1938 {
                        tunnel: [w1951 w1953] -> w1933
                        tunnel: w1936 -> [w1950 w1953]
                        tunnel: [w1950 w1952] -> w1931
                        tunnel: w1935 -> [w1951 w1952]
                        frame 1, Default {
                        }
                        frame 2 {
                        }
                      }
                      n661 = Index Array(array=w1932, index=w1931) -> (element=w1912:refnum<vi>)
                      n662 = Index Array(array=w1934, index=w1933) -> (element=w1899:refnum<vi>)
                      n663 = call "SpeedControl.vi"("XPos"=w1912, "CurrentX"=w1911, "YPos"=w1899, "CurrentY"=w1861, "SelectPol"=w1930) -> ("1轴速度"=w1929:i32, "2轴速度"=w1918:i32, "错误输出"=w1928:errorcluster)  [unwired: 12 in]
                      n664 = call "SetSpeedQueue.vi"("MotorNum队列"=w1926, "MotorSpeed队列"=w1925, "MotorNum元素"=5, "MotorSpeed元素"=w1929, "错误输入（无错误）"=w1928) -> ("MotorNum队列输出"=w1921:refnum<queue>, "MotorSpeed队列输出"=w1920:refnum<queue>, "错误输出"=w1923:errorcluster)  [unwired: 8 in]
                      n665 = Enqueue Element(queue=w1924, element=T4."SetMotorSpeed" ("元素"), error in (no error)=w1923) -> (queue out=w1916:refnum<queue>, error out=w1919:errorcluster)  [unwired: 1 in, 1 out]
                      n666 = call "SetSpeedQueue.vi"("MotorNum队列"=w1921, "MotorSpeed队列"=w1920, "MotorNum元素"=6, "MotorSpeed元素"=w1918, "错误输入（无错误）"=w1919) -> ("错误输出"=w1915:errorcluster)  [unwired: 8 in, 2 out]
                      n667 = Enqueue Element(queue=w1916, element=T4."SetMotorSpeed" ("元素"), error in (no error)=w1915) -> (queue out=w1902:refnum<queue>, error out=w1913:errorcluster)  [unwired: 1 in, 1 out]
                      n668 = call "ThridPlatX.vi"("错误输入（无错误）"=w1913, "CurrentX引用"=w1911, "X引用"=w1912) -> ("错误输出"=w1910:errorcluster, "Direction"=w1907:i32, "Step"=w1908:i32, "MotorNum"=w1909:i32)  [unwired: 5 in]
                      n669 = call "QueueMotorStart.vi"("MotorNum"=w1906, "Step"=w1905, "Direction"=w1904, "错误输入（无错误）"=w1910, "MotorNum_Int"=w1909, "Step_Int"=w1908, "Direction_Int"=w1907) -> ("MotorNum_OUT"=w1894:refnum<queue>, "Step_OUT"=w1893:refnum<queue>, "Direction_OUT"=w1892:refnum<queue>, "错误输出"=w1903:errorcluster)  [unwired: 9 in]
                      n670 = Enqueue Element(queue=w1902, element=T4."MotorStart" ("元素"), error in (no error)=w1903) -> (queue out=w1890:refnum<queue>, error out=w1900:errorcluster)  [unwired: 1 in, 1 out]
                      n671 = call "ThridPlatY.vi"("错误输入（无错误）"=w1900, "CurrentY引用"=w1861, "Y引用"=w1899) -> ("错误输出"=w1895:errorcluster, "Direction"=w1896:i32, "Step"=w1897:i32, "MotorNum"=w1898:i32)  [unwired: 5 in]
                      n672 = call "QueueMotorStart.vi"("MotorNum"=w1894, "Step"=w1893, "Direction"=w1892, "错误输入（无错误）"=w1895, "MotorNum_Int"=w1898, "Step_Int"=w1897, "Direction_Int"=w1896) -> ("MotorNum_OUT"=w1871:refnum<queue>, "Step_OUT"=w1870:refnum<queue>, "Direction_OUT"=w1869:refnum<queue>, "错误输出"=w1891:errorcluster)  [unwired: 9 in]
                      n673 = Enqueue Element(queue=w1890, element=T4."MotorStart" ("元素"), error in (no error)=w1891) -> (queue out=w1877:refnum<queue>, error out=w1888:errorcluster)  [unwired: 1 in, 1 out]
                      n674 = call "Check.vi"("错误输入（无错误）"=w1888, "长度"=2, "索引"=4, "Array引用"=w1858, "Bool引用"=w1850) -> ("错误输出"=w1882:errorcluster)  [unwired: 6 in]
                      n675 = call "QueueSolenAct.vi"("SolenNum_IN"=w1881, "SolenStatue_IN"=w1880, "SolenNum_Value"=37, "SolenStatue_Value"=1, "错误输入（无错误）"=w1882) -> ("SolenNum_OUT"=w1855:refnum<queue>, "SolenStatue_OUT"=w1854:refnum<queue>, "错误输出"=w1876:errorcluster)  [unwired: 8 in]
                      n676 = Enqueue Element(queue=w1877, element=T4."SolenAction" ("元素"), error in (no error)=w1876) -> (queue out=w1864:refnum<queue>, error out=w1874:errorcluster)  [unwired: 1 in, 1 out]
                      n677 = call "Check.vi"("错误输入（无错误）"=w1874, "长度"=1, "索引"=5, "Array引用"=w1849, "Bool引用"=w1850) -> ("错误输出"=w1868:errorcluster)  [unwired: 6 in]
                      n678 = call "QueueMotorStart.vi"("MotorNum"=w1871, "Step"=w1870, "Direction"=w1869, "错误输入（无错误）"=w1868, "MotorNum_Int"=6, "Step_Int"=w1860, "Direction_Int"=1) -> ("错误输出"=w1865:errorcluster)  [unwired: 9 in, 3 out]
                      n679 = Enqueue Element(queue=w1864, element=T4."MotorStart" ("元素"), error in (no error)=w1865) -> (queue out=w1843:refnum<queue>, error out=w1862:errorcluster)  [unwired: 1 in, 1 out]
                      n680 = flat-sequence {
                        tunnel: w1862 -> [w1941]
                        tunnel: w1861 -> [w1942]
                        tunnel: w1860 -> [w1945]
                        tunnel: [w1939] -> w1859
                        frame #0 {
                          n681 = property class="DigNum (严格)"(reference=w1942, error in=w1941) -> (reference out=w1943:refnum<vi>, error out=w1940:errorcluster, "Value"=w1946:i32)
                          n682 = Add(x=w1946, y=w1945) -> (x+y=w1944:i32)
                          n683 = property class="DigNum (严格)"(reference=w1943, error in=w1940, "Value"=w1944) -> (error out=w1939:errorcluster)  [unwired: 1 out]
                        }
                      }
                      n684 = call "Check.vi"("错误输入（无错误）"=w1859, "长度"=2, "索引"=4, "Array引用"=w1858, "Bool引用"=w1850) -> ("错误输出"=w1853:errorcluster)  [unwired: 6 in]
                      n685 = call "QueueSolenAct.vi"("SolenNum_IN"=w1855, "SolenStatue_IN"=w1854, "SolenNum_Value"=36, "SolenStatue_Value"=1, "错误输入（无错误）"=w1853) -> ("错误输出"=w1845:errorcluster)  [unwired: 8 in, 2 out]
                      n686 = Enqueue Element(queue=w1843, element=T4."SolenAction" ("元素"), error in (no error)=w1845) -> (error out=w1844:errorcluster)  [unwired: 1 in, 2 out]
                      n687 = call "Check.vi"("错误输入（无错误）"=w1844, "长度"=1, "索引"=4, "Array引用"=w1849, "Bool引用"=w1850) -> ("错误输出"=w1846:errorcluster)  [unwired: 6 in]
                      n688 = flat-sequence {
                        tunnel: [enum16{"回取料点", "放置物料"}."回取料点"] -> w1885
                        tunnel: w1884 -> [w1948]
                        tunnel: [w1947] -> w1883
                        tunnel: w1846 -> [_]
                        frame #0 {
                          n689 = Increment(x=w1948) -> (x+1=w1947:i32)
                        }
                      }
                    }
                    frame "NOPE" {
                    }
                  }
                }
              }
              n690 = Equal?(x=w1741, y=16) -> (x = y?=w1738:bool)
              "while-control" <- w1738
              n691 = property on="Plat3StopBtn" class="Bool (严格)"() -> ("Value"=w1739:bool)  [unwired: 2 in, 2 out]
              n692 = Or(x=w1738, y=w1739) -> (x .or. y?=w1737:bool)
            }
          }
          frame True {
          }
        }
      }
      event "Plat3StopBtn": Value Change {
        n693 = event-data() -> ()  [unwired: 1 in, 5 out]
        n694 = flat-sequence {
          tunnel: [w2090] -> w2080
          tunnel: [w2089] -> w2079
          tunnel: [w2088] -> w2078
          tunnel: w2083 -> [w2098]
          tunnel: w2082 -> [w2099]
          tunnel: w2081 -> [w2093]
          tunnel: w2077 -> [w2087]
          tunnel: w2076 -> [w2086]
          tunnel: [w2085] -> w2074
          tunnel: [w2084] -> w2072
          tunnel: w2080 -> [w2106]
          tunnel: w2079 -> [w2108]
          tunnel: w2078 -> [w2109]
          tunnel: [w2103] -> w2075
          tunnel: w2074 -> [w2103]
          tunnel: [w2102] -> w2073
          tunnel: w2072 -> [w2102]
          tunnel: [w2101] -> w2071
          tunnel: [w2100] -> w2070
          tunnel: w2075 -> [w2118]
          tunnel: w2073 -> [w2117]
          tunnel: w2071 -> [w2114]
          tunnel: w2070 -> [w2112]
          tunnel: [w2110] -> w2069
          tunnel: w2069 -> [_]
          frame #0 {
            n695 = Flush Queue(queue=w2086) -> (queue out=w2084:refnum<queue>)  [unwired: 1 in, 2 out]
            n696 = Flush Queue(queue=w2093) -> (queue out=w2092:refnum<queue>)  [unwired: 1 in, 2 out]
            n697 = Flush Queue(queue=w2098, error in (no error)=w2099) -> (queue out=w2095:refnum<queue>, error out=w2097:errorcluster)  [unwired: 1 out]
            n698 = Enqueue Element(queue=w2092, element=5 ("元素"), error in (no error)=w2097) -> (queue out=w2088:refnum<queue>, error out=w2096:errorcluster)  [unwired: 1 in, 1 out]
            n699 = Flush Queue(queue=w2087) -> (queue out=w2085:refnum<queue>)  [unwired: 1 in, 2 out]
            n700 = Enqueue Element(queue=w2095, element=T8."MotorStop" ("元素"), error in (no error)=w2096) -> (queue out=w2090:refnum<queue>, error out=w2089:errorcluster)  [unwired: 1 in, 1 out]
          }
          frame #1 {
            n701 = Enqueue Element(queue=w2109, element=6 ("元素"), error in (no error)=w2108) -> (error out=w2107:errorcluster)  [unwired: 1 in, 2 out]
            n702 = Enqueue Element(queue=w2106, element=T8."MotorStop" ("元素"), error in (no error)=w2107) -> (queue out=w2100:refnum<queue>, error out=w2101:errorcluster)  [unwired: 1 in, 1 out]
          }
          frame #2 {
            n703 = call "QueueSolenAdv.vi"("Statue_IN"=w2118, "PlatNum_IN"=w2117, "Statue_Value"=0, "PlatNum_Value"=2, "错误输入（无错误）"=w2114) -> ("错误输出"=w2113:errorcluster)  [unwired: 8 in, 2 out]
            n704 = Enqueue Element(queue=w2112, element=T4."SolenAdv" ("元素"), error in (no error)=w2113) -> (error out=w2110:errorcluster)  [unwired: 1 in, 2 out]
          }
          frame #3 {
            n705 = Wait (ms)(milliseconds to wait=u32 200 ("等待时间（毫秒）")) -> ()  [unwired: 1 out]
          }
          frame #4 {
            n706 = property on="Plat3StopBtn" class="Bool (严格)"("Value"=FALSE ("Plat3StopBtn")) -> ()  [unwired: 2 in, 2 out]
          }
        }
      }
    }
  }
  n707 = while "Plat1-While循环" {
    tunnel: w28 -> [w2132]
    tunnel: w27 -> [w2131]
    tunnel: w36 -> [w2130]
    tunnel: w35 -> [w2129]
    tunnel: w34 -> [w2128]
    tunnel: w30 -> [w2127]
    tunnel: w26 -> [w2126]
    tunnel: w37 -> [w2125]
    tunnel: w29 -> [w2124]
    tunnel: w33 -> [w2123]
    tunnel: w32 -> [w2122]
    tunnel: w31 -> [w2121]
    stop <- FALSE stop-if-true
    n708 = event shown="[2] \"Plat1StopBtn\": 值改变" {
      selector: _ -> [_ _ _]
      dyn-events: _ -> [_ _ _]
      timeout: _ -> [_ _ _]
      tunnel: w2132 -> [_ w2203 _]
      tunnel: w2131 -> [_ w2201 _]
      tunnel: w2130 -> [_ w2206 _]
      tunnel: w2129 -> [_ w2205 _]
      tunnel: w2128 -> [_ w2204 _]
      tunnel: w2127 -> [_ w2199 w2495]
      tunnel: w2126 -> [_ w2197 _]
      tunnel: w2125 -> [_ w2207 _]
      tunnel: w2124 -> [_ w2196 w2497]
      tunnel: w2123 -> [_ w2194 _]
      tunnel: w2122 -> [_ w2192 _]
      tunnel: w2121 -> [_ w2190 w2496]
      event Timeout {
        n709 = event-data() -> ()  [unwired: 1 in, 2 out]
      }
      event "Plat1Btn": Value Change {
        w2138 = 0
        n710 = event-data() -> ()  [unwired: 1 in, 5 out]
        n711 = Flush Queue(queue=w2207) -> ()  [unwired: 1 in, 3 out]
        n712 = Flush Queue(queue=w2197) -> ()  [unwired: 1 in, 3 out]
        n713 = local write "Collection_Color"(0) -> ()
        n714 = local write "Property_T"("") -> ()
        n715 = local write "Red_Last"(w2138) -> ()
        n716 = local write "Green_Last"(w2138) -> ()
        n717 = local write "Blue_Last"(w2138) -> ()
        n718 = Flush Queue(queue=w2206) -> (queue out=w2146:refnum<queue>)  [unwired: 1 in, 2 out]
        n719 = Flush Queue(queue=w2205) -> (queue out=w2145:refnum<queue>)  [unwired: 1 in, 2 out]
        n720 = Flush Queue(queue=w2204) -> (queue out=w2144:refnum<queue>)  [unwired: 1 in, 2 out]
        n721 = control-ref of="SensorWait"() -> (w2141:refnum<vi>)
        n722 = control-ref of="Plat1StopBtn"() -> (w2148:refnum<vi>)
        n723 = control-ref of="Plat1SelectPolic1"() -> (w2136:refnum<vi>)
        n724 = control-ref of="Plat1SelectPolic2"() -> (w2135:refnum<vi>)
        n725 = control-ref of="Sensor array output"() -> (w2147:refnum<vi>)
        n726 = control-ref of="Plat1_FeedMotorSpeed"() -> (w2187:refnum<vi>)
        n727 = property class="DigNum (严格)"(reference=w2187) -> (error out=w2185:errorcluster, "Value"=w2186:i32)  [unwired: 1 in, 1 out]
        n728 = Flush Queue(queue=w2203) -> (queue out=w2202:refnum<queue>)  [unwired: 1 in, 2 out]
        n729 = Flush Queue(queue=w2201) -> (queue out=w2200:refnum<queue>)  [unwired: 1 in, 2 out]
        n730 = control-ref of="motor statue array output"() -> (w2139:refnum<vi>)
        n731 = control-ref of="platformStatue0 output"() -> (w2134:refnum<vi>)
        n732 = call "SetSpeedQueue.vi"("MotorNum队列"=w2202, "MotorSpeed队列"=w2200, "MotorNum元素"=1, "MotorSpeed元素"=w2186, "错误输入（无错误）"=w2185) -> ("错误输出"=w2184:errorcluster)  [unwired: 8 in, 2 out]
        n733 = Flush Queue(queue=w2196) -> (queue out=w2195:refnum<queue>)  [unwired: 1 in, 2 out]
        n734 = Enqueue Element(queue=w2195, element=T4."SetMotorSpeed" ("元素"), error in (no error)=w2184) -> (queue out=w2181:refnum<queue>, error out=w2182:errorcluster)  [unwired: 1 in, 1 out]
        n735 = Flush Queue(queue=w2190) -> (queue out=w2189:refnum<queue>)  [unwired: 1 in, 2 out]
        n736 = Flush Queue(queue=w2199) -> (queue out=w2198:refnum<queue>)  [unwired: 1 in, 2 out]
        n737 = Enqueue Element(queue=w2181, element=T4."FeedMotorStop" ("元素"), error in (no error)=w2182) -> (queue out=w2175:refnum<queue>, error out=w2179:errorcluster)  [unwired: 1 in, 1 out]
        n738 = call "QueueSolenAdv.vi"("Statue_IN"=w2189, "PlatNum_IN"=w2198, "Statue_Value"=0, "PlatNum_Value"=0, "错误输入（无错误）"=w2179) -> ("错误输出"=w2176:errorcluster)  [unwired: 8 in, 2 out]
        n739 = Flush Queue(queue=w2194) -> (queue out=w2193:refnum<queue>)  [unwired: 1 in, 2 out]
        n740 = Flush Queue(queue=w2192) -> (queue out=w2191:refnum<queue>)  [unwired: 1 in, 2 out]
        n741 = Enqueue Element(queue=w2175, element=T4."SolenAdv" ("元素"), error in (no error)=w2176) -> (queue out=w2170:refnum<queue>, error out=w2173:errorcluster)  [unwired: 1 in, 1 out]
        n742 = call "QueueSolenAct.vi"("SolenNum_IN"=w2193, "SolenStatue_IN"=w2191, "SolenNum_Value"=3, "SolenStatue_Value"=1, "错误输入（无错误）"=w2173) -> ("SolenNum_OUT"=w2163:refnum<queue>, "SolenStatue_OUT"=w2162:refnum<queue>, "错误输出"=w2169:errorcluster)  [unwired: 8 in]
        n743 = Enqueue Element(queue=w2170, element=T4."SolenAction" ("元素"), error in (no error)=w2169) -> (queue out=w2158:refnum<queue>, error out=w2167:errorcluster)  [unwired: 1 in, 1 out]
        n744 = call "Check.vi"("错误输入（无错误）"=w2167, "长度"=1, "索引"=3, "Array引用"=w2134, "Bool引用"=w2148) -> ("错误输出"=w2164:errorcluster)  [unwired: 6 in]
        n745 = call "QueueSolenAct.vi"("SolenNum_IN"=w2163, "SolenStatue_IN"=w2162, "SolenNum_Value"=1, "SolenStatue_Value"=1, "错误输入（无错误）"=w2164) -> ("SolenNum_OUT"=w2150:refnum<queue>, "SolenStatue_OUT"=w2149:refnum<queue>, "错误输出"=w2159:errorcluster)  [unwired: 8 in]
        n746 = Enqueue Element(queue=w2158, element=T4."SolenAction" ("元素"), error in (no error)=w2159) -> (queue out=w2151:refnum<queue>, error out=w2156:errorcluster)  [unwired: 1 in, 1 out]
        n747 = call "Check.vi"("错误输入（无错误）"=w2156, "长度"=1, "索引"=1, "Array引用"=w2134, "Bool引用"=w2148) -> ("错误输出"=w2153:errorcluster)  [unwired: 6 in]
        n748 = control-ref of="2to3Pos"() -> (w2142:refnum<vi>)
        n749 = control-ref of="1to2pos"() -> (w2143:refnum<vi>)
        n750 = while {
          tunnel: w2153 -> [_]
          shift-right: [w2213] -> _
          shift-left: enum16{"推料检测", "选料运输"}."推料检测" -> [w2225]
          tunnel: w2151 -> [w2224]
          tunnel: w2150 -> [w2223]
          tunnel: w2149 -> [w2222]
          tunnel: w2148 -> [w2221]
          tunnel: w2147 -> [w2220]
          tunnel: w2146 -> [w2219]
          tunnel: w2145 -> [w2218]
          tunnel: w2144 -> [w2217]
          tunnel: w2143 -> [w2216]
          tunnel: w2142 -> [w2215]
          tunnel: w2141 -> [w2214]
          tunnel: w2139 -> [w2211]
          tunnel: w2136 -> [w2210]
          tunnel: w2135 -> [w2209]
          tunnel: w2134 -> [w2208]
          stop <- w2212 stop-if-true
          n751 = case shown="\"选料运输\"" w2225 {
            tunnel: w2224 -> [w2291 w2311]
            tunnel: w2223 -> [w2289 w2315]
            tunnel: w2222 -> [w2288 w2314]
            tunnel: w2221 -> [w2235 w2318]
            tunnel: w2220 -> [w2280 w2317]
            tunnel: w2219 -> [w2266 _]
            tunnel: w2218 -> [w2265 _]
            tunnel: w2217 -> [w2264 _]
            tunnel: w2216 -> [w2261 _]
            tunnel: w2215 -> [w2250 _]
            tunnel: w2214 -> [w2244 _]
            tunnel: [w2240 w2312] -> w2213
            tunnel: w2211 -> [w2232 _]
            tunnel: w2210 -> [_ w2320]
            tunnel: w2209 -> [_ w2319]
            tunnel: w2208 -> [_ w2316]
            frame "推料检测", Default {
              n752 = property class="DigNum (严格)"(reference=w2244) -> ("Value"=w2243:i32)  [unwired: 1 in, 2 out]
              n753 = property class="DigNum (严格)"(reference=w2250) -> ("Value"=w2249:i32)  [unwired: 1 in, 2 out]
              n754 = property class="DigNum (严格)"(reference=w2244) -> ("Value"=w2255:i32)  [unwired: 1 in, 2 out]
              n755 = property class="DigNum (严格)"(reference=w2261) -> ("Value"=w2260:i32)  [unwired: 1 in, 2 out]
              n756 = Enqueue Element(queue=w2291, element=T4."FeedMotorStart" ("元素")) -> (queue out=w2284:refnum<queue>, error out=w2287:errorcluster)  [unwired: 2 in, 1 out]
              n757 = call "QueueSolenAct.vi"("SolenNum_IN"=w2289, "SolenStatue_IN"=w2288, "SolenNum_Value"=5, "SolenStatue_Value"=1, "错误输入（无错误）"=w2287) -> ("SolenNum_OUT"=w2274:refnum<queue>, "SolenStatue_OUT"=w2273:refnum<queue>, "错误输出"=w2283:errorcluster)  [unwired: 8 in]
              n758 = Enqueue Element(queue=w2284, element=T4."SolenAction" ("元素"), error in (no error)=w2283) -> (queue out=w2276:refnum<queue>, error out=w2281:errorcluster)  [unwired: 1 in, 1 out]
              n759 = call "CheckTure.vi"("Bool引用"=w2235, "Array引用"=w2280, "索引"=2, "长度"=1, "错误输入（无错误）"=w2281) -> ("错误输出"=w2277:errorcluster)  [unwired: 10 in]
              n760 = Enqueue Element(queue=w2276, element=T4."FeedMotorStop" ("元素"), error in (no error)=w2277) -> (queue out=w2269:refnum<queue>, error out=w2272:errorcluster)  [unwired: 1 in, 1 out]
              n761 = call "QueueSolenAct.vi"("SolenNum_IN"=w2274, "SolenStatue_IN"=w2273, "SolenNum_Value"=5, "SolenStatue_Value"=0, "错误输入（无错误）"=w2272) -> ("错误输出"=w2268:errorcluster)  [unwired: 8 in, 2 out]
              n762 = Enqueue Element(queue=w2269, element=T4."SolenAction" ("元素"), error in (no error)=w2268) -> (queue out=w2257:refnum<queue>, error out=w2259:errorcluster)  [unwired: 1 in, 1 out]
              n763 = call "QueueMotorStart.vi"("MotorNum"=w2266, "Step"=w2265, "Direction"=w2264, "错误输入（无错误）"=w2259, "MotorNum_Int"=1, "Step_Int"=w2260, "Direction_Int"=0) -> ("MotorNum_OUT"=w2254:refnum<queue>, "Step_OUT"=w2253:refnum<queue>, "Direction_OUT"=w2252:refnum<queue>, "错误输出"=w2258:errorcluster)  [unwired: 9 in]
              n764 = Enqueue Element(queue=w2257, element=T4."MotorStart" ("元素"), error in (no error)=w2258) -> (queue out=w2246:refnum<queue>, error out=w2239:errorcluster)  [unwired: 1 in, 1 out]
              n765 = call "Check.vi"("错误输入（无错误）"=w2239, "长度"=1, "索引"=0, "Array引用"=w2232, "Bool引用"=w2235) -> ("错误输出"=w2238:errorcluster)  [unwired: 6 in]
              n766 = call "DelayPlat3.vi"("error In"=w2238, "DelayTime"=w2255, "Bool"=w2235) -> ("error Out"=w2242:errorcluster)  [unwired: 8 in]
              n767 = flat-sequence {
                tunnel: w2242 -> [w2310]
                tunnel: [w2310] -> w2241
                frame #0 {
                  n768 = local read "Green"() -> (w2307:i32)
                  n769 = local read "Blue"() -> (w2303:i32)
                  n770 = local read "Red"() -> (w2309:i32)
                  n771 = local write "Red_Last"(w2309) -> ()
                  n772 = local write "Green_Last"(w2307) -> ()
                  n773 = local write "Blue_Last"(w2303) -> ()
                  n774 = Multiply(x=w2307, y=256) -> (x*y=w2304:i32)
                  n775 = Multiply(x=w2309, y=65536) -> (x*y=w2305:i32)
                  n776 = Add(x=w2305, y=w2304) -> (x+y=w2302:i32)
                  n777 = Add(x=w2302, y=w2303) -> (x+y=w2301:i32)
                  n778 = local write "Collection_Color"(w2301) -> ()
                }
              }
              n779 = call "QueueMotorStart.vi"("MotorNum"=w2254, "Step"=w2253, "Direction"=w2252, "错误输入（无错误）"=w2241, "MotorNum_Int"=1, "Step_Int"=w2249, "Direction_Int"=0) -> ("错误输出"=w2247:errorcluster)  [unwired: 9 in, 3 out]
              n780 = Enqueue Element(queue=w2246, element=T4."MotorStart" ("元素"), error in (no error)=w2247) -> (queue out=w2228:refnum<queue>, error out=w2237:errorcluster)  [unwired: 1 in, 1 out]
              n781 = call "Check.vi"("错误输入（无错误）"=w2237, "长度"=1, "索引"=0, "Array引用"=w2232, "Bool引用"=w2235) -> ("错误输出"=w2236:errorcluster)  [unwired: 6 in]
              n782 = call "DelayPlat3.vi"("error In"=w2236, "DelayTime"=w2243, "Bool"=w2235) -> ("error Out"=w2229:errorcluster)  [unwired: 8 in]
              n783 = flat-sequence {
                tunnel: w2229 -> [w2292]
                tunnel: w2228 -> [w2293]
                tunnel: [w2293] -> w2227
                tunnel: [w2292] -> w2226
                tunnel: w2227 -> [w2299]
                tunnel: w2226 -> [w2298]
                tunnel: [enum16{"推料检测", "选料运输"}."选料运输"] -> w2240
                frame #0 {
                  n784 = local read "电涡流电平"() -> (w2294:i32)
                  n785 = case shown="1" w2294 {
                    frame 0, Default {
                      n786 = local write "Property_T"("非磁性") -> ()
                    }
                    frame 1 {
                      n787 = local write "Property_T"("磁性") -> ()
                    }
                  }
                }
                frame #1 {
                  n788 = Enqueue Element(queue=w2299, element=T4."FeedMotorStart" ("元素"), error in (no error)=w2298) -> ()  [unwired: 1 in, 3 out]
                }
                frame #2 {
                }
              }
            }
            frame "选料运输" {
              n789 = while {
                shift-right: [w2334] -> w2313
                shift-left: T9."初始化选择器" -> [w2327]
                tunnel: w2320 -> [w2336]
                tunnel: w2319 -> [w2335]
                tunnel: w2318 -> [w2333]
                tunnel: w2317 -> [w2332]
                tunnel: w2316 -> [w2331]
                tunnel: w2311 -> [w2330]
                tunnel: w2315 -> [w2329]
                tunnel: w2314 -> [w2328]
                stop <- w2323 stop-if-true
                n790 = case shown="\"1号料槽选料\"" w2327 {
                  tunnel: w2336 -> [w2341 _ _ _]
                  tunnel: w2335 -> [w2337 _ _ _]
                  tunnel: [w2338 w2458 w2467 w2474] -> w2334
                  tunnel: w2333 -> [_ w2453 w2472 w2481]
                  tunnel: w2332 -> [_ w2461 w2471 w2480]
                  tunnel: w2331 -> [_ _ _ w2479]
                  tunnel: w2330 -> [_ w2457 w2466 w2478]
                  tunnel: w2329 -> [_ w2460 w2470 w2477]
                  tunnel: w2328 -> [_ w2459 w2469 w2476]
                  frame "初始化选择器", Default {
                    n791 = property class="CmbBox"(reference=w2341) -> ("Value"=w2340:string)  [unwired: 1 in, 2 out]
                    n792 = Decimal String To Number(string=w2340) -> (number=w2339:i32)  [unwired: 2 in, 1 out]
                    n793 = case shown="0, 默认" w2339 {
                      tunnel: [w2343 w2371 w2400 w2429] -> w2338
                      tunnel: w2337 -> [w2342 w2373 w2401 w2430]
                      frame 0, Default {
                        n794 = local read "Property_T"() -> (w2346:string)
                        n795 = Equal?(x=w2346, y="非磁性") -> (x = y?=w2344:bool)
                        n796 = case shown="假" w2344 {
                          tunnel: [w2347 enum16{"初始化选择器", "1号料槽选料", "2号料槽选料", "取料动作"}."1号料槽选料"] -> w2343
                          tunnel: w2342 -> [w2350 _]
                          frame False {
                            n797 = property class="CmbBox"(reference=w2350) -> ("Value"=w2349:string)  [unwired: 1 in, 2 out]
                            n798 = Decimal String To Number(string=w2349) -> (number=w2348:i32)  [unwired: 2 in, 1 out]
                            n799 = case shown="2" w2348 {
                              tunnel: [w2351 w2357 w2363 enum16{"初始化选择器", "1号料槽选料", "2号料槽选料", "取料动作"}."取料动作"] -> w2347
                              frame 0, Default {
                                n800 = local read "Property_T"() -> (w2353:string)
                                n801 = Equal?(x=w2353, y="非磁性") -> (x = y?=w2352:bool)
                                n802 = case shown="真" w2352 {
                                tunnel: [enum16{"初始化选择器", "1号料槽选料", "2号料槽选料", "取料动作"}."取料动作" enum16{"初始化选择器", "1号料槽选料", "2号料槽选料", "取料动作"}."2号料槽选料"] -> w2351
                                frame False {
                                }
                                frame True {
                                }
                                }
                              }
                              frame 1 {
                                n803 = local read "Property_T"() -> (w2359:string)
                                n804 = Equal?(x=w2359, y="磁性") -> (x = y?=w2358:bool)
                                n805 = case shown="假" w2358 {
                                tunnel: [enum16{"初始化选择器", "1号料槽选料", "2号料槽选料", "取料动作"}."取料动作" enum16{"初始化选择器", "1号料槽选料", "2号料槽选料", "取料动作"}."2号料槽选料"] -> w2357
                                frame False {
                                }
                                frame True {
                                }
                                }
                              }
                              frame 2 {
                                n806 = local read "Blue_Last"() -> (w2366:i32)
                                n807 = Greater?(x=w2366, y=100) -> (0:w2364:bool)
                                n808 = case shown="真" w2364 {
                                tunnel: [enum16{"初始化选择器", "1号料槽选料", "2号料槽选料", "取料动作"}."取料动作" enum16{"初始化选择器", "1号料槽选料", "2号料槽选料", "取料动作"}."2号料槽选料"] -> w2363
                                frame False {
                                }
                                frame True {
                                }
                                }
                              }
                              frame 3 {
                              }
                            }
                          }
                          frame True {
                          }
                        }
                      }
                      frame 1 {
                        n809 = local read "Property_T"() -> (w2375:string)
                        n810 = Equal?(x=w2375, y="磁性") -> (x = y?=w2372:bool)
                        n811 = case shown="假" w2372 {
                          tunnel: [w2376 enum16{"初始化选择器", "1号料槽选料", "2号料槽选料", "取料动作"}."1号料槽选料"] -> w2371
                          tunnel: w2373 -> [w2379 _]
                          frame False {
                            n812 = property class="CmbBox"(reference=w2379) -> ("Value"=w2378:string)  [unwired: 1 in, 2 out]
                            n813 = Decimal String To Number(string=w2378) -> (number=w2377:i32)  [unwired: 2 in, 1 out]
                            n814 = case shown="0, 默认" w2377 {
                              tunnel: [w2380 w2386 w2392 enum16{"初始化选择器", "1号料槽选料", "2号料槽选料", "取料动作"}."取料动作"] -> w2376
                              frame 0, Default {
                                n815 = local read "Property_T"() -> (w2382:string)
                                n816 = Equal?(x=w2382, y="非磁性") -> (x = y?=w2381:bool)
                                n817 = case shown="真" w2381 {
                                tunnel: [enum16{"初始化选择器", "1号料槽选料", "2号料槽选料", "取料动作"}."取料动作" enum16{"初始化选择器", "1号料槽选料", "2号料槽选料", "取料动作"}."2号料槽选料"] -> w2380
                                frame False {
                                }
                                frame True {
                                }
                                }
                              }
                              frame 1 {
                                n818 = local read "Property_T"() -> (w2388:string)
                                n819 = Equal?(x=w2388, y="磁性") -> (x = y?=w2387:bool)
                                n820 = case shown="假" w2387 {
                                tunnel: [enum16{"初始化选择器", "1号料槽选料", "2号料槽选料", "取料动作"}."取料动作" enum16{"初始化选择器", "1号料槽选料", "2号料槽选料", "取料动作"}."2号料槽选料"] -> w2386
                                frame False {
                                }
                                frame True {
                                }
                                }
                              }
                              frame 2 {
                                n821 = local read "Blue_Last"() -> (w2395:i32)
                                n822 = Greater?(x=w2395, y=100) -> (0:w2393:bool)
                                n823 = case shown="真" w2393 {
                                tunnel: [enum16{"初始化选择器", "1号料槽选料", "2号料槽选料", "取料动作"}."取料动作" enum16{"初始化选择器", "1号料槽选料", "2号料槽选料", "取料动作"}."2号料槽选料"] -> w2392
                                frame False {
                                }
                                frame True {
                                }
                                }
                              }
                              frame 3 {
                              }
                            }
                          }
                          frame True {
                          }
                        }
                      }
                      frame 2 {
                        n824 = local read "Blue_Last"() -> (w2403:i32)
                        n825 = Greater?(x=w2403, y=100) -> (0:w2402:bool)
                        n826 = case shown="假" w2402 {
                          tunnel: [w2405 enum16{"初始化选择器", "1号料槽选料", "2号料槽选料", "取料动作"}."1号料槽选料"] -> w2400
                          tunnel: w2401 -> [w2408 _]
                          frame False {
                            n827 = property class="CmbBox"(reference=w2408) -> ("Value"=w2407:string)  [unwired: 1 in, 2 out]
                            n828 = Decimal String To Number(string=w2407) -> (number=w2406:i32)  [unwired: 2 in, 1 out]
                            n829 = case shown="0, 默认" w2406 {
                              tunnel: [w2409 w2415 w2421 enum16{"初始化选择器", "1号料槽选料", "2号料槽选料", "取料动作"}."取料动作"] -> w2405
                              frame 0, Default {
                                n830 = local read "Property_T"() -> (w2411:string)
                                n831 = Equal?(x=w2411, y="非磁性") -> (x = y?=w2410:bool)
                                n832 = case shown="真" w2410 {
                                tunnel: [enum16{"初始化选择器", "1号料槽选料", "2号料槽选料", "取料动作"}."取料动作" enum16{"初始化选择器", "1号料槽选料", "2号料槽选料", "取料动作"}."2号料槽选料"] -> w2409
                                frame False {
                                }
                                frame True {
                                }
                                }
                              }
                              frame 1 {
                                n833 = local read "Property_T"() -> (w2417:string)
                                n834 = Equal?(x=w2417, y="磁性") -> (x = y?=w2416:bool)
                                n835 = case shown="假" w2416 {
                                tunnel: [enum16{"初始化选择器", "1号料槽选料", "2号料槽选料", "取料动作"}."取料动作" enum16{"初始化选择器", "1号料槽选料", "2号料槽选料", "取料动作"}."2号料槽选料"] -> w2415
                                frame False {
                                }
                                frame True {
                                }
                                }
                              }
                              frame 2 {
                                n836 = local read "Blue_Last"() -> (w2424:i32)
                                n837 = Greater?(x=w2424, y=100) -> (0:w2422:bool)
                                n838 = case shown="真" w2422 {
                                tunnel: [enum16{"初始化选择器", "1号料槽选料", "2号料槽选料", "取料动作"}."取料动作" enum16{"初始化选择器", "1号料槽选料", "2号料槽选料", "取料动作"}."2号料槽选料"] -> w2421
                                frame False {
                                }
                                frame True {
                                }
                                }
                              }
                              frame 3 {
                              }
                            }
                          }
                          frame True {
                          }
                        }
                      }
                      frame 3 {
                        n839 = property class="CmbBox"(reference=w2430) -> ("Value"=w2432:string)  [unwired: 1 in, 2 out]
                        n840 = Decimal String To Number(string=w2432) -> (number=w2431:i32)  [unwired: 2 in, 1 out]
                        n841 = case shown="1" w2431 {
                          tunnel: [w2433 w2439 w2445 enum16{"初始化选择器", "1号料槽选料", "2号料槽选料", "取料动作"}."取料动作"] -> w2429
                          frame 0, Default {
                            n842 = local read "Property_T"() -> (w2435:string)
                            n843 = Equal?(x=w2435, y="非磁性") -> (x = y?=w2434:bool)
                            n844 = case shown="真" w2434 {
                              tunnel: [enum16{"初始化选择器", "1号料槽选料", "2号料槽选料", "取料动作"}."取料动作" enum16{"初始化选择器", "1号料槽选料", "2号料槽选料", "取料动作"}."2号料槽选料"] -> w2433
                              frame False {
                              }
                              frame True {
                              }
                            }
                          }
                          frame 1 {
                            n845 = local read "Property_T"() -> (w2441:string)
                            n846 = Equal?(x=w2441, y="磁性") -> (x = y?=w2440:bool)
                            n847 = case shown="假" w2440 {
                              tunnel: [enum16{"初始化选择器", "1号料槽选料", "2号料槽选料", "取料动作"}."取料动作" enum16{"初始化选择器", "1号料槽选料", "2号料槽选料", "取料动作"}."2号料槽选料"] -> w2439
                              frame False {
                              }
                              frame True {
                              }
                            }
                          }
                          frame 2 {
                            n848 = local read "Blue_Last"() -> (w2448:i32)
                            n849 = Greater?(x=w2448, y=100) -> (0:w2446:bool)
                            n850 = case shown="真" w2446 {
                              tunnel: [enum16{"初始化选择器", "1号料槽选料", "2号料槽选料", "取料动作"}."取料动作" enum16{"初始化选择器", "1号料槽选料", "2号料槽选料", "取料动作"}."2号料槽选料"] -> w2445
                              frame False {
                              }
                              frame True {
                              }
                            }
                          }
                          frame 3 {
                          }
                        }
                      }
                    }
                  }
                  frame "1号料槽选料" {
                    n851 = Enqueue Element(queue=w2457, element=T4."FeedMotorStop" ("元素")) -> (queue out=w2456:refnum<queue>, error out=w2455:errorcluster)  [unwired: 2 in, 1 out]
                    n852 = call "FirstDumper_Enable.vi"("StopBool引用"=w2453, "SensorArray引用"=w2461, "Cmd"=w2456, "SolenNum_IN"=w2460, "SolenStatue_IN"=w2459, "错误输入（无错误）"=w2455) -> ("错误输出"=w2452:errorcluster)  [unwired: 10 in, 3 out]
                    n853 = flat-sequence {
                      tunnel: [T9."Stop"] -> w2458
                      tunnel: w2452 -> [_]
                      frame #0 {
                      }
                    }
                  }
                  frame "2号料槽选料" {
                    n854 = Enqueue Element(queue=w2466, element=T4."FeedMotorStop" ("元素")) -> (queue out=w2465:refnum<queue>, error out=w2464:errorcluster)  [unwired: 2 in, 1 out]
                    n855 = call "SecondDumper_Enable.vi"("StopBool引用"=w2472, "SensorArray引用"=w2471, "Cmd"=w2465, "SolenNum_IN"=w2470, "SolenStatue_IN"=w2469, "错误输入（无错误）"=w2464) -> ("错误输出"=w2468:errorcluster)  [unwired: 10 in, 3 out]
                    n856 = flat-sequence {
                      tunnel: w2468 -> [_]
                      tunnel: [T9."Stop"] -> w2467
                      frame #0 {
                      }
                    }
                  }
                  frame "取料动作" {
                    n857 = call "Plat1Take.vi"("StopBtnBool引用"=w2481, "SensorArray引用"=w2480, "Plat1StatueArray引用"=w2479, "Cmd"=w2478, "SolenNum_IN"=w2477, "SolenStatue_IN"=w2476) -> ("错误输出"=w2475:errorcluster)  [unwired: 10 in, 3 out]
                    n858 = flat-sequence {
                      tunnel: w2475 -> [_]
                      tunnel: [T9."Stop"] -> w2474
                      frame #0 {
                      }
                    }
                  }
                }
                n859 = Equal?(x=w2327, y=T9."Stop") -> (x = y?=w2325:bool)
                n860 = local read "Plat1StopBtn"() -> (w2324:bool)
                n861 = Or(x=w2325, y=w2324) -> (x .or. y?=w2323:bool)
              }
              n862 = flat-sequence {
                tunnel: w2313 -> [_]
                tunnel: [enum16{"推料检测", "选料运输"}."推料检测"] -> w2312
                frame #0 {
                }
              }
            }
          }
          n863 = local read "Plat1StopBtn"() -> (w2212:bool)
        }
      }
      event "Plat1StopBtn": Value Change {
        n864 = event-data() -> ()  [unwired: 1 in, 5 out]
        n865 = Flush Queue(queue=w2495) -> (queue out=w2491:refnum<queue>)  [unwired: 1 in, 2 out]
        n866 = Flush Queue(queue=w2497) -> (queue out=w2494:refnum<queue>)  [unwired: 1 in, 2 out]
        n867 = Flush Queue(queue=w2496) -> (queue out=w2492:refnum<queue>)  [unwired: 1 in, 2 out]
        n868 = Enqueue Element(queue=w2494, element=T4."FeedMotorStop" ("元素")) -> (queue out=w2486:refnum<queue>, error out=w2490:errorcluster)  [unwired: 2 in, 1 out]
        n869 = call "QueueSolenAdv.vi"("Statue_IN"=w2492, "PlatNum_IN"=w2491, "Statue_Value"=0, "PlatNum_Value"=0, "错误输入（无错误）"=w2490) -> ("错误输出"=w2487:errorcluster)  [unwired: 8 in, 2 out]
        n870 = Enqueue Element(queue=w2486, element=T4."SolenAdv" ("元素"), error in (no error)=w2487) -> (error out=w2483:errorcluster)  [unwired: 1 in, 2 out]
        n871 = property on="Plat1StopBtn" class="Bool (严格)"(error in=w2483, "Value"=FALSE ("Plat1StopBtn")) -> ()  [unwired: 1 in, 2 out]
      }
    }
  }
  n872 = control-ref of="Plat2SelectPolicy"() -> (w97:refnum<vi>)
  n873 = case shown="真" w233 {
    tunnel: w232 -> [w2499 w2500]
    tunnel: w231 -> [w2498 w2502]
    tunnel: w230 -> [_ w2503]
    tunnel: [w2498 w2501] -> w220
    tunnel: [w2499 w2500] -> w221
    frame False {
    }
    frame True {
      n874 = property on="Horizontal2" class="DigNum (严格)"(error in=w2502, "Value"=w2503) -> (error out=w2501:errorcluster)  [unwired: 1 in, 1 out]
    }
  }
  n875 = control-ref of="Plat2SendX"() -> (w99:refnum<vi>)
  n876 = control-ref of="Plat2SendY"() -> (w98:refnum<vi>)
  n877 = control-ref of="Plat2RecvX"() -> (w101:refnum<vi>)
  n878 = control-ref of="Plat2RecvY"() -> (w100:refnum<vi>)
  n879 = call-poly <vilib>:"Read Key.vi"("section"=w146, "error in (no error)"=w220, "key"="X3Pos", "refnum"=w221) -> ("error out"=w226:errorcluster, "value"=w227:i32, "found?"=w229:bool, "refnum out"=w228:T5)  [unwired: 4 in]
  n880 = case shown="真" w229 {
    tunnel: w228 -> [w2505 w2507]
    tunnel: w227 -> [_ w2509]
    tunnel: w226 -> [w2504 w2508]
    tunnel: [w2505 w2507] -> w219
    tunnel: [w2504 w2506] -> w218
    frame False {
    }
    frame True {
      n881 = property on="Horizontal3" class="DigNum (严格)"(error in=w2508, "Value"=w2509) -> (error out=w2506:errorcluster)  [unwired: 1 in, 1 out]
    }
  }
  n882 = call-poly <vilib>:"Read Key.vi"("section"=w146, "error in (no error)"=w218, "key"="X4Pos", "refnum"=w219) -> ("error out"=w223:errorcluster, "value"=w222:i32, "found?"=w225:bool, "refnum out"=w224:T5)  [unwired: 4 in]
  n883 = while {
    tunnel: w365 -> [_]
    tunnel: w363 -> [_]
    tunnel: w362 -> [_]
    tunnel: w361 -> [_]
    tunnel: w353 -> [_]
    tunnel: w352 -> [_]
    tunnel: w349 -> [_]
    tunnel: w347 -> [_]
    tunnel: w29 -> [w2512]
    tunnel: w170 -> [w2511]
    tunnel: w343 -> [_]
    tunnel: w334 -> [_]
    tunnel: w333 -> [_]
    tunnel: w331 -> [_]
    tunnel: w330 -> [_]
    tunnel: w327 -> [_]
    tunnel: w325 -> [_]
    tunnel: "选项卡控件" -> [_]
    tunnel: "选项卡控件Next" -> [_]
    tunnel: w171 -> [_]
    stop <- FALSE stop-if-true
    n884 = event shown="[1] \"start\": 值改变" {
      selector: _ -> [_ _ _]
      dyn-events: _ -> [_ _ _]
      timeout: _ -> [_ _ _]
      tunnel: w2512 -> [_ w2519 w2635]
      tunnel: w2511 -> [_ w2518 w2634]
      event Timeout {
        n885 = event-data() -> ()  [unwired: 1 in, 2 out]
      }
      event "start": Value Change {
        n886 = event-data() -> ()  [unwired: 1 in, 5 out]
        n887 = Flush Queue(queue=w2519, error in (no error)=w2518) -> (queue out=w2517:refnum<queue>, error out=w2516:errorcluster)  [unwired: 1 out]
        n888 = call "API SYSINIT.vi"() -> ("SYSINIT return value"=w2520:bool)  [unwired: 11 in]
        n889 = property on="Statue" class="Bool (严格)"("Value"=w2520) -> (error out=w2515:errorcluster)  [unwired: 2 in, 1 out]
        n890 = call "ColorAPI_Init.vi"("错误输入（无错误）"=w2515, "端口号"=10) -> ("错误输出"=w2513:errorcluster)  [unwired: 7 in, 2 out]
        n891 = case shown="真" w2520 {
          tunnel: w2517 -> [_ w2530]
          tunnel: w2516 -> [_ w2529]
          tunnel: w2513 -> [_ _]
          frame False {
          }
          frame True {
            w2524 = T3."Enabled" ("禁用")
            w2533 = T3."Enabled" ("禁用")
            n892 = while {
              stop <- w2549 stop-if-true
              n893 = local read "stop"() -> (w2551:bool)
              n894 = call "ColorAPI_GetData.vi"() -> ("Blue"=w2541:i32, "Green"=w2546:i32, "Red"=w2548:i32)  [unwired: 8 in, 1 out]
              "Red" <- w2548
              "Green" <- w2546
              "Blue" <- w2541
              n895 = Wait (ms)(milliseconds to wait=u32 100 ("等待时间（毫秒）")) -> ()  [unwired: 1 out]
              n896 = And(x=w2551, y=TRUE) -> (x .and. y?=w2549:bool)
              n897 = Multiply(x=w2546, y=256) -> (x*y=w2543:i32)
              n898 = Multiply(x=w2548, y=65536) -> (x*y=w2544:i32)
              n899 = Add(x=w2544, y=w2543) -> (x+y=w2542:i32)
              n900 = Add(x=w2542, y=w2541) -> (x+y=w2540:i32)
              n901 = property on="颜色盒" class="ColBox"("Value"=w2540) -> ()  [unwired: 2 in, 2 out]
            }
            n902 = node-c288() -> (w2523:T11)  [unwired: 4 in]
            n903 = timed-loop {
              shift-right: [w2556] -> _
              shift-left: w2530 -> [w2564]
              shift-right: [w2555] -> _
              shift-left: w2529 -> [w2563]
              timing: w2523 -> [_]
              timing-out: [_] -> w2522
              stop <- w2552 stop-if-true
              n904 = node-c288() -> ()  [unwired: 1 in, 1 out]
              n905 = local read "stop"() -> (w2553:bool)
              n906 = And(x=w2553, y=TRUE) -> (x .and. y?=w2552:bool)
              n907 = Enqueue Element(queue=w2564, element=T10."RcvDataInit" ("元素"), error in (no error)=w2563) -> (queue out=w2566:refnum<queue>, error out=w2565:errorcluster)  [unwired: 1 in, 1 out]
              n908 = Enqueue Element(queue=w2566, element=T10."GetSensorStatue" ("元素"), error in (no error)=w2565) -> (queue out=w2574:refnum<queue>, error out=w2573:errorcluster)  [unwired: 1 in, 1 out]
              n909 = Enqueue Element(queue=w2574, element=T10."GetSensorAD" ("元素"), error in (no error)=w2573) -> (queue out=w2572:refnum<queue>, error out=w2571:errorcluster)  [unwired: 1 in, 1 out]
              n910 = Enqueue Element(queue=w2572, element=T10."GetSolenStatue" ("元素"), error in (no error)=w2571) -> (queue out=w2570:refnum<queue>, error out=w2569:errorcluster)  [unwired: 1 in, 1 out]
              n911 = Enqueue Element(queue=w2570, element=T10."GetPaltformStatue" ("元素"), error in (no error)=w2569) -> (queue out=w2568:refnum<queue>, error out=w2567:errorcluster)  [unwired: 1 in, 1 out]
              n912 = Enqueue Element(queue=w2568, element=T10."GetMotorStatue" ("元素"), error in (no error)=w2567) -> (queue out=w2556:refnum<queue>, error out=w2555:errorcluster)  [unwired: 1 in, 1 out]
              n913 = node-c288() -> ()  [unwired: 1 in, 1 out]
            }
            n914 = property on="stop" class="Bool (严格)"("DisabledEnum"=w2533) -> (error out=w2532:errorcluster)  [unwired: 2 in, 1 out]
            n915 = property on="restartbtn" class="Bool"(error in=w2532, "DisabledEnum"=w2533) -> (error out=w2531:errorcluster)  [unwired: 1 in, 1 out]
            n916 = while {
              shift-right: [w2592] -> _
              shift-left: 0 -> [w2594]
              shift-right: [w2593] -> _
              shift-left: enum16{"允许计数", "不允许计数"}."允许计数" -> [w2595]
              shift-right: [w2586] -> _
              shift-left: enum16{"允许计数", "不允许计数"}."允许计数" -> [w2588]
              shift-right: [w2585] -> _
              shift-left: 0 -> [w2587]
              stop <- w2589 stop-if-true
              n917 = case shown="\"不允许计数\"" w2588 {
                tunnel: w2587 -> [w2598 w2607]
                tunnel: [w2597 w2607] -> w2585
                tunnel: [w2596 w2608] -> w2586
                frame "允许计数", Default {
                  n918 = property on="红外电平" class="DigNum (严格)"() -> ("Value"=w2601:i32)  [unwired: 2 in, 2 out]
                  n919 = Greater?(x=w2601, y=0.5) -> (0:w2599:bool)
                  n920 = case shown="假" w2599 {
                    tunnel: w2598 -> [w2602 w2606]
                    tunnel: [w2602 w2605] -> w2597
                    tunnel: [enum16{"允许计数", "不允许计数"}."允许计数" enum16{"允许计数", "不允许计数"}."不允许计数"] -> w2596
                    frame False {
                    }
                    frame True {
                      n921 = Increment(x=w2606) -> (x+1=w2605:i32)
                    }
                  }
                }
                frame "不允许计数" {
                  n922 = property on="红外电平" class="DigNum (严格)"() -> ("Value"=w2611:i32)  [unwired: 2 in, 2 out]
                  n923 = Less?(x=w2611, y=0.5) -> (x < y?=w2609:bool)
                  n924 = case shown="假" w2609 {
                    tunnel: [enum16{"允许计数", "不允许计数"}."不允许计数" enum16{"允许计数", "不允许计数"}."允许计数"] -> w2608
                    frame False {
                    }
                    frame True {
                    }
                  }
                }
              }
              n925 = case shown="\"不允许计数\"" w2595 {
                tunnel: w2594 -> [w2616 w2625]
                tunnel: [w2615 w2625] -> w2592
                tunnel: [w2614 w2626] -> w2593
                frame "允许计数", Default {
                  n926 = property on="电涡流电平" class="DigNum (严格)"() -> ("Value"=w2619:i32)  [unwired: 2 in, 2 out]
                  n927 = Greater?(x=w2619, y=0.5) -> (0:w2617:bool)
                  n928 = case shown="假" w2617 {
                    tunnel: w2616 -> [w2620 w2624]
                    tunnel: [w2620 w2623] -> w2615
                    tunnel: [enum16{"允许计数", "不允许计数"}."允许计数" enum16{"允许计数", "不允许计数"}."不允许计数"] -> w2614
                    frame False {
                    }
                    frame True {
                      n929 = Increment(x=w2624) -> (x+1=w2623:i32)
                    }
                  }
                }
                frame "不允许计数" {
                  n930 = property on="电涡流电平" class="DigNum (严格)"() -> ("Value"=w2629:i32)  [unwired: 2 in, 2 out]
                  n931 = Less?(x=w2629, y=0.5) -> (x < y?=w2627:bool)
                  n932 = case shown="假" w2627 {
                    tunnel: [enum16{"允许计数", "不允许计数"}."不允许计数" enum16{"允许计数", "不允许计数"}."允许计数"] -> w2626
                    frame False {
                    }
                    frame True {
                    }
                  }
                }
              }
              n933 = local read "stop"() -> (w2591:bool)
              n934 = Wait (ms)(milliseconds to wait=u32 10 ("等待时间（毫秒）")) -> ()  [unwired: 1 out]
              n935 = property on="电桥电平_Event" class="DigNum (严格)"() -> ("Value"=w2583:dbl)  [unwired: 2 in, 2 out]
              n936 = And(x=w2591, y=TRUE) -> (x .and. y?=w2589:bool)
              n937 = property on="KCurrent" class="DigNum (严格)"() -> ("Value"=w2582:dbl)  [unwired: 2 in, 2 out]
              n938 = Multiply(x=w2583, y=w2582) -> (x*y=w2581:dbl)
              n939 = property on="BCurrent" class="DigNum (严格)"() -> ("Value"=w2580:dbl)  [unwired: 2 in, 2 out]
              n940 = Add(x=w2581, y=w2580) -> (x+y=w2579:dbl)
              n941 = property on="Stog" class="DigNum (严格)"("Value"=w2579) -> ()  [unwired: 2 in, 2 out]
              n942 = property on="红外计数" class="DigNum (严格)"("Value"=w2585) -> ()  [unwired: 2 in, 2 out]
              n943 = property on="电涡流计数" class="DigNum (严格)"("Value"=w2592) -> ()  [unwired: 2 in, 2 out]
            }
            n944 = property on="start" class="Bool"(error in=w2531, "DisabledEnum"=T3."Disabled and Grayed Out" ("禁用")) -> (error out=w2521:errorcluster)  [unwired: 1 in, 1 out]
            n945 = property on="No1Btn" class="Bool"(error in=w2521, "DisabledEnum"=w2524) -> (error out=w2528:errorcluster)  [unwired: 1 in, 1 out]
            n946 = property on="No2Btn" class="Bool"(error in=w2528, "DisabledEnum"=w2524) -> (error out=w2527:errorcluster)  [unwired: 1 in, 1 out]
            n947 = property on="No3Btn" class="Bool"(error in=w2527, "DisabledEnum"=w2524) -> (error out=w2526:errorcluster)  [unwired: 1 in, 1 out]
            n948 = property on="BaseBtn" class="Bool"(error in=w2526, "DisabledEnum"=w2524) -> (error out=w2525:errorcluster)  [unwired: 1 in, 1 out]
            n949 = property on="MotinAdv" class="Bool"(error in=w2525, "DisabledEnum"=w2524) -> ()  [unwired: 1 in, 2 out]
            n950 = node-c288(w2522) -> ()  [unwired: 1 out]
          }
        }
      }
      event "stop": Value Change {
        n951 = event-data() -> ()  [unwired: 1 in, 5 out]
        n952 = flat-sequence {
          tunnel: w2634 -> [w2637]
          tunnel: w2635 -> [w2638]
          tunnel: [w2638] -> w2633
          tunnel: [w2637] -> w2632
          tunnel: w2633 -> [w2640]
          tunnel: w2632 -> [w2639]
          frame #0 {
            n953 = Wait (ms)(milliseconds to wait=u32 200 ("等待时间（毫秒）")) -> ()  [unwired: 1 out]
          }
          frame #1 {
            n954 = Flush Queue(queue=w2640, error in (no error)=w2639) -> ()  [unwired: 3 out]
          }
          frame #2 {
            w2641 = T3."Disabled and Grayed Out" ("禁用")
            (unwired) T3."Enabled" ("禁用")
            n955 = property on="start" class="Bool"("DisabledEnum"=T3."Enabled" ("禁用")) -> (error out=w2652:errorcluster)  [unwired: 2 in, 1 out]
            n956 = property on="restartbtn" class="Bool"("DisabledEnum"=w2641) -> (error out=w2648:errorcluster)  [unwired: 2 in, 1 out]
            n957 = property on="stop" class="Bool (严格)"(error in=w2652, "DisabledEnum"=T3."Disabled and Grayed Out" ("禁用")) -> (error out=w2649:errorcluster)  [unwired: 1 in, 1 out]
            n958 = property on="stop" class="Bool (严格)"(error in=w2649, "Value"=FALSE ("stop")) -> ()  [unwired: 1 in, 2 out]
            n959 = property on="Statue" class="Bool (严格)"(error in=w2648, "Value"=FALSE ("Statue")) -> (error out=w2646:errorcluster)  [unwired: 1 in, 1 out]
            n960 = property on="No1Btn" class="Bool"(error in=w2646, "DisabledEnum"=w2641) -> (error out=w2645:errorcluster)  [unwired: 1 in, 1 out]
            n961 = property on="No2Btn" class="Bool"(error in=w2645, "DisabledEnum"=w2641) -> (error out=w2644:errorcluster)  [unwired: 1 in, 1 out]
            n962 = property on="No3Btn" class="Bool"(error in=w2644, "DisabledEnum"=w2641) -> (error out=w2643:errorcluster)  [unwired: 1 in, 1 out]
            n963 = property on="BaseBtn" class="Bool"(error in=w2643, "DisabledEnum"=w2641) -> (error out=w2642:errorcluster)  [unwired: 1 in, 1 out]
            n964 = property on="MotinAdv" class="Bool"(error in=w2642, "DisabledEnum"=w2641) -> ()  [unwired: 1 in, 2 out]
          }
          frame #3 {
            n965 = call "API SYSQUIT.vi"() -> ()  [unwired: 12 in]
            n966 = call "ColorAPI_Quit.vi"() -> ()  [unwired: 11 in, 1 out]
          }
        }
      }
    }
  }
  n967 = while "Plat2-While循环" {
    tunnel: w101 -> [w2670]
    tunnel: w100 -> [w2669]
    tunnel: w99 -> [w2668]
    tunnel: w98 -> [w2667]
    tunnel: w97 -> [w2666]
    tunnel: w28 -> [w2662]
    tunnel: w27 -> [w2663]
    tunnel: w36 -> [w2654]
    tunnel: w35 -> [w2659]
    tunnel: w34 -> [w2655]
    tunnel: w30 -> [w2661]
    tunnel: w26 -> [w2664]
    tunnel: w37 -> [w2658]
    tunnel: w29 -> [w2665]
    tunnel: w33 -> [w2660]
    tunnel: w32 -> [w2657]
    tunnel: w31 -> [w2656]
    stop <- FALSE stop-if-true
    n968 = event shown="[1] \"Plat2Btn\": 值改变" {
      selector: _ -> [_ _ _]
      dyn-events: _ -> [_ _ _]
      timeout: _ -> [_ _ _]
      tunnel: w2670 -> [_ w2746 _]
      tunnel: w2669 -> [_ w2735 _]
      tunnel: w2668 -> [_ w2701 _]
      tunnel: w2667 -> [_ w2689 _]
      tunnel: w2666 -> [_ w2719 _]
      tunnel: w2665 -> [_ w2813 w2821]
      tunnel: w2664 -> [_ w2812 _]
      tunnel: w2663 -> [_ w2811 _]
      tunnel: w2662 -> [_ w2810 _]
      tunnel: w2661 -> [_ w2809 _]
      tunnel: w2660 -> [_ w2808 _]
      tunnel: w2659 -> [_ w2807 _]
      tunnel: w2658 -> [_ w2806 w2834]
      tunnel: w2657 -> [_ w2805 _]
      tunnel: w2656 -> [_ w2804 _]
      tunnel: w2655 -> [_ w2803 _]
      tunnel: w2654 -> [_ w2802 _]
      event Timeout {
        n969 = event-data() -> ()  [unwired: 1 in, 2 out]
      }
      event "Plat2Btn": Value Change {
        n970 = event-data() -> ()  [unwired: 1 in, 5 out]
        n971 = Flush Queue(queue=w2804) -> ()  [unwired: 1 in, 3 out]
        n972 = Flush Queue(queue=w2806) -> ()  [unwired: 1 in, 3 out]
        n973 = Flush Queue(queue=w2812) -> ()  [unwired: 1 in, 3 out]
        n974 = Flush Queue(queue=w2809) -> ()  [unwired: 1 in, 3 out]
        n975 = Flush Queue(queue=w2810) -> (queue out=w2763:refnum<queue>)  [unwired: 1 in, 2 out]
        n976 = Flush Queue(queue=w2811) -> (queue out=w2764:refnum<queue>)  [unwired: 1 in, 2 out]
        n977 = Flush Queue(queue=w2808) -> (queue out=w2777:refnum<queue>)  [unwired: 1 in, 2 out]
        n978 = Flush Queue(queue=w2805) -> (queue out=w2778:refnum<queue>)  [unwired: 1 in, 2 out]
        n979 = Flush Queue(queue=w2802) -> (queue out=w2800:refnum<queue>)  [unwired: 1 in, 2 out]
        n980 = Flush Queue(queue=w2807) -> (queue out=w2801:refnum<queue>)  [unwired: 1 in, 2 out]
        n981 = Flush Queue(queue=w2803) -> (queue out=w2799:refnum<queue>)  [unwired: 1 in, 2 out]
        n982 = control-ref of="Plat2CurrentY"() -> (w2687:refnum<vi>)
        n983 = control-ref of="Plat2CurrentX"() -> (w2700:refnum<vi>)
        n984 = control-ref of="Plat2StopBtn"() -> (w2675:refnum<vi>)
        n985 = Flush Queue(queue=w2813) -> (queue out=w2798:refnum<queue>)  [unwired: 1 in, 2 out]
        n986 = call "QueueMotorStart.vi"("MotorNum"=w2800, "Step"=w2801, "Direction"=w2799, "MotorNum_Int"=3, "Step_Int"=20000, "Direction_Int"=1) -> ("MotorNum_OUT"=w2791:refnum<queue>, "Step_OUT"=w2790:refnum<queue>, "Direction_OUT"=w2789:refnum<queue>, "错误输出"=w2797:errorcluster)  [unwired: 10 in]
        n987 = control-ref of="motor statue array output"() -> (w2674:refnum<vi>)
        n988 = control-ref of="platformStatue1 output"() -> (w2769:refnum<vi>)
        n989 = Enqueue Element(queue=w2798, element=T4."MotorStart" ("元素"), error in (no error)=w2797) -> (queue out=w2784:refnum<queue>, error out=w2792:errorcluster)  [unwired: 1 in, 1 out]
        n990 = call "QueueMotorStart.vi"("MotorNum"=w2791, "Step"=w2790, "Direction"=w2789, "错误输入（无错误）"=w2792, "MotorNum_Int"=4, "Step_Int"=20000, "Direction_Int"=1) -> ("MotorNum_OUT"=w2741:refnum<queue>, "Step_OUT"=w2740:refnum<queue>, "Direction_OUT"=w2739:refnum<queue>, "错误输出"=w2785:errorcluster)  [unwired: 9 in]
        n991 = Enqueue Element(queue=w2784, element=T4."MotorStart" ("元素"), error in (no error)=w2785) -> (queue out=w2772:refnum<queue>, error out=w2782:errorcluster)  [unwired: 1 in, 1 out]
        n992 = call "Check.vi"("错误输入（无错误）"=w2782, "长度"=2, "索引"=2, "Array引用"=w2674, "Bool引用"=w2675) -> ("错误输出"=w2779:errorcluster)  [unwired: 6 in]
        n993 = flat-sequence {
          tunnel: w2779 -> [w2817]
          tunnel: [w2817] -> w2774
          tunnel: w2700 -> [w2816]
          tunnel: w2687 -> [w2815]
          frame #0 {
            w2814 = 0 ("值")
            n994 = property class="DigNum (严格)"(reference=w2815, "Value"=w2814) -> ()  [unwired: 1 in, 2 out]
            n995 = property class="DigNum (严格)"(reference=w2816, "Value"=w2814) -> ()  [unwired: 1 in, 2 out]
          }
        }
        n996 = call "QueueSolenAct.vi"("SolenNum_IN"=w2777, "SolenStatue_IN"=w2778, "SolenNum_Value"=16, "SolenStatue_Value"=1, "错误输入（无错误）"=w2774) -> ("错误输出"=w2773:errorcluster)  [unwired: 8 in, 2 out]
        n997 = Enqueue Element(queue=w2772, element=T4."SolenAction" ("元素"), error in (no error)=w2773) -> (queue out=w2761:refnum<queue>, error out=w2770:errorcluster)  [unwired: 1 in, 1 out]
        n998 = call "Check.vi"("错误输入（无错误）"=w2770, "长度"=1, "索引"=4, "Array引用"=w2769, "Bool引用"=w2675) -> ("错误输出"=w2766:errorcluster)  [unwired: 6 in]
        n999 = call "SpeedControl.vi"("XPos"=w2746, "CurrentX"=w2700, "YPos"=w2735, "CurrentY"=w2687, "SelectPol"=w2719, "错误输入（无错误）"=w2766) -> ("1轴速度"=w2765:i32, "2轴速度"=w2754:i32, "错误输出"=w2760:errorcluster)  [unwired: 11 in]
        n1000 = call "SetSpeedQueue.vi"("MotorNum队列"=w2763, "MotorSpeed队列"=w2764, "MotorNum元素"=3, "MotorSpeed元素"=w2765, "错误输入（无错误）"=w2760) -> ("MotorNum队列输出"=w2756:refnum<queue>, "MotorSpeed队列输出"=w2755:refnum<queue>, "错误输出"=w2759:errorcluster)  [unwired: 8 in]
        n1001 = Enqueue Element(queue=w2761, element=T4."SetMotorSpeed" ("元素"), error in (no error)=w2759) -> (queue out=w2751:refnum<queue>, error out=w2757:errorcluster)  [unwired: 1 in, 1 out]
        n1002 = call "SetSpeedQueue.vi"("MotorNum队列"=w2756, "MotorSpeed队列"=w2755, "MotorNum元素"=4, "MotorSpeed元素"=w2754, "错误输入（无错误）"=w2757) -> ("MotorNum队列输出"=w2715:refnum<queue>, "MotorSpeed队列输出"=w2714:refnum<queue>, "错误输出"=w2752:errorcluster)  [unwired: 8 in]
        n1003 = Enqueue Element(queue=w2751, element=T4."SetMotorSpeed" ("元素"), error in (no error)=w2752) -> (queue out=w2737:refnum<queue>, error out=w2747:errorcluster)  [unwired: 1 in, 1 out]
        n1004 = call "SecondPlatX.vi"("错误输入（无错误）"=w2747, "CurrentX引用"=w2700, "X引用"=w2746) -> ("错误输出"=w2745:errorcluster, "Direction"=w2742:i32, "Step"=w2743:i32, "MotorNum"=w2744:i32)  [unwired: 5 in]
        n1005 = call "QueueMotorStart.vi"("MotorNum"=w2741, "Step"=w2740, "Direction"=w2739, "错误输入（无错误）"=w2745, "MotorNum_Int"=w2744, "Step_Int"=w2743, "Direction_Int"=w2742) -> ("MotorNum_OUT"=w2729:refnum<queue>, "Step_OUT"=w2728:refnum<queue>, "Direction_OUT"=w2727:refnum<queue>, "错误输出"=w2738:errorcluster)  [unwired: 9 in]
        n1006 = Enqueue Element(queue=w2737, element=T4."MotorStart" ("元素"), error in (no error)=w2738) -> (queue out=w2726:refnum<queue>, error out=w2734:errorcluster)  [unwired: 1 in, 1 out]
        n1007 = call "SecondPlatY.vi"("错误输入（无错误）"=w2734, "CurrentY引用"=w2687, "Y引用"=w2735) -> ("错误输出"=w2730:errorcluster, "Direction"=w2731:i32, "Step"=w2732:i32, "MotorNum"=w2733:i32)  [unwired: 5 in]
        n1008 = call "QueueMotorStart.vi"("MotorNum"=w2729, "Step"=w2728, "Direction"=w2727, "错误输入（无错误）"=w2730, "MotorNum_Int"=w2733, "Step_Int"=w2732, "Direction_Int"=w2731) -> ("MotorNum_OUT"=w2695:refnum<queue>, "Step_OUT"=w2694:refnum<queue>, "Direction_OUT"=w2693:refnum<queue>, "错误输出"=w2725:errorcluster)  [unwired: 9 in]
        n1009 = Enqueue Element(queue=w2726, element=T4."MotorStart" ("元素"), error in (no error)=w2725) -> (queue out=w2712:refnum<queue>, error out=w2723:errorcluster)  [unwired: 1 in, 1 out]
        n1010 = call "Check.vi"("错误输入（无错误）"=w2723, "长度"=2, "索引"=2, "Array引用"=w2674, "Bool引用"=w2675) -> ("错误输出"=w2721:errorcluster)  [unwired: 6 in]
        n1011 = call "DelayPlat3.vi"("error In"=w2721, "DelayTime"=u32 300, "Bool"=w2675) -> ("error Out"=w2720:errorcluster)  [unwired: 8 in]
        n1012 = call "SpeedControl.vi"("XPos"=w2701, "CurrentX"=w2700, "YPos"=w2689, "CurrentY"=w2687, "SelectPol"=w2719, "错误输入（无错误）"=w2720) -> ("1轴速度"=w2717:i32, "2轴速度"=w2710:i32, "错误输出"=w2718:errorcluster)  [unwired: 11 in]
        n1013 = call "SetSpeedQueue.vi"("MotorNum队列"=w2715, "MotorSpeed队列"=w2714, "MotorNum元素"=3, "MotorSpeed元素"=w2717, "错误输入（无错误）"=w2718) -> ("MotorNum队列输出"=w2707:refnum<queue>, "MotorSpeed队列输出"=w2706:refnum<queue>, "错误输出"=w2713:errorcluster)  [unwired: 8 in]
        n1014 = Enqueue Element(queue=w2712, element=T4."SetMotorSpeed" ("元素"), error in (no error)=w2713) -> (queue out=w2704:refnum<queue>, error out=w2708:errorcluster)  [unwired: 1 in, 1 out]
        n1015 = call "SetSpeedQueue.vi"("MotorNum队列"=w2707, "MotorSpeed队列"=w2706, "MotorNum元素"=4, "MotorSpeed元素"=w2710, "错误输入（无错误）"=w2708) -> ("错误输出"=w2705:errorcluster)  [unwired: 8 in, 2 out]
        n1016 = Enqueue Element(queue=w2704, element=T4."SetMotorSpeed" ("元素"), error in (no error)=w2705) -> (queue out=w2691:refnum<queue>, error out=w2702:errorcluster)  [unwired: 1 in, 1 out]
        n1017 = call "SecondPlatX.vi"("错误输入（无错误）"=w2702, "CurrentX引用"=w2700, "X引用"=w2701) -> ("错误输出"=w2696:errorcluster, "Direction"=w2697:i32, "Step"=w2698:i32, "MotorNum"=w2699:i32)  [unwired: 5 in]
        n1018 = call "QueueMotorStart.vi"("MotorNum"=w2695, "Step"=w2694, "Direction"=w2693, "错误输入（无错误）"=w2696, "MotorNum_Int"=w2699, "Step_Int"=w2698, "Direction_Int"=w2697) -> ("MotorNum_OUT"=w2682:refnum<queue>, "Step_OUT"=w2681:refnum<queue>, "Direction_OUT"=w2680:refnum<queue>, "错误输出"=w2692:errorcluster)  [unwired: 9 in]
        n1019 = Enqueue Element(queue=w2691, element=T4."MotorStart" ("元素"), error in (no error)=w2692) -> (queue out=w2679:refnum<queue>, error out=w2688:errorcluster)  [unwired: 1 in, 1 out]
        n1020 = call "SecondPlatY.vi"("错误输入（无错误）"=w2688, "CurrentY引用"=w2687, "Y引用"=w2689) -> ("错误输出"=w2683:errorcluster, "Direction"=w2684:i32, "Step"=w2685:i32, "MotorNum"=w2686:i32)  [unwired: 5 in]
        n1021 = call "QueueMotorStart.vi"("MotorNum"=w2682, "Step"=w2681, "Direction"=w2680, "错误输入（无错误）"=w2683, "MotorNum_Int"=w2686, "Step_Int"=w2685, "Direction_Int"=w2684) -> ("错误输出"=w2677:errorcluster)  [unwired: 9 in, 3 out]
        n1022 = Enqueue Element(queue=w2679, element=T4."MotorStart" ("元素"), error in (no error)=w2677) -> (error out=w2676:errorcluster)  [unwired: 1 in, 2 out]
        n1023 = call "Check.vi"("错误输入（无错误）"=w2676, "长度"=2, "索引"=2, "Array引用"=w2674, "Bool引用"=w2675) -> ()  [unwired: 6 in, 1 out]
      }
      event "Plat2StopBtn": Value Change {
        n1024 = event-data() -> ()  [unwired: 1 in, 5 out]
        n1025 = Flush Queue(queue=w2834) -> (queue out=w2833:refnum<queue>, error out=w2831:errorcluster)  [unwired: 1 in, 1 out]
        n1026 = Flush Queue(queue=w2821) -> (queue out=w2820:refnum<queue>)  [unwired: 1 in, 2 out]
        n1027 = Enqueue Element(queue=w2833, element=3 ("元素"), error in (no error)=w2831) -> (queue out=w2828:refnum<queue>, error out=w2830:errorcluster)  [unwired: 1 in, 1 out]
        n1028 = Enqueue Element(queue=w2820, element=T4."MotorStop" ("元素"), error in (no error)=w2830) -> (queue out=w2824:refnum<queue>, error out=w2826:errorcluster)  [unwired: 1 in, 1 out]
        n1029 = Enqueue Element(queue=w2828, element=4 ("元素"), error in (no error)=w2826) -> (error out=w2825:errorcluster)  [unwired: 1 in, 2 out]
        n1030 = Enqueue Element(queue=w2824, element=T4."MotorStop" ("元素"), error in (no error)=w2825) -> (error out=w2822:errorcluster)  [unwired: 1 in, 2 out]
        n1031 = flat-sequence {
          tunnel: w2822 -> [w2835]
          tunnel: [w2835] -> w2819
          frame #0 {
            n1032 = Wait (ms)(milliseconds to wait=u32 200 ("等待时间（毫秒）")) -> ()  [unwired: 1 out]
          }
        }
        n1033 = property on="Plat2StopBtn" class="Bool (严格)"(error in=w2819, "Value"=FALSE ("Plat2StopBtn")) -> ()  [unwired: 1 in, 2 out]
      }
    }
  }
  n1034 = while {
    tunnel: w37 -> [w2856]
    tunnel: w36 -> [w2855]
    tunnel: w35 -> [w2854]
    tunnel: w34 -> [w2853]
    tunnel: w33 -> [w2852]
    tunnel: w32 -> [w2851]
    tunnel: w31 -> [w2850]
    tunnel: w30 -> [w2849]
    tunnel: w29 -> [w2848]
    tunnel: w28 -> [w2847]
    tunnel: w27 -> [w2846]
    tunnel: w26 -> [w2845]
    tunnel: w8 -> [w2844]
    tunnel: w7 -> [w2843]
    tunnel: "Color_String" -> [_]
    tunnel: w6 -> [w2842]
    tunnel: w5 -> [w2841]
    tunnel: w4 -> [w2840]
    tunnel: w3 -> [w2839]
    tunnel: w10 -> [w2838]
    tunnel: w9 -> [w2837]
    stop <- FALSE stop-if-true
    n1035 = event shown="[2] \"TogStartBtn\": 值改变" {
      selector: _ -> [_ _ _]
      dyn-events: _ -> [_ _ _]
      timeout: _ -> [_ _ _]
      tunnel: w2856 -> [_ w2998 w3071]
      tunnel: w2855 -> [_ w2997 w3070]
      tunnel: w2854 -> [_ w2996 w3069]
      tunnel: w2853 -> [_ w2995 w3068]
      tunnel: w2852 -> [_ w2994 w3067]
      tunnel: w2851 -> [_ w2993 w3066]
      tunnel: w2850 -> [_ w2992 w3065]
      tunnel: w2849 -> [_ w2991 w3064]
      tunnel: w2848 -> [_ w2990 w3063]
      tunnel: w2847 -> [_ w2989 w3062]
      tunnel: w2846 -> [_ w2988 w3061]
      tunnel: w2845 -> [_ w2987 w3060]
      tunnel: w2844 -> [_ _ w3041]
      tunnel: w2843 -> [_ _ w3042]
      tunnel: w2842 -> [_ _ w3037]
      tunnel: w2841 -> [_ _ w3036]
      tunnel: w2840 -> [_ _ w3020]
      tunnel: w2839 -> [_ _ w3021]
      tunnel: w2838 -> [_ _ w3018]
      tunnel: w2837 -> [_ _ w3019]
      event Timeout {
        n1036 = event-data() -> ()  [unwired: 1 in, 2 out]
      }
      event "restartbtn": Value Change {
        n1037 = event-data() -> ()  [unwired: 1 in, 5 out]
        n1038 = Flush Queue(queue=w2998) -> ()  [unwired: 1 in, 3 out]
        n1039 = Flush Queue(queue=w2988) -> ()  [unwired: 1 in, 3 out]
        n1040 = Flush Queue(queue=w2989) -> ()  [unwired: 1 in, 3 out]
        n1041 = Flush Queue(queue=w2987) -> ()  [unwired: 1 in, 3 out]
        n1042 = Flush Queue(queue=w2997) -> (queue out=w2914:refnum<queue>)  [unwired: 1 in, 2 out]
        n1043 = Flush Queue(queue=w2996) -> (queue out=w2913:refnum<queue>)  [unwired: 1 in, 2 out]
        n1044 = Flush Queue(queue=w2995) -> (queue out=w2912:refnum<queue>)  [unwired: 1 in, 2 out]
        n1045 = Flush Queue(queue=w2990) -> (queue out=w2986:refnum<queue>)  [unwired: 1 in, 2 out]
        n1046 = Flush Queue(queue=w2992) -> (queue out=w2984:refnum<queue>)  [unwired: 1 in, 2 out]
        n1047 = Flush Queue(queue=w2991) -> (queue out=w2983:refnum<queue>)  [unwired: 1 in, 2 out]
        n1048 = Enqueue Element(queue=w2986, element=T4."FeedMotorStop" ("元素")) -> (queue out=w2979:refnum<queue>, error out=w2980:errorcluster)  [unwired: 2 in, 1 out]
        n1049 = control-ref of="platformStatue0 output"() -> (w2925:refnum<vi>)
        n1050 = control-ref of="platformStatue1 output"() -> (w2920:refnum<vi>)
        n1051 = control-ref of="platformStatue2 output"() -> (w2861:refnum<vi>)
        n1052 = control-ref of="motor statue array output"() -> (w2875:refnum<vi>)
        n1053 = call "QueueSolenAdv.vi"("Statue_IN"=w2984, "PlatNum_IN"=w2983, "Statue_Value"=0, "PlatNum_Value"=0, "错误输入（无错误）"=w2980) -> ("Statue_OUT"=w2976:refnum<queue>, "PlatNum_OUT"=w2975:refnum<queue>, "错误输出"=w2978:errorcluster)  [unwired: 8 in]
        n1054 = Flush Queue(queue=w2994) -> (queue out=w2960:refnum<queue>)  [unwired: 1 in, 2 out]
        n1055 = Flush Queue(queue=w2993) -> (queue out=w2959:refnum<queue>)  [unwired: 1 in, 2 out]
        n1056 = Enqueue Element(queue=w2979, element=T4."SolenAdv" ("元素"), error in (no error)=w2978) -> (queue out=w2974:refnum<queue>, error out=w2973:errorcluster)  [unwired: 1 in, 1 out]
        n1057 = call "QueueSolenAdv.vi"("Statue_IN"=w2976, "PlatNum_IN"=w2975, "Statue_Value"=0, "PlatNum_Value"=1, "错误输入（无错误）"=w2973) -> ("Statue_OUT"=w2969:refnum<queue>, "PlatNum_OUT"=w2968:refnum<queue>, "错误输出"=w2972:errorcluster)  [unwired: 8 in]
        n1058 = Enqueue Element(queue=w2974, element=T4."SolenAdv" ("元素"), error in (no error)=w2972) -> (queue out=w2963:refnum<queue>, error out=w2967:errorcluster)  [unwired: 1 in, 1 out]
        n1059 = call "QueueSolenAdv.vi"("Statue_IN"=w2969, "PlatNum_IN"=w2968, "Statue_Value"=0, "PlatNum_Value"=2, "错误输入（无错误）"=w2967) -> ("错误输出"=w2964:errorcluster)  [unwired: 8 in, 2 out]
        n1060 = Enqueue Element(queue=w2963, element=T4."SolenAdv" ("元素"), error in (no error)=w2964) -> (queue out=w2957:refnum<queue>, error out=w2958:errorcluster)  [unwired: 1 in, 1 out]
        n1061 = call "QueueSolenAct.vi"("SolenNum_IN"=w2960, "SolenStatue_IN"=w2959, "SolenNum_Value"=1, "SolenStatue_Value"=1, "错误输入（无错误）"=w2958) -> ("SolenNum_OUT"=w2952:refnum<queue>, "SolenStatue_OUT"=w2951:refnum<queue>, "错误输出"=w2956:errorcluster)  [unwired: 8 in]
        n1062 = Enqueue Element(queue=w2957, element=T4."SolenAction" ("元素"), error in (no error)=w2956) -> (queue out=w2949:refnum<queue>, error out=w2931:errorcluster)  [unwired: 1 in, 1 out]
        n1063 = control-ref of="stop"() -> (w2864:refnum<vi>)
        n1064 = call "Check.vi"("错误输入（无错误）"=w2931, "长度"=1, "索引"=1, "Array引用"=w2925, "Bool引用"=w2864) -> ("错误输出"=w2928:errorcluster)  [unwired: 6 in]
        n1065 = call "QueueSolenAct.vi"("SolenNum_IN"=w2952, "SolenStatue_IN"=w2951, "SolenNum_Value"=3, "SolenStatue_Value"=1, "错误输入（无错误）"=w2928) -> ("SolenNum_OUT"=w2945:refnum<queue>, "SolenStatue_OUT"=w2944:refnum<queue>, "错误输出"=w2950:errorcluster)  [unwired: 8 in]
        n1066 = Enqueue Element(queue=w2949, element=T4."SolenAction" ("元素"), error in (no error)=w2950) -> (queue out=w2941:refnum<queue>, error out=w2927:errorcluster)  [unwired: 1 in, 1 out]
        n1067 = call "Check.vi"("错误输入（无错误）"=w2927, "长度"=1, "索引"=3, "Array引用"=w2925, "Bool引用"=w2864) -> ("错误输出"=w2926:errorcluster)  [unwired: 6 in]
        n1068 = call "QueueSolenAct.vi"("SolenNum_IN"=w2945, "SolenStatue_IN"=w2944, "SolenNum_Value"=16, "SolenStatue_Value"=1, "错误输入（无错误）"=w2926) -> ("SolenNum_OUT"=w2938:refnum<queue>, "SolenStatue_OUT"=w2937:refnum<queue>, "错误输出"=w2940:errorcluster)  [unwired: 8 in]
        n1069 = Enqueue Element(queue=w2941, element=T4."SolenAction" ("元素"), error in (no error)=w2940) -> (queue out=w2936:refnum<queue>, error out=w2922:errorcluster)  [unwired: 1 in, 1 out]
        n1070 = call "Check.vi"("错误输入（无错误）"=w2922, "长度"=1, "索引"=4, "Array引用"=w2920, "Bool引用"=w2864) -> ("错误输出"=w2921:errorcluster)  [unwired: 6 in]
        n1071 = call "QueueSolenAct.vi"("SolenNum_IN"=w2938, "SolenStatue_IN"=w2937, "SolenNum_Value"=32, "SolenStatue_Value"=1, "错误输入（无错误）"=w2921) -> ("SolenNum_OUT"=w2872:refnum<queue>, "SolenStatue_OUT"=w2871:refnum<queue>, "错误输出"=w2935:errorcluster)  [unwired: 8 in]
        n1072 = Enqueue Element(queue=w2936, element=T4."SolenAction" ("元素"), error in (no error)=w2935) -> (queue out=w2867:refnum<queue>, error out=w2917:errorcluster)  [unwired: 1 in, 1 out]
        n1073 = call "Check.vi"("错误输入（无错误）"=w2917, "长度"=1, "索引"=7, "Array引用"=w2861, "Bool引用"=w2864) -> ("错误输出"=w2870:errorcluster)  [unwired: 6 in]
        n1074 = call "QueueSolenAct.vi"("SolenNum_IN"=w2872, "SolenStatue_IN"=w2871, "SolenNum_Value"=36, "SolenStatue_Value"=1, "错误输入（无错误）"=w2870) -> ("错误输出"=w2865:errorcluster)  [unwired: 8 in, 2 out]
        n1075 = Enqueue Element(queue=w2867, element=T4."SolenAction" ("元素"), error in (no error)=w2865) -> (queue out=w2866:refnum<queue>, error out=w2863:errorcluster)  [unwired: 1 in, 1 out]
        n1076 = call "Check.vi"("错误输入（无错误）"=w2863, "长度"=1, "索引"=4, "Array引用"=w2861, "Bool引用"=w2864) -> ("错误输出"=w2862:errorcluster)  [unwired: 6 in]
        n1077 = call "QueueMotorStart.vi"("MotorNum"=w2914, "Step"=w2913, "Direction"=w2912, "错误输入（无错误）"=w2862, "MotorNum_Int"=3, "Step_Int"=20000, "Direction_Int"=1) -> ("MotorNum_OUT"=w2906:refnum<queue>, "Step_OUT"=w2905:refnum<queue>, "Direction_OUT"=w2904:refnum<queue>, "错误输出"=w2908:errorcluster)  [unwired: 9 in]
        n1078 = Enqueue Element(queue=w2866, element=T4."MotorStart" ("元素"), error in (no error)=w2908) -> (queue out=w2902:refnum<queue>, error out=w2882:errorcluster)  [unwired: 1 in, 1 out]
        n1079 = call "QueueMotorStart.vi"("MotorNum"=w2906, "Step"=w2905, "Direction"=w2904, "错误输入（无错误）"=w2882, "MotorNum_Int"=4, "Step_Int"=20000, "Direction_Int"=1) -> ("MotorNum_OUT"=w2897:refnum<queue>, "Step_OUT"=w2896:refnum<queue>, "Direction_OUT"=w2895:refnum<queue>, "错误输出"=w2903:errorcluster)  [unwired: 9 in]
        n1080 = Enqueue Element(queue=w2902, element=T4."MotorStart" ("元素"), error in (no error)=w2903) -> (queue out=w2893:refnum<queue>, error out=w2881:errorcluster)  [unwired: 1 in, 1 out]
        n1081 = call "QueueMotorStart.vi"("MotorNum"=w2897, "Step"=w2896, "Direction"=w2895, "错误输入（无错误）"=w2881, "MotorNum_Int"=5, "Step_Int"=20000, "Direction_Int"=0) -> ("MotorNum_OUT"=w2892:refnum<queue>, "Step_OUT"=w2891:refnum<queue>, "Direction_OUT"=w2890:refnum<queue>, "错误输出"=w2894:errorcluster)  [unwired: 9 in]
        n1082 = Enqueue Element(queue=w2893, element=T4."MotorStart" ("元素"), error in (no error)=w2894) -> (queue out=w2889:refnum<queue>, error out=w2880:errorcluster)  [unwired: 1 in, 1 out]
        n1083 = call "QueueMotorStart.vi"("MotorNum"=w2892, "Step"=w2891, "Direction"=w2890, "错误输入（无错误）"=w2880, "MotorNum_Int"=6, "Step_Int"=20000, "Direction_Int"=1) -> ("错误输出"=w2879:errorcluster)  [unwired: 9 in, 3 out]
        n1084 = Enqueue Element(queue=w2889, element=T4."MotorStart" ("元素"), error in (no error)=w2879) -> (error out=w2876:errorcluster)  [unwired: 1 in, 2 out]
        n1085 = call "Check.vi"("错误输入（无错误）"=w2876, "长度"=6, "索引"=0, "Array引用"=w2875, "Bool引用"=w2864) -> ()  [unwired: 6 in, 1 out]
      }
      event "TogStartBtn": Value Change {
        n1086 = event-data() -> ()  [unwired: 1 in, 5 out]
        n1087 = Flush Queue(queue=w3071) -> ()  [unwired: 1 in, 3 out]
        n1088 = Flush Queue(queue=w3060) -> ()  [unwired: 1 in, 3 out]
        n1089 = control-ref of="ComboPolicy"() -> (w3016:refnum<vi>)
        n1090 = Flush Queue(queue=w3070) -> (queue out=w3112:refnum<queue>)  [unwired: 1 in, 2 out]
        n1091 = Flush Queue(queue=w3069) -> (queue out=w3111:refnum<queue>)  [unwired: 1 in, 2 out]
        n1092 = Flush Queue(queue=w3068) -> (queue out=w3110:refnum<queue>)  [unwired: 1 in, 2 out]
        n1093 = Flush Queue(queue=w3063) -> (queue out=w3183:refnum<queue>)  [unwired: 1 in, 2 out]
        n1094 = Flush Queue(queue=w3062) -> (queue out=w3028:refnum<queue>)  [unwired: 1 in, 2 out]
        n1095 = Flush Queue(queue=w3061) -> (queue out=w3027:refnum<queue>)  [unwired: 1 in, 2 out]
        n1096 = control-ref of="Plat2SendX"() -> (w3040:refnum<vi>)
        n1097 = control-ref of="Plat2SendY"() -> (w3039:refnum<vi>)
        n1098 = control-ref of="Plat2RecvX"() -> (w3047:refnum<vi>)
        n1099 = control-ref of="Plat2RecvY"() -> (w3046:refnum<vi>)
        n1100 = control-ref of="TogStopBtn"() -> (w2999:refnum<vi>)
        n1101 = control-ref of="电涡流电平"() -> (w3053:refnum<vi>)
        n1102 = control-ref of="SensorWait"() -> (w3054:refnum<vi>)
        n1103 = control-ref of="Plat2SelectPolicy"() -> (w3043:refnum<vi>)
        n1104 = control-ref of="SelectPolicy"() -> (w3029:refnum<vi>)
        n1105 = control-ref of="Plat1SelectPolic1"() -> (w3052:refnum<vi>)
        n1106 = control-ref of="Plat1SelectPolic2"() -> (w3051:refnum<vi>)
        n1107 = control-ref of="Plat2CurrentX_Adv"() -> (w3045:refnum<vi>)
        n1108 = control-ref of="Plat2CurrentY_Adv"() -> (w3044:refnum<vi>)
        n1109 = control-ref of="Sensor array output"() -> (w3058:refnum<vi>)
        n1110 = control-ref of="Plat1_FeedMotorSpeed"() -> (w3057:refnum<vi>)
        n1111 = control-ref of="Plat3CurrentX_Adv"() -> (w3033:refnum<vi>)
        n1112 = control-ref of="Plat3CurrentY_Adv"() -> (w3032:refnum<vi>)
        n1113 = Flush Queue(queue=w3065) -> (queue out=w3181:refnum<queue>)  [unwired: 1 in, 2 out]
        n1114 = Flush Queue(queue=w3064) -> (queue out=w3180:refnum<queue>)  [unwired: 1 in, 2 out]
        n1115 = Enqueue Element(queue=w3183, element=T4."FeedMotorStop" ("元素")) -> (queue out=w3176:refnum<queue>, error out=w3177:errorcluster)  [unwired: 2 in, 1 out]
        n1116 = control-ref of="platformStatue0 output"() -> (w3049:refnum<vi>)
        n1117 = control-ref of="platformStatue1 output"() -> (w3118:refnum<vi>)
        n1118 = control-ref of="platformStatue2 output"() -> (w3002:refnum<vi>)
        n1119 = control-ref of="motor statue array output"() -> (w3022:refnum<vi>)
        n1120 = call "QueueSolenAdv.vi"("Statue_IN"=w3181, "PlatNum_IN"=w3180, "Statue_Value"=0, "PlatNum_Value"=0, "错误输入（无错误）"=w3177) -> ("Statue_OUT"=w3173:refnum<queue>, "PlatNum_OUT"=w3172:refnum<queue>, "错误输出"=w3175:errorcluster)  [unwired: 8 in]
        n1121 = Flush Queue(queue=w3067) -> (queue out=w3157:refnum<queue>)  [unwired: 1 in, 2 out]
        n1122 = Flush Queue(queue=w3066) -> (queue out=w3156:refnum<queue>)  [unwired: 1 in, 2 out]
        n1123 = Enqueue Element(queue=w3176, element=T4."SolenAdv" ("元素"), error in (no error)=w3175) -> (queue out=w3171:refnum<queue>, error out=w3170:errorcluster)  [unwired: 1 in, 1 out]
        n1124 = call "QueueSolenAdv.vi"("Statue_IN"=w3173, "PlatNum_IN"=w3172, "Statue_Value"=0, "PlatNum_Value"=1, "错误输入（无错误）"=w3170) -> ("Statue_OUT"=w3166:refnum<queue>, "PlatNum_OUT"=w3165:refnum<queue>, "错误输出"=w3169:errorcluster)  [unwired: 8 in]
        n1125 = Enqueue Element(queue=w3171, element=T4."SolenAdv" ("元素"), error in (no error)=w3169) -> (queue out=w3160:refnum<queue>, error out=w3164:errorcluster)  [unwired: 1 in, 1 out]
        n1126 = call "QueueSolenAdv.vi"("Statue_IN"=w3166, "PlatNum_IN"=w3165, "Statue_Value"=0, "PlatNum_Value"=2, "错误输入（无错误）"=w3164) -> ("错误输出"=w3161:errorcluster)  [unwired: 8 in, 2 out]
        n1127 = Enqueue Element(queue=w3160, element=T4."SolenAdv" ("元素"), error in (no error)=w3161) -> (queue out=w3154:refnum<queue>, error out=w3155:errorcluster)  [unwired: 1 in, 1 out]
        n1128 = call "QueueSolenAct.vi"("SolenNum_IN"=w3157, "SolenStatue_IN"=w3156, "SolenNum_Value"=1, "SolenStatue_Value"=1, "错误输入（无错误）"=w3155) -> ("SolenNum_OUT"=w3149:refnum<queue>, "SolenStatue_OUT"=w3148:refnum<queue>, "错误输出"=w3153:errorcluster)  [unwired: 8 in]
        n1129 = Enqueue Element(queue=w3154, element=T4."SolenAction" ("元素"), error in (no error)=w3153) -> (queue out=w3146:refnum<queue>, error out=w3128:errorcluster)  [unwired: 1 in, 1 out]
        n1130 = call "Check.vi"("错误输入（无错误）"=w3128, "长度"=1, "索引"=1, "Array引用"=w3049, "Bool引用"=w2999) -> ("错误输出"=w3125:errorcluster)  [unwired: 6 in]
        n1131 = call "QueueSolenAct.vi"("SolenNum_IN"=w3149, "SolenStatue_IN"=w3148, "SolenNum_Value"=3, "SolenStatue_Value"=1, "错误输入（无错误）"=w3125) -> ("SolenNum_OUT"=w3142:refnum<queue>, "SolenStatue_OUT"=w3141:refnum<queue>, "错误输出"=w3147:errorcluster)  [unwired: 8 in]
        n1132 = Enqueue Element(queue=w3146, element=T4."SolenAction" ("元素"), error in (no error)=w3147) -> (queue out=w3138:refnum<queue>, error out=w3124:errorcluster)  [unwired: 1 in, 1 out]
        n1133 = call "Check.vi"("错误输入（无错误）"=w3124, "长度"=1, "索引"=3, "Array引用"=w3049, "Bool引用"=w2999) -> ("错误输出"=w3123:errorcluster)  [unwired: 6 in]
        n1134 = call "QueueSolenAct.vi"("SolenNum_IN"=w3142, "SolenStatue_IN"=w3141, "SolenNum_Value"=16, "SolenStatue_Value"=1, "错误输入（无错误）"=w3123) -> ("SolenNum_OUT"=w3135:refnum<queue>, "SolenStatue_OUT"=w3134:refnum<queue>, "错误输出"=w3137:errorcluster)  [unwired: 8 in]
        n1135 = Enqueue Element(queue=w3138, element=T4."SolenAction" ("元素"), error in (no error)=w3137) -> (queue out=w3133:refnum<queue>, error out=w3120:errorcluster)  [unwired: 1 in, 1 out]
        n1136 = call "Check.vi"("错误输入（无错误）"=w3120, "长度"=1, "索引"=4, "Array引用"=w3118, "Bool引用"=w2999) -> ("错误输出"=w3119:errorcluster)  [unwired: 6 in]
        n1137 = call "QueueSolenAct.vi"("SolenNum_IN"=w3135, "SolenStatue_IN"=w3134, "SolenNum_Value"=32, "SolenStatue_Value"=1, "错误输入（无错误）"=w3119) -> ("SolenNum_OUT"=w3014:refnum<queue>, "SolenStatue_OUT"=w3013:refnum<queue>, "错误输出"=w3132:errorcluster)  [unwired: 8 in]
        n1138 = Enqueue Element(queue=w3133, element=T4."SolenAction" ("元素"), error in (no error)=w3132) -> (queue out=w3008:refnum<queue>, error out=w3115:errorcluster)  [unwired: 1 in, 1 out]
        n1139 = call "Check.vi"("错误输入（无错误）"=w3115, "长度"=1, "索引"=7, "Array引用"=w3002, "Bool引用"=w2999) -> ("错误输出"=w3015:errorcluster)  [unwired: 6 in]
        n1140 = call "QueueSolenAct.vi"("SolenNum_IN"=w3014, "SolenStatue_IN"=w3013, "SolenNum_Value"=36, "SolenStatue_Value"=1, "错误输入（无错误）"=w3015) -> ("SolenNum_OUT"=w3012:refnum<queue>, "SolenStatue_OUT"=w3011:refnum<queue>, "错误输出"=w3007:errorcluster)  [unwired: 8 in]
        n1141 = Enqueue Element(queue=w3008, element=T4."SolenAction" ("元素"), error in (no error)=w3007) -> (queue out=w3005:refnum<queue>, error out=w3004:errorcluster)  [unwired: 1 in, 1 out]
        n1142 = call "Check.vi"("错误输入（无错误）"=w3004, "长度"=1, "索引"=4, "Array引用"=w3002, "Bool引用"=w2999) -> ("错误输出"=w3003:errorcluster)  [unwired: 6 in]
        n1143 = call "QueueMotorStart.vi"("MotorNum"=w3112, "Step"=w3111, "Direction"=w3110, "错误输入（无错误）"=w3003, "MotorNum_Int"=3, "Step_Int"=20000, "Direction_Int"=1) -> ("MotorNum_OUT"=w3104:refnum<queue>, "Step_OUT"=w3103:refnum<queue>, "Direction_OUT"=w3102:refnum<queue>, "错误输出"=w3106:errorcluster)  [unwired: 9 in]
        n1144 = Enqueue Element(queue=w3005, element=T4."MotorStart" ("元素"), error in (no error)=w3106) -> (queue out=w3100:refnum<queue>, error out=w3080:errorcluster)  [unwired: 1 in, 1 out]
        n1145 = call "QueueMotorStart.vi"("MotorNum"=w3104, "Step"=w3103, "Direction"=w3102, "错误输入（无错误）"=w3080, "MotorNum_Int"=4, "Step_Int"=20000, "Direction_Int"=1) -> ("MotorNum_OUT"=w3095:refnum<queue>, "Step_OUT"=w3094:refnum<queue>, "Direction_OUT"=w3093:refnum<queue>, "错误输出"=w3101:errorcluster)  [unwired: 9 in]
        n1146 = Enqueue Element(queue=w3100, element=T4."MotorStart" ("元素"), error in (no error)=w3101) -> (queue out=w3091:refnum<queue>, error out=w3079:errorcluster)  [unwired: 1 in, 1 out]
        n1147 = call "QueueMotorStart.vi"("MotorNum"=w3095, "Step"=w3094, "Direction"=w3093, "错误输入（无错误）"=w3079, "MotorNum_Int"=5, "Step_Int"=20000, "Direction_Int"=0) -> ("MotorNum_OUT"=w3090:refnum<queue>, "Step_OUT"=w3089:refnum<queue>, "Direction_OUT"=w3088:refnum<queue>, "错误输出"=w3092:errorcluster)  [unwired: 9 in]
        n1148 = Enqueue Element(queue=w3091, element=T4."MotorStart" ("元素"), error in (no error)=w3092) -> (queue out=w3087:refnum<queue>, error out=w3078:errorcluster)  [unwired: 1 in, 1 out]
        n1149 = call "QueueMotorStart.vi"("MotorNum"=w3090, "Step"=w3089, "Direction"=w3088, "错误输入（无错误）"=w3078, "MotorNum_Int"=6, "Step_Int"=20000, "Direction_Int"=1) -> ("MotorNum_OUT"=w3025:refnum<queue>, "Step_OUT"=w3024:refnum<queue>, "Direction_OUT"=w3023:refnum<queue>, "错误输出"=w3077:errorcluster)  [unwired: 9 in]
        n1150 = Enqueue Element(queue=w3087, element=T4."MotorStart" ("元素"), error in (no error)=w3077) -> (queue out=w3026:refnum<queue>, error out=w3074:errorcluster)  [unwired: 1 in, 1 out]
        n1151 = call "Check.vi"("错误输入（无错误）"=w3074, "长度"=6, "索引"=0, "Array引用"=w3022, "Bool引用"=w2999) -> ("错误输出"=w3059:errorcluster)  [unwired: 6 in]
        n1152 = flat-sequence {
          tunnel: w3059 -> [w4064]
          tunnel: [w4060] -> w3034
          frame #0 {
            w4059 = 0
            n1153 = property on="Plat2CurrentX_Adv" class="DigNum (严格)"(error in=w4064, "Value"=w4059) -> (error out=w4063:errorcluster)  [unwired: 1 in, 1 out]
            n1154 = property on="Plat2CurrentY_Adv" class="DigNum (严格)"(error in=w4063, "Value"=w4059) -> (error out=w4062:errorcluster)  [unwired: 1 in, 1 out]
            n1155 = property on="Plat3CurrentX_Adv" class="DigNum (严格)"(error in=w4062, "Value"=w4059) -> (error out=w4061:errorcluster)  [unwired: 1 in, 1 out]
            n1156 = property on="Plat3CurrentY_Adv" class="DigNum (严格)"(error in=w4061, "Value"=w4059) -> (error out=w4060:errorcluster)  [unwired: 1 in, 1 out]
          }
        }
        n1157 = while {
          shift-right: [w3408] -> _
          shift-left: enum16{"捡取物料", "放下物料"}."捡取物料" -> [w3416]
          tunnel: w3034 -> [_]
          tunnel: w3012 -> [w3415]
          tunnel: w3011 -> [w3414]
          tunnel: w3026 -> [w3413]
          tunnel: w2999 -> [w3412]
          tunnel: w3002 -> [w3411]
          tunnel: w3037 -> [w3410]
          tunnel: w3036 -> [w3409]
          tunnel: w3021 -> [w3407]
          tunnel: w3020 -> [w3406]
          stop <- w3405 stop-if-true
          n1158 = case shown="\"捡取物料\", 默认" w3416 {
            tunnel: w3415 -> [w3437 w3480]
            tunnel: w3414 -> [w3436 w3479]
            tunnel: w3413 -> [w3433 w3478]
            tunnel: w3412 -> [w3419 w3477]
            tunnel: w3411 -> [w3429 w3476]
            tunnel: w3410 -> [w3426 _]
            tunnel: w3409 -> [w3418 _]
            tunnel: [w3417 w3474] -> w3408
            tunnel: w3407 -> [_ w3482]
            tunnel: w3406 -> [_ w3475]
            frame "捡取物料", Default {
              n1159 = call "QueueSolenAct.vi"("SolenNum_IN"=w3437, "SolenStatue_IN"=w3436, "SolenNum_Value"=32, "SolenStatue_Value"=1) -> ("SolenNum_OUT"=w3422:refnum<queue>, "SolenStatue_OUT"=w3421:refnum<queue>, "错误输出"=w3432:errorcluster)  [unwired: 9 in]
              n1160 = Enqueue Element(queue=w3433, element=T4."SolenAction" ("元素"), error in (no error)=w3432) -> (queue out=w3420:refnum<queue>, error out=w3430:errorcluster)  [unwired: 1 in, 1 out]
              n1161 = call "Check.vi"("错误输入（无错误）"=w3430, "长度"=1, "索引"=7, "Array引用"=w3429, "Bool引用"=w3419) -> ("错误输出"=w3425:errorcluster)  [unwired: 6 in]
              n1162 = Dequeue Element(queue=w3426, error in (no error)=w3425) -> (element=w3424:enum16{"平台2已回到取料点", "NOPE"}, error out=w3423:errorcluster)  [unwired: 1 in, 2 out]
              n1163 = case shown="\"NOPE\"" w3424 {
                tunnel: w3423 -> [w3471 _]
                tunnel: w3422 -> [w3470 _]
                tunnel: w3421 -> [w3469 _]
                tunnel: w3420 -> [w3466 _]
                tunnel: w3419 -> [w3444 _]
                tunnel: w3418 -> [w3441 _]
                tunnel: [w3438 enum16{"捡取物料", "放下物料"}."捡取物料"] -> w3417
                frame "平台2已回到取料点", Default {
                  n1164 = call "QueueSolenAct.vi"("SolenNum_IN"=w3470, "SolenStatue_IN"=w3469, "SolenNum_Value"=34, "SolenStatue_Value"=1, "错误输入（无错误）"=w3471) -> ("SolenNum_OUT"=w3461:refnum<queue>, "SolenStatue_OUT"=w3460:refnum<queue>, "错误输出"=w3465:errorcluster)  [unwired: 8 in]
                  n1165 = Enqueue Element(queue=w3466, element=T4."SolenAction" ("元素"), error in (no error)=w3465) -> (queue out=w3459:refnum<queue>, error out=w3463:errorcluster)  [unwired: 1 in, 1 out]
                  n1166 = call "DelayPlat3.vi"("error In"=w3463, "DelayTime"=u32 1000, "Bool"=w3444) -> ("error Out"=w3458:errorcluster)  [unwired: 8 in]
                  n1167 = call "QueueSolenAct.vi"("SolenNum_IN"=w3461, "SolenStatue_IN"=w3460, "SolenNum_Value"=35, "SolenStatue_Value"=1, "错误输入（无错误）"=w3458) -> ("SolenNum_OUT"=w3453:refnum<queue>, "SolenStatue_OUT"=w3452:refnum<queue>, "错误输出"=w3457:errorcluster)  [unwired: 8 in]
                  n1168 = Enqueue Element(queue=w3459, element=T4."SolenAction" ("元素"), error in (no error)=w3457) -> (queue out=w3448:refnum<queue>, error out=w3451:errorcluster)  [unwired: 1 in, 1 out]
                  n1169 = call "QueueSolenAct.vi"("SolenNum_IN"=w3453, "SolenStatue_IN"=w3452, "SolenNum_Value"=34, "SolenStatue_Value"=0, "错误输入（无错误）"=w3451) -> ("错误输出"=w3447:errorcluster)  [unwired: 8 in, 2 out]
                  n1170 = Enqueue Element(queue=w3448, element=T4."SolenAction" ("元素"), error in (no error)=w3447) -> (error out=w3445:errorcluster)  [unwired: 1 in, 2 out]
                  n1171 = call "DelayPlat3.vi"("error In"=w3445, "DelayTime"=u32 1000, "Bool"=w3444) -> ("error Out"=w3442:errorcluster)  [unwired: 8 in]
                  n1172 = Enqueue Element(queue=w3441, element=enum16{"平台3机械手完成取料动作", "NOPE"}."平台3机械手完成取料动作" ("元素"), error in (no error)=w3442) -> (error out=w3439:errorcluster)  [unwired: 1 in, 2 out]
                  n1173 = flat-sequence {
                    tunnel: w3439 -> [_]
                    tunnel: [enum16{"捡取物料", "放下物料"}."放下物料"] -> w3438
                    frame #0 {
                    }
                  }
                }
                frame "NOPE" {
                }
              }
            }
            frame "放下物料" {
              n1174 = Dequeue Element(queue=w3482) -> (element=w3481:enum16{"平台3放料机构已回到取料点", "NOPE"})  [unwired: 2 in, 3 out]
              n1175 = case shown="\"平台3放料机构已回到取料点\", 默认" w3481 {
                tunnel: w3480 -> [w3528 _]
                tunnel: w3479 -> [w3527 _]
                tunnel: w3478 -> [w3524 _]
                tunnel: w3477 -> [w3486 _]
                tunnel: w3476 -> [w3520 _]
                tunnel: w3475 -> [w3493 _]
                tunnel: [w3490 enum16{"捡取物料", "放下物料"}."放下物料"] -> w3474
                frame "平台3放料机构已回到取料点", Default {
                  w3485 = u32 1000 ("DelayTime")
                  n1176 = call "QueueSolenAct.vi"("SolenNum_IN"=w3528, "SolenStatue_IN"=w3527, "SolenNum_Value"=33, "SolenStatue_Value"=1) -> ("SolenNum_OUT"=w3517:refnum<queue>, "SolenStatue_OUT"=w3516:refnum<queue>, "错误输出"=w3523:errorcluster)  [unwired: 9 in]
                  n1177 = Enqueue Element(queue=w3524, element=T4."SolenAction" ("元素"), error in (no error)=w3523) -> (queue out=w3512:refnum<queue>, error out=w3521:errorcluster)  [unwired: 1 in, 1 out]
                  n1178 = call "Check.vi"("错误输入（无错误）"=w3521, "长度"=1, "索引"=6, "Array引用"=w3520, "Bool引用"=w3486) -> ("错误输出"=w3515:errorcluster)  [unwired: 6 in]
                  n1179 = call "QueueSolenAct.vi"("SolenNum_IN"=w3517, "SolenStatue_IN"=w3516, "SolenNum_Value"=34, "SolenStatue_Value"=1, "错误输入（无错误）"=w3515) -> ("SolenNum_OUT"=w3508:refnum<queue>, "SolenStatue_OUT"=w3507:refnum<queue>, "错误输出"=w3511:errorcluster)  [unwired: 8 in]
                  n1180 = Enqueue Element(queue=w3512, element=T4."SolenAction" ("元素"), error in (no error)=w3511) -> (queue out=w3503:refnum<queue>, error out=w3509:errorcluster)  [unwired: 1 in, 1 out]
                  n1181 = call "DelayPlat3.vi"("error In"=w3509, "DelayTime"=w3485, "Bool"=w3486) -> ("error Out"=w3506:errorcluster)  [unwired: 8 in]
                  n1182 = call "QueueSolenAct.vi"("SolenNum_IN"=w3508, "SolenStatue_IN"=w3507, "SolenNum_Value"=35, "SolenStatue_Value"=0, "错误输入（无错误）"=w3506) -> ("SolenNum_OUT"=w3500:refnum<queue>, "SolenStatue_OUT"=w3499:refnum<queue>, "错误输出"=w3502:errorcluster)  [unwired: 8 in]
                  n1183 = Enqueue Element(queue=w3503, element=T4."SolenAction" ("元素"), error in (no error)=w3502) -> (queue out=w3496:refnum<queue>, error out=w3489:errorcluster)  [unwired: 1 in, 1 out]
                  n1184 = call "DelayPlat3.vi"("error In"=w3489, "DelayTime"=u32 200, "Bool"=w3486) -> ("error Out"=w3488:errorcluster)  [unwired: 8 in]
                  n1185 = call "QueueSolenAct.vi"("SolenNum_IN"=w3500, "SolenStatue_IN"=w3499, "SolenNum_Value"=34, "SolenStatue_Value"=0, "错误输入（无错误）"=w3488) -> ("错误输出"=w3495:errorcluster)  [unwired: 8 in, 2 out]
                  n1186 = Enqueue Element(queue=w3496, element=T4."SolenAction" ("元素"), error in (no error)=w3495) -> (error out=w3484:errorcluster)  [unwired: 1 in, 2 out]
                  n1187 = call "DelayPlat3.vi"("error In"=w3484, "DelayTime"=w3485, "Bool"=w3486) -> ("error Out"=w3483:errorcluster)  [unwired: 8 in]
                  n1188 = Enqueue Element(queue=w3493, element=enum16{"平台3机械手已完成放料动作", "NOPE"}."平台3机械手已完成放料动作" ("元素"), error in (no error)=w3483) -> (error out=w3491:errorcluster)  [unwired: 1 in, 2 out]
                  n1189 = flat-sequence {
                    tunnel: w3491 -> [_]
                    tunnel: [enum16{"捡取物料", "放下物料"}."捡取物料"] -> w3490
                    frame #0 {
                    }
                  }
                }
                frame "NOPE" {
                }
              }
            }
          }
          n1190 = local read "TogStopBtn"() -> (w3405:bool)
        }
        n1191 = while {
          shift-right: [w3538] -> _
          shift-left: enum16{"回一号台接料点", "回二号台接料点"}."回一号台接料点" -> [w3552]
          tunnel: w3047 -> [w3551]
          tunnel: w3046 -> [w3550]
          tunnel: w3045 -> [w3549]
          tunnel: w3044 -> [w3548]
          tunnel: w3043 -> [w3547]
          tunnel: w3028 -> [w3545]
          tunnel: w3027 -> [w3544]
          tunnel: w3026 -> [w3546]
          tunnel: w3025 -> [w3543]
          tunnel: w3024 -> [w3542]
          tunnel: w3023 -> [w3541]
          tunnel: w2999 -> [w3540]
          tunnel: w3022 -> [w3539]
          tunnel: w3042 -> [w3537]
          tunnel: w3041 -> [w3536]
          tunnel: w3037 -> [w3535]
          tunnel: w3036 -> [w3534]
          tunnel: w3034 -> [_]
          tunnel: w3040 -> [w3533]
          tunnel: w3039 -> [w3532]
          stop <- w3531 stop-if-true
          n1192 = case shown="\"回一号台接料点\", 默认" w3552 {
            tunnel: w3551 -> [w3586 w3625]
            tunnel: w3550 -> [w3572 w3624]
            tunnel: w3549 -> [w3585 w3623]
            tunnel: w3548 -> [w3571 w3622]
            tunnel: w3547 -> [w3603 w3621]
            tunnel: w3546 -> [w3597 w3618]
            tunnel: w3545 -> [w3599 w3620]
            tunnel: w3544 -> [w3598 w3619]
            tunnel: w3543 -> [w3579 w3617]
            tunnel: w3542 -> [w3578 w3616]
            tunnel: w3541 -> [w3577 w3615]
            tunnel: w3540 -> [w3560 w3614]
            tunnel: w3539 -> [w3559 w3613]
            tunnel: [w3554 w3626] -> w3538
            tunnel: w3537 -> [w3553 _]
            tunnel: w3536 -> [_ w3629]
            tunnel: w3535 -> [_ w3612]
            tunnel: w3534 -> [_ w3611]
            tunnel: w3533 -> [_ w3610]
            tunnel: w3532 -> [_ w3609]
            frame "回一号台接料点", Default {
              n1193 = call "SpeedControl.vi"("XPos"=w3586, "CurrentX"=w3585, "YPos"=w3572, "CurrentY"=w3571, "SelectPol"=w3603) -> ("1轴速度"=w3601:i32, "2轴速度"=w3592:i32, "错误输出"=w3602:errorcluster)  [unwired: 12 in]
              n1194 = call "SetSpeedQueue.vi"("MotorNum队列"=w3599, "MotorSpeed队列"=w3598, "MotorNum元素"=3, "MotorSpeed元素"=w3601, "错误输入（无错误）"=w3602) -> ("MotorNum队列输出"=w3594:refnum<queue>, "MotorSpeed队列输出"=w3593:refnum<queue>, "错误输出"=w3596:errorcluster)  [unwired: 8 in]
              n1195 = Enqueue Element(queue=w3597, element=T4."SetMotorSpeed" ("元素"), error in (no error)=w3596) -> (queue out=w3589:refnum<queue>, error out=w3590:errorcluster)  [unwired: 1 in, 1 out]
              n1196 = call "SetSpeedQueue.vi"("MotorNum队列"=w3594, "MotorSpeed队列"=w3593, "MotorNum元素"=4, "MotorSpeed元素"=w3592, "错误输入（无错误）"=w3590) -> ("错误输出"=w3588:errorcluster)  [unwired: 8 in, 2 out]
              n1197 = Enqueue Element(queue=w3589, element=T4."SetMotorSpeed" ("元素"), error in (no error)=w3588) -> (queue out=w3576:refnum<queue>, error out=w3584:errorcluster)  [unwired: 1 in, 1 out]
              n1198 = call "SecondPlatX.vi"("错误输入（无错误）"=w3584, "CurrentX引用"=w3585, "X引用"=w3586) -> ("错误输出"=w3583:errorcluster, "Direction"=w3580:i32, "Step"=w3581:i32, "MotorNum"=w3582:i32)  [unwired: 5 in]
              n1199 = call "QueueMotorStart.vi"("MotorNum"=w3579, "Step"=w3578, "Direction"=w3577, "错误输入（无错误）"=w3583, "MotorNum_Int"=w3582, "Step_Int"=w3581, "Direction_Int"=w3580) -> ("MotorNum_OUT"=w3566:refnum<queue>, "Step_OUT"=w3565:refnum<queue>, "Direction_OUT"=w3564:refnum<queue>, "错误输出"=w3575:errorcluster)  [unwired: 9 in]
              n1200 = Enqueue Element(queue=w3576, element=T4."MotorStart" ("元素"), error in (no error)=w3575) -> (queue out=w3558:refnum<queue>, error out=w3573:errorcluster)  [unwired: 1 in, 1 out]
              n1201 = call "SecondPlatY.vi"("错误输入（无错误）"=w3573, "CurrentY引用"=w3571, "Y引用"=w3572) -> ("错误输出"=w3570:errorcluster, "Direction"=w3567:i32, "Step"=w3568:i32, "MotorNum"=w3569:i32)  [unwired: 5 in]
              n1202 = call "QueueMotorStart.vi"("MotorNum"=w3566, "Step"=w3565, "Direction"=w3564, "错误输入（无错误）"=w3570, "MotorNum_Int"=w3569, "Step_Int"=w3568, "Direction_Int"=w3567) -> ("错误输出"=w3563:errorcluster)  [unwired: 9 in, 3 out]
              n1203 = Enqueue Element(queue=w3558, element=T4."MotorStart" ("元素"), error in (no error)=w3563) -> (error out=w3561:errorcluster)  [unwired: 1 in, 2 out]
              n1204 = call "Check.vi"("错误输入（无错误）"=w3561, "长度"=2, "索引"=2, "Array引用"=w3559, "Bool引用"=w3560) -> ("错误输出"=w3555:errorcluster)  [unwired: 6 in]
              n1205 = flat-sequence {
                tunnel: w3555 -> [w3606]
                tunnel: [enum16{"回一号台接料点", "回二号台接料点"}."回二号台接料点"] -> w3554
                tunnel: w3553 -> [w3607]
                tunnel: [w3604] -> _
                frame #0 {
                  n1206 = Enqueue Element(queue=w3607, element=enum16{"平台2已回到接料点", "NOPE"}."平台2已回到接料点" ("元素"), error in (no error)=w3606) -> (error out=w3604:errorcluster)  [unwired: 1 in, 2 out]
                }
              }
            }
            frame "回二号台接料点" {
              n1207 = Dequeue Element(queue=w3629) -> (element=w3628:enum16{"平台1运动完成", "NOPE"}, error out=w3627:errorcluster)  [unwired: 2 in, 2 out]
              n1208 = case shown="\"NOPE\"" w3628 {
                tunnel: w3627 -> [w3685 _]
                tunnel: [w3632 enum16{"回一号台接料点", "回二号台接料点"}."回二号台接料点"] -> w3626
                tunnel: w3625 -> [_ _]
                tunnel: w3624 -> [_ _]
                tunnel: w3623 -> [w3666 _]
                tunnel: w3622 -> [w3655 _]
                tunnel: w3621 -> [w3684 _]
                tunnel: w3620 -> [w3680 _]
                tunnel: w3619 -> [w3679 _]
                tunnel: w3618 -> [w3677 _]
                tunnel: w3617 -> [w3661 _]
                tunnel: w3616 -> [w3660 _]
                tunnel: w3615 -> [w3659 _]
                tunnel: w3614 -> [w3642 _]
                tunnel: w3613 -> [w3641 _]
                tunnel: w3612 -> [w3638 _]
                tunnel: w3611 -> [w3635 _]
                tunnel: w3610 -> [w3631 _]
                tunnel: w3609 -> [w3630 _]
                frame "平台1运动完成", Default {
                  n1209 = call "SpeedControl.vi"("XPos"=w3631, "CurrentX"=w3666, "YPos"=w3630, "CurrentY"=w3655, "SelectPol"=w3684, "错误输入（无错误）"=w3685) -> ("1轴速度"=w3682:i32, "2轴速度"=w3672:i32, "错误输出"=w3683:errorcluster)  [unwired: 11 in]
                  n1210 = call "SetSpeedQueue.vi"("MotorNum队列"=w3680, "MotorSpeed队列"=w3679, "MotorNum元素"=3, "MotorSpeed元素"=w3682, "错误输入（无错误）"=w3683) -> ("MotorNum队列输出"=w3674:refnum<queue>, "MotorSpeed队列输出"=w3673:refnum<queue>, "错误输出"=w3678:errorcluster)  [unwired: 8 in]
                  n1211 = Enqueue Element(queue=w3677, element=T4."SetMotorSpeed" ("元素"), error in (no error)=w3678) -> (queue out=w3670:refnum<queue>, error out=w3675:errorcluster)  [unwired: 1 in, 1 out]
                  n1212 = call "SetSpeedQueue.vi"("MotorNum队列"=w3674, "MotorSpeed队列"=w3673, "MotorNum元素"=4, "MotorSpeed元素"=w3672, "错误输入（无错误）"=w3675) -> ("错误输出"=w3669:errorcluster)  [unwired: 8 in, 2 out]
                  n1213 = Enqueue Element(queue=w3670, element=T4."SetMotorSpeed" ("元素"), error in (no error)=w3669) -> (queue out=w3657:refnum<queue>, error out=w3667:errorcluster)  [unwired: 1 in, 1 out]
                  n1214 = call "SecondPlatX.vi"("错误输入（无错误）"=w3667, "CurrentX引用"=w3666, "X引用"=w3631) -> ("错误输出"=w3662:errorcluster, "Direction"=w3663:i32, "Step"=w3664:i32, "MotorNum"=w3665:i32)  [unwired: 5 in]
                  n1215 = call "QueueMotorStart.vi"("MotorNum"=w3661, "Step"=w3660, "Direction"=w3659, "错误输入（无错误）"=w3662, "MotorNum_Int"=w3665, "Step_Int"=w3664, "Direction_Int"=w3663) -> ("MotorNum_OUT"=w3649:refnum<queue>, "Step_OUT"=w3648:refnum<queue>, "Direction_OUT"=w3647:refnum<queue>, "错误输出"=w3658:errorcluster)  [unwired: 9 in]
                  n1216 = Enqueue Element(queue=w3657, element=T4."MotorStart" ("元素"), error in (no error)=w3658) -> (queue out=w3645:refnum<queue>, error out=w3654:errorcluster)  [unwired: 1 in, 1 out]
                  n1217 = call "SecondPlatY.vi"("错误输入（无错误）"=w3654, "CurrentY引用"=w3655, "Y引用"=w3630) -> ("错误输出"=w3653:errorcluster, "Direction"=w3650:i32, "Step"=w3651:i32, "MotorNum"=w3652:i32)  [unwired: 5 in]
                  n1218 = call "QueueMotorStart.vi"("MotorNum"=w3649, "Step"=w3648, "Direction"=w3647, "错误输入（无错误）"=w3653, "MotorNum_Int"=w3652, "Step_Int"=w3651, "Direction_Int"=w3650) -> ("错误输出"=w3646:errorcluster)  [unwired: 9 in, 3 out]
                  n1219 = Enqueue Element(queue=w3645, element=T4."MotorStart" ("元素"), error in (no error)=w3646) -> (error out=w3643:errorcluster)  [unwired: 1 in, 2 out]
                  n1220 = call "Check.vi"("错误输入（无错误）"=w3643, "长度"=2, "索引"=2, "Array引用"=w3641, "Bool引用"=w3642) -> ("错误输出"=w3637:errorcluster)  [unwired: 6 in]
                  n1221 = Enqueue Element(queue=w3638, element=enum16{"平台2已回到取料点", "NOPE"}."平台2已回到取料点" ("元素"), error in (no error)=w3637) -> (error out=w3634:errorcluster)  [unwired: 1 in, 2 out]
                  n1222 = while {
                    tunnel: w3635 -> [w3691]
                    tunnel: w3634 -> [w3690]
                    tunnel: [w3687] -> w3633
                    stop <- w3688 stop-if-true
                    n1223 = Dequeue Element(queue=w3691, error in (no error)=w3690) -> (element=w3689:enum16{"平台3机械手完成取料动作", "NOPE"}, error out=w3687:errorcluster)  [unwired: 1 in, 2 out]
                    n1224 = case shown="\"平台3机械手完成取料动作\", 默认" w3689 {
                      tunnel: [TRUE FALSE] -> w3688
                      frame "平台3机械手完成取料动作", Default {
                      }
                      frame "NOPE" {
                      }
                    }
                  }
                  n1225 = flat-sequence {
                    tunnel: w3633 -> [_]
                    tunnel: [enum16{"回一号台接料点", "回二号台接料点"}."回一号台接料点"] -> w3632
                    frame #0 {
                    }
                  }
                }
                frame "NOPE" {
                }
              }
            }
          }
          n1226 = local read "TogStopBtn"() -> (w3531:bool)
        }
        n1227 = control-ref of="2to3Pos"() -> (w3055:refnum<vi>)
        n1228 = control-ref of="1to2pos"() -> (w3056:refnum<vi>)
        n1229 = control-ref of="FirstPosX"() -> (w3031:refnum<vi>)
        n1230 = control-ref of="FirstPosZ"() -> (w3030:refnum<vi>)
        n1231 = while {
          shift-right: [w3699] -> _
          shift-left: T14."1号台推料检测" -> [w3717]
          tunnel: w3034 -> [_]
          tunnel: w3012 -> [w3716]
          tunnel: w3011 -> [w3715]
          tunnel: w3026 -> [w3714]
          tunnel: w2999 -> [w3713]
          tunnel: w3058 -> [w3712]
          tunnel: w3025 -> [w3711]
          tunnel: w3024 -> [w3710]
          tunnel: w3023 -> [w3709]
          tunnel: w3028 -> [w3708]
          tunnel: w3027 -> [w3707]
          tunnel: w3057 -> [w3706]
          tunnel: w3056 -> [w3705]
          tunnel: w3055 -> [w3704]
          tunnel: w3054 -> [w3703]
          tunnel: w3053 -> [w3702]
          tunnel: w3052 -> [w3701]
          tunnel: w3051 -> [w3700]
          tunnel: w3049 -> [w3698]
          tunnel: w3042 -> [w3697]
          tunnel: w3041 -> [w3696]
          stop <- w3695 stop-if-true
          n1232 = case shown="\"1号台放料\"" w3717 {
            tunnel: w3716 -> [w3783 w3853 w3865 _ w4040 w4051]
            tunnel: w3715 -> [w3782 w3852 w3864 _ w4039 w4050]
            tunnel: w3714 -> [w3759 w3855 w3866 _ w4046 w4057]
            tunnel: w3713 -> [w3735 w3809 w3863 _ w4042 w4055]
            tunnel: w3712 -> [w3774 w3858 _ _ w4043 w4054]
            tunnel: w3711 -> [w3770 _ _ _ _ _]
            tunnel: w3710 -> [w3769 _ _ _ _ _]
            tunnel: w3709 -> [w3768 _ _ _ _ _]
            tunnel: w3708 -> [w3761 _ _ _ _ _]
            tunnel: w3707 -> [w3760 _ _ _ _ _]
            tunnel: w3706 -> [w3754 _ _ _ _ _]
            tunnel: w3705 -> [w3751 _ _ _ _ _]
            tunnel: w3704 -> [w3750 _ _ _ _ _]
            tunnel: w3703 -> [w3748 _ _ _ _ _]
            tunnel: w3702 -> [w3731 _ _ _ _ _]
            tunnel: w3701 -> [_ _ _ w3926 _ _]
            tunnel: w3700 -> [_ _ _ w3922 _ _]
            tunnel: [w3729 w3814 w3861 w3923 w4037 w4048] -> w3699
            tunnel: w3698 -> [_ w3808 w3862 _ _ _]
            tunnel: w3697 -> [_ _ w3868 _ _ _]
            tunnel: w3696 -> [_ _ w3860 _ _ _]
            frame "1号台推料检测", Default {
              n1233 = property class="DigNum (严格)"(reference=w3750) -> ("Value"=w3739:i32)  [unwired: 1 in, 2 out]
              n1234 = property class="DigNum (严格)"(reference=w3748) -> ("Value"=w3733:i32)  [unwired: 1 in, 2 out]
              n1235 = property class="DigNum (严格)"(reference=w3751) -> ("Value"=w3749:i32)  [unwired: 1 in, 2 out]
              n1236 = property class="DigNum (严格)"(reference=w3754) -> ("Value"=w3753:i32)  [unwired: 1 in, 2 out]
              n1237 = local write "Property_T"("") -> ()
              n1238 = call "SetSpeedQueue.vi"("MotorNum队列"=w3761, "MotorSpeed队列"=w3760, "MotorNum元素"=1, "MotorSpeed元素"=w3753) -> ("错误输出"=w3756:errorcluster)  [unwired: 9 in, 2 out]
              n1239 = Enqueue Element(queue=w3759, element=T4."SetMotorSpeed" ("元素"), error in (no error)=w3756) -> (queue out=w3758:refnum<queue>, error out=w3757:errorcluster)  [unwired: 1 in, 1 out]
              n1240 = Enqueue Element(queue=w3758, element=T4."FeedMotorStart" ("元素"), error in (no error)=w3757) -> (queue out=w3777:refnum<queue>, error out=w3781:errorcluster)  [unwired: 1 in, 1 out]
              n1241 = call "QueueSolenAct.vi"("SolenNum_IN"=w3783, "SolenStatue_IN"=w3782, "SolenNum_Value"=5, "SolenStatue_Value"=1, "错误输入（无错误）"=w3781) -> ("SolenNum_OUT"=w3728:refnum<queue>, "SolenStatue_OUT"=w3727:refnum<queue>, "错误输出"=w3778:errorcluster)  [unwired: 8 in]
              n1242 = Enqueue Element(queue=w3777, element=T4."SolenAction" ("元素"), error in (no error)=w3778) -> (queue out=w3723:refnum<queue>, error out=w3775:errorcluster)  [unwired: 1 in, 1 out]
              n1243 = call "CheckTure.vi"("Bool引用"=w3735, "Array引用"=w3774, "索引"=2, "长度"=1, "错误输入（无错误）"=w3775) -> ("错误输出"=w3721:errorcluster)  [unwired: 10 in]
              n1244 = call "QueueSolenAct.vi"("SolenNum_IN"=w3728, "SolenStatue_IN"=w3727, "SolenNum_Value"=5, "SolenStatue_Value"=0, "错误输入（无错误）"=w3721) -> ("错误输出"=w3724:errorcluster)  [unwired: 8 in, 2 out]
              n1245 = Enqueue Element(queue=w3723, element=T4."SolenAction" ("元素"), error in (no error)=w3724) -> (queue out=w3722:refnum<queue>, error out=w3720:errorcluster)  [unwired: 1 in, 1 out]
              n1246 = Enqueue Element(queue=w3722, element=T4."FeedMotorStop" ("元素"), error in (no error)=w3720) -> (queue out=w3765:refnum<queue>, error out=w3767:errorcluster)  [unwired: 1 in, 1 out]
              n1247 = call "QueueMotorStart.vi"("MotorNum"=w3770, "Step"=w3769, "Direction"=w3768, "错误输入（无错误）"=w3767, "MotorNum_Int"=1, "Step_Int"=w3749, "Direction_Int"=0) -> ("MotorNum_OUT"=w3744:refnum<queue>, "Step_OUT"=w3743:refnum<queue>, "Direction_OUT"=w3742:refnum<queue>, "错误输出"=w3766:errorcluster)  [unwired: 9 in]
              n1248 = Enqueue Element(queue=w3765, element=T4."MotorStart" ("元素"), error in (no error)=w3766) -> (queue out=w3737:refnum<queue>, error out=w3747:errorcluster)  [unwired: 1 in, 1 out]
              n1249 = call "DelayPlat3.vi"("error In"=w3747, "DelayTime"=w3733, "Bool"=w3735) -> ("error Out"=w3746:errorcluster)  [unwired: 8 in]
              n1250 = flat-sequence {
                tunnel: w3746 -> [w3792]
                tunnel: [w3792] -> w3745
                frame #0 {
                  n1251 = local read "Green"() -> (w3801:i32)
                  n1252 = local read "Blue"() -> (w3795:i32)
                  n1253 = local read "Red"() -> (w3803:i32)
                  n1254 = local write "Red_Last"(w3803) -> ()
                  n1255 = local write "Blue_Last"(w3795) -> ()
                  n1256 = local write "Green_Last"(w3801) -> ()
                  n1257 = Multiply(x=w3801, y=256) -> (x*y=w3798:i32)
                  n1258 = Greater?(x=w3795, y=100) -> (0:w3793:bool)
                  n1259 = Multiply(x=w3803, y=65536) -> (x*y=w3799:i32)
                  n1260 = case shown="真" w3793 {
                    frame False {
                      n1261 = local write "Color_String"("其它" ("Color_String")) -> ()
                    }
                    frame True {
                      n1262 = local write "Color_String"("蓝色" ("Color_String")) -> ()
                    }
                  }
                  n1263 = Add(x=w3799, y=w3798) -> (x+y=w3797:i32)
                  n1264 = Add(x=w3797, y=w3795) -> (x+y=w3796:i32)
                  n1265 = local write "Collection_Color"(w3796) -> ()
                }
              }
              n1266 = call "QueueMotorStart.vi"("MotorNum"=w3744, "Step"=w3743, "Direction"=w3742, "错误输入（无错误）"=w3745, "MotorNum_Int"=1, "Step_Int"=w3739, "Direction_Int"=0) -> ("错误输出"=w3738:errorcluster)  [unwired: 9 in, 3 out]
              n1267 = Enqueue Element(queue=w3737, element=T4."MotorStart" ("元素"), error in (no error)=w3738) -> (error out=w3734:errorcluster)  [unwired: 1 in, 2 out]
              n1268 = call "DelayPlat3.vi"("error In"=w3734, "DelayTime"=w3733, "Bool"=w3735) -> ("error Out"=w3732:errorcluster)  [unwired: 8 in]
              n1269 = flat-sequence {
                tunnel: w3732 -> [w3785]
                tunnel: w3731 -> [w3787]
                tunnel: [w3785] -> w3730
                tunnel: [w3791] -> _
                tunnel: w3730 -> [w3791]
                tunnel: [T14."检测策略选择"] -> w3729
                frame #0 {
                  n1270 = property class="DigNum (严格)"(reference=w3787) -> ("Value"=w3786:i32)  [unwired: 1 in, 2 out]
                  n1271 = case shown="0, 默认" w3786 {
                    frame 0, Default {
                      n1272 = local write "Property_T"("非磁性" ("Property_T")) -> ()
                    }
                    frame 1 {
                      n1273 = local write "Property_T"("磁性" ("Property_T")) -> ()
                    }
                  }
                }
                frame #1 {
                }
              }
            }
            frame "1号台取料" {
              n1274 = Enqueue Element(queue=w3855, element=T4."FeedMotorStart" ("元素")) -> (queue out=w3849:refnum<queue>, error out=w3812:errorcluster)  [unwired: 2 in, 1 out]
              n1275 = call "CheckTure.vi"("Bool引用"=w3809, "Array引用"=w3858, "索引"=3, "长度"=1, "错误输入（无错误）"=w3812) -> ("错误输出"=w3813:errorcluster)  [unwired: 10 in]
              n1276 = call "QueueSolenAct.vi"("SolenNum_IN"=w3853, "SolenStatue_IN"=w3852, "SolenNum_Value"=2, "SolenStatue_Value"=1, "错误输入（无错误）"=w3813) -> ("SolenNum_OUT"=w3843:refnum<queue>, "SolenStatue_OUT"=w3841:refnum<queue>, "错误输出"=w3848:errorcluster)  [unwired: 8 in]
              n1277 = Enqueue Element(queue=w3849, element=T4."SolenAction" ("元素"), error in (no error)=w3848) -> (queue out=w3838:refnum<queue>, error out=w3846:errorcluster)  [unwired: 1 in, 1 out]
              n1278 = call "Check.vi"("错误输入（无错误）"=w3846, "长度"=1, "索引"=2, "Array引用"=w3808, "Bool引用"=w3809) -> ("错误输出"=w3842:errorcluster)  [unwired: 6 in]
              n1279 = call "QueueSolenAct.vi"("SolenNum_IN"=w3843, "SolenStatue_IN"=w3841, "SolenNum_Value"=4, "SolenStatue_Value"=1, "错误输入（无错误）"=w3842) -> ("SolenNum_OUT"=w3833:refnum<queue>, "SolenStatue_OUT"=w3832:refnum<queue>, "错误输出"=w3837:errorcluster)  [unwired: 8 in]
              n1280 = Enqueue Element(queue=w3838, element=T4."SolenAction" ("元素"), error in (no error)=w3837) -> (queue out=w3828:refnum<queue>, error out=w3835:errorcluster)  [unwired: 1 in, 1 out]
              n1281 = call "DelayPlat3.vi"("error In"=w3835, "DelayTime"=u32 1000, "Bool"=w3809) -> ("error Out"=w3831:errorcluster)  [unwired: 8 in]
              n1282 = call "QueueSolenAct.vi"("SolenNum_IN"=w3833, "SolenStatue_IN"=w3832, "SolenNum_Value"=3, "SolenStatue_Value"=1, "错误输入（无错误）"=w3831) -> ("SolenNum_OUT"=w3825:refnum<queue>, "SolenStatue_OUT"=w3824:refnum<queue>, "错误输出"=w3827:errorcluster)  [unwired: 8 in]
              n1283 = Enqueue Element(queue=w3828, element=T4."SolenAction" ("元素"), error in (no error)=w3827) -> (queue out=w3820:refnum<queue>, error out=w3811:errorcluster)  [unwired: 1 in, 1 out]
              n1284 = call "Check.vi"("错误输入（无错误）"=w3811, "长度"=1, "索引"=3, "Array引用"=w3808, "Bool引用"=w3809) -> ("错误输出"=w3810:errorcluster)  [unwired: 6 in]
              n1285 = call "QueueSolenAct.vi"("SolenNum_IN"=w3825, "SolenStatue_IN"=w3824, "SolenNum_Value"=0, "SolenStatue_Value"=1, "错误输入（无错误）"=w3810) -> ("错误输出"=w3821:errorcluster)  [unwired: 8 in, 2 out]
              n1286 = Enqueue Element(queue=w3820, element=T4."SolenAction" ("元素"), error in (no error)=w3821) -> (error out=w3818:errorcluster)  [unwired: 1 in, 2 out]
              n1287 = call "Check.vi"("错误输入（无错误）"=w3818, "长度"=1, "索引"=0, "Array引用"=w3808, "Bool引用"=w3809) -> ("错误输出"=w3815:errorcluster)  [unwired: 6 in]
              n1288 = flat-sequence {
                tunnel: w3815 -> [_]
                tunnel: [T14."1号台放料"] -> w3814
                frame #0 {
                }
              }
            }
            frame "1号台放料" {
              n1289 = Dequeue Element(queue=w3868) -> (element=w3867:enum16{"平台2已回到接料点", "NOPE"})  [unwired: 2 in, 3 out]
              n1290 = case shown="\"平台2已回到接料点\", 默认" w3867 {
                tunnel: w3866 -> [w3911 _]
                tunnel: w3865 -> [w3915 _]
                tunnel: w3864 -> [w3914 _]
                tunnel: w3863 -> [w3875 _]
                tunnel: w3862 -> [w3874 _]
                tunnel: [w3870 T14."1号台放料"] -> w3861
                tunnel: w3860 -> [w3869 _]
                frame "平台2已回到接料点", Default {
                  n1291 = call "QueueSolenAct.vi"("SolenNum_IN"=w3915, "SolenStatue_IN"=w3914, "SolenNum_Value"=2, "SolenStatue_Value"=1) -> ("SolenNum_OUT"=w3905:refnum<queue>, "SolenStatue_OUT"=w3904:refnum<queue>, "错误输出"=w3910:errorcluster)  [unwired: 9 in]
                  n1292 = Enqueue Element(queue=w3911, element=T4."SolenAction" ("元素"), error in (no error)=w3910) -> (queue out=w3899:refnum<queue>, error out=w3908:errorcluster)  [unwired: 1 in, 1 out]
                  n1293 = call "Check.vi"("错误输入（无错误）"=w3908, "长度"=1, "索引"=2, "Array引用"=w3874, "Bool引用"=w3875) -> ("错误输出"=w3901:errorcluster)  [unwired: 6 in]
                  n1294 = call "QueueSolenAct.vi"("SolenNum_IN"=w3905, "SolenStatue_IN"=w3904, "SolenNum_Value"=4, "SolenStatue_Value"=0, "错误输入（无错误）"=w3901) -> ("SolenNum_OUT"=w3895:refnum<queue>, "SolenStatue_OUT"=w3894:refnum<queue>, "错误输出"=w3900:errorcluster)  [unwired: 8 in]
                  n1295 = Enqueue Element(queue=w3899, element=T4."SolenAction" ("元素"), error in (no error)=w3900) -> (queue out=w3889:refnum<queue>, error out=w3897:errorcluster)  [unwired: 1 in, 1 out]
                  n1296 = call "DelayPlat3.vi"("error In"=w3897, "DelayTime"=u32 1000, "Bool"=w3875) -> ("error Out"=w3893:errorcluster)  [unwired: 8 in]
                  n1297 = call "QueueSolenAct.vi"("SolenNum_IN"=w3895, "SolenStatue_IN"=w3894, "SolenNum_Value"=3, "SolenStatue_Value"=1, "错误输入（无错误）"=w3893) -> ("SolenNum_OUT"=w3883:refnum<queue>, "SolenStatue_OUT"=w3882:refnum<queue>, "错误输出"=w3890:errorcluster)  [unwired: 8 in]
                  n1298 = Enqueue Element(queue=w3889, element=T4."SolenAction" ("元素"), error in (no error)=w3890) -> (queue out=w3878:refnum<queue>, error out=w3887:errorcluster)  [unwired: 1 in, 1 out]
                  n1299 = call "Check.vi"("错误输入（无错误）"=w3887, "长度"=1, "索引"=3, "Array引用"=w3874, "Bool引用"=w3875) -> ("错误输出"=w3884:errorcluster)  [unwired: 6 in]
                  n1300 = call "QueueSolenAct.vi"("SolenNum_IN"=w3883, "SolenStatue_IN"=w3882, "SolenNum_Value"=1, "SolenStatue_Value"=1, "错误输入（无错误）"=w3884) -> ("错误输出"=w3879:errorcluster)  [unwired: 8 in, 2 out]
                  n1301 = Enqueue Element(queue=w3878, element=T4."SolenAction" ("元素"), error in (no error)=w3879) -> (error out=w3876:errorcluster)  [unwired: 1 in, 2 out]
                  n1302 = call "Check.vi"("错误输入（无错误）"=w3876, "长度"=1, "索引"=1, "Array引用"=w3874, "Bool引用"=w3875) -> ("错误输出"=w3871:errorcluster)  [unwired: 6 in]
                  n1303 = flat-sequence {
                    tunnel: w3871 -> [w3918]
                    tunnel: [T14."1号台推料检测"] -> w3870
                    tunnel: w3869 -> [w3919]
                    tunnel: [w3916] -> _
                    frame #0 {
                      n1304 = Enqueue Element(queue=w3919, element=enum16{"平台1运动完成", "NOPE"}."平台1运动完成" ("元素"), error in (no error)=w3918) -> (error out=w3916:errorcluster)  [unwired: 1 in, 2 out]
                    }
                  }
                }
                frame "NOPE" {
                }
              }
            }
            frame "检测策略选择" {
              n1305 = property class="CmbBox"(reference=w3926) -> ("Value"=w3925:string)  [unwired: 1 in, 2 out]
              n1306 = Decimal String To Number(string=w3925) -> (number=w3924:i32)  [unwired: 2 in, 1 out]
              n1307 = case shown="0, 默认" w3924 {
                tunnel: [w3928 w3958 w3987 w4014] -> w3923
                tunnel: w3922 -> [w3927 w3956 w3985 w4015]
                frame 0, Default {
                  n1308 = local read "Property_T"() -> (w3931:string)
                  n1309 = Equal?(x=w3931, y="非磁性") -> (x = y?=w3929:bool)
                  n1310 = case shown="假" w3929 {
                    tunnel: [w3932 T14."使能取料槽1"] -> w3928
                    tunnel: w3927 -> [w3935 _]
                    frame False {
                      n1311 = property class="CmbBox"(reference=w3935) -> ("Value"=w3934:string)  [unwired: 1 in, 2 out]
                      n1312 = Decimal String To Number(string=w3934) -> (number=w3933:i32)  [unwired: 2 in, 1 out]
                      n1313 = case shown="3" w3933 {
                        tunnel: [w3936 w3942 w3948 T14."1号台取料"] -> w3932
                        frame 0, Default {
                          n1314 = local read "Property_T"() -> (w3938:string)
                          n1315 = Equal?(x=w3938, y="非磁性") -> (x = y?=w3937:bool)
                          n1316 = case shown="假" w3937 {
                            tunnel: [T14."1号台取料" T14."使能取料槽2"] -> w3936
                            frame False {
                            }
                            frame True {
                            }
                          }
                        }
                        frame 1 {
                          n1317 = local read "Property_T"() -> (w3944:string)
                          n1318 = Equal?(x=w3944, y="磁性") -> (x = y?=w3943:bool)
                          n1319 = case shown="假" w3943 {
                            tunnel: [T14."1号台取料" T14."使能取料槽2"] -> w3942
                            frame False {
                            }
                            frame True {
                            }
                          }
                        }
                        frame 2 {
                          n1320 = local read "Blue_Last"() -> (w3951:i32)
                          n1321 = Greater?(x=w3951, y=100) -> (0:w3949:bool)
                          n1322 = case shown="真" w3949 {
                            tunnel: [T14."1号台取料" T14."使能取料槽2"] -> w3948
                            frame False {
                            }
                            frame True {
                            }
                          }
                        }
                        frame 3 {
                        }
                      }
                    }
                    frame True {
                    }
                  }
                }
                frame 1 {
                  n1323 = local read "Property_T"() -> (w3960:string)
                  n1324 = Equal?(x=w3960, y="磁性") -> (x = y?=w3957:bool)
                  n1325 = case shown="假" w3957 {
                    tunnel: [w3961 T14."使能取料槽1"] -> w3958
                    tunnel: w3956 -> [w3964 _]
                    frame False {
                      n1326 = property class="CmbBox"(reference=w3964) -> ("Value"=w3963:string)  [unwired: 1 in, 2 out]
                      n1327 = Decimal String To Number(string=w3963) -> (number=w3962:i32)  [unwired: 2 in, 1 out]
                      n1328 = case shown="2" w3962 {
                        tunnel: [w3965 w3971 w3977 T14."1号台取料"] -> w3961
                        frame 0, Default {
                          n1329 = local read "Property_T"() -> (w3967:string)
                          n1330 = Equal?(x=w3967, y="非磁性") -> (x = y?=w3966:bool)
                          n1331 = case shown="假" w3966 {
                            tunnel: [T14."1号台取料" T14."使能取料槽2"] -> w3965
                            frame False {
                            }
                            frame True {
                            }
                          }
                        }
                        frame 1 {
                          n1332 = local read "Property_T"() -> (w3973:string)
                          n1333 = Equal?(x=w3973, y="磁性") -> (x = y?=w3972:bool)
                          n1334 = case shown="假" w3972 {
                            tunnel: [T14."1号台取料" T14."使能取料槽2"] -> w3971
                            frame False {
                            }
                            frame True {
                            }
                          }
                        }
                        frame 2 {
                          n1335 = local read "Blue_Last"() -> (w3980:i32)
                          n1336 = Greater?(x=w3980, y=100) -> (0:w3978:bool)
                          n1337 = case shown="真" w3978 {
                            tunnel: [T14."1号台取料" T14."使能取料槽2"] -> w3977
                            frame False {
                            }
                            frame True {
                            }
                          }
                        }
                        frame 3 {
                        }
                      }
                    }
                    frame True {
                    }
                  }
                }
                frame 2 {
                  n1338 = local read "Blue_Last"() -> (w3989:i32)
                  n1339 = Greater?(x=w3989, y=100) -> (0:w3986:bool)
                  n1340 = case shown="假" w3986 {
                    tunnel: [w3990 T14."使能取料槽1"] -> w3987
                    tunnel: w3985 -> [w3993 _]
                    frame False {
                      n1341 = property class="CmbBox"(reference=w3993) -> ("Value"=w3992:string)  [unwired: 1 in, 2 out]
                      n1342 = Decimal String To Number(string=w3992) -> (number=w3991:i32)  [unwired: 2 in, 1 out]
                      n1343 = case shown="3" w3991 {
                        tunnel: [w3994 w4000 w4006 T14."1号台取料"] -> w3990
                        frame 0, Default {
                          n1344 = local read "Property_T"() -> (w3996:string)
                          n1345 = Equal?(x=w3996, y="非磁性") -> (x = y?=w3995:bool)
                          n1346 = case shown="假" w3995 {
                            tunnel: [T14."1号台取料" T14."使能取料槽2"] -> w3994
                            frame False {
                            }
                            frame True {
                            }
                          }
                        }
                        frame 1 {
                          n1347 = local read "Property_T"() -> (w4002:string)
                          n1348 = Equal?(x=w4002, y="磁性") -> (x = y?=w4001:bool)
                          n1349 = case shown="假" w4001 {
                            tunnel: [T14."1号台取料" T14."使能取料槽2"] -> w4000
                            frame False {
                            }
                            frame True {
                            }
                          }
                        }
                        frame 2 {
                          n1350 = local read "Blue_Last"() -> (w4009:i32)
                          n1351 = Greater?(x=w4009, y=100) -> (0:w4007:bool)
                          n1352 = case shown="真" w4007 {
                            tunnel: [T14."1号台取料" T14."使能取料槽2"] -> w4006
                            frame False {
                            }
                            frame True {
                            }
                          }
                        }
                        frame 3 {
                        }
                      }
                    }
                    frame True {
                    }
                  }
                }
                frame 3 {
                  n1353 = property class="CmbBox"(reference=w4015) -> ("Value"=w4016:string)  [unwired: 1 in, 2 out]
                  n1354 = Decimal String To Number(string=w4016) -> (number=w4017:i32)  [unwired: 2 in, 1 out]
                  n1355 = case shown="0, 默认" w4017 {
                    tunnel: [w4018 w4024 w4030 T14."1号台取料"] -> w4014
                    frame 0, Default {
                      n1356 = local read "Property_T"() -> (w4020:string)
                      n1357 = Equal?(x=w4020, y="非磁性") -> (x = y?=w4019:bool)
                      n1358 = case shown="假" w4019 {
                        tunnel: [T14."1号台取料" T14."使能取料槽2"] -> w4018
                        frame False {
                        }
                        frame True {
                        }
                      }
                    }
                    frame 1 {
                      n1359 = local read "Property_T"() -> (w4026:string)
                      n1360 = Equal?(x=w4026, y="磁性") -> (x = y?=w4025:bool)
                      n1361 = case shown="假" w4025 {
                        tunnel: [T14."1号台取料" T14."使能取料槽2"] -> w4024
                        frame False {
                        }
                        frame True {
                        }
                      }
                    }
                    frame 2 {
                      n1362 = local read "Blue_Last"() -> (w4033:i32)
                      n1363 = Greater?(x=w4033, y=100) -> (0:w4031:bool)
                      n1364 = case shown="真" w4031 {
                        tunnel: [T14."1号台取料" T14."使能取料槽2"] -> w4030
                        frame False {
                        }
                        frame True {
                        }
                      }
                    }
                    frame 3 {
                    }
                  }
                }
              }
            }
            frame "使能取料槽1" {
              n1365 = Enqueue Element(queue=w4046, element=T4."FeedMotorStop" ("元素")) -> (queue out=w4041:refnum<queue>, error out=w4045:errorcluster)  [unwired: 2 in, 1 out]
              n1366 = call "FirstDumper_Enable.vi"("StopBool引用"=w4042, "SensorArray引用"=w4043, "Cmd"=w4041, "SolenNum_IN"=w4040, "SolenStatue_IN"=w4039, "错误输入（无错误）"=w4045) -> ("错误输出"=w4038:errorcluster)  [unwired: 10 in, 3 out]
              n1367 = flat-sequence {
                tunnel: w4038 -> [_]
                tunnel: [T14."1号台推料检测"] -> w4037
                frame #0 {
                }
              }
            }
            frame "使能取料槽2" {
              n1368 = Enqueue Element(queue=w4057, element=T4."FeedMotorStop" ("元素")) -> (queue out=w4052:refnum<queue>, error out=w4053:errorcluster)  [unwired: 2 in, 1 out]
              n1369 = call "SecondDumper_Enable.vi"("StopBool引用"=w4055, "SensorArray引用"=w4054, "Cmd"=w4052, "SolenNum_IN"=w4051, "SolenStatue_IN"=w4050, "错误输入（无错误）"=w4053) -> ("错误输出"=w4049:errorcluster)  [unwired: 10 in, 3 out]
              n1370 = flat-sequence {
                tunnel: w4049 -> [_]
                tunnel: [T14."1号台推料检测"] -> w4048
                frame #0 {
                }
              }
            }
          }
          n1371 = local read "TogStopBtn"() -> (w3695:bool)
        }
        n1372 = while {
          shift-right: [w3194] -> _
          shift-left: enum16{"回取料点", "放置物料"}."回取料点" -> [w3209]
          tunnel: w3034 -> [_]
          tunnel: w3033 -> [w3208]
          tunnel: w3032 -> [w3207]
          tunnel: w3031 -> [w3206]
          tunnel: w3030 -> [w3205]
          tunnel: w3029 -> [w3204]
          tunnel: w3028 -> [w3203]
          tunnel: w3027 -> [w3202]
          tunnel: w3026 -> [w3201]
          tunnel: w3025 -> [w3200]
          tunnel: w3024 -> [w3199]
          tunnel: w3023 -> [w3198]
          tunnel: w2999 -> [w3197]
          tunnel: w3022 -> [w3196]
          tunnel: w3021 -> [w3195]
          tunnel: w3020 -> [w3193]
          tunnel: w3019 -> [w3192]
          tunnel: w3018 -> [w3191]
          shift-right: [w3185] -> _
          shift-left: 0 -> [w3190]
          tunnel: w3016 -> [w3189]
          tunnel: w3012 -> [w3188]
          tunnel: w3011 -> [w3187]
          tunnel: w3002 -> [w3186]
          stop <- w3184 stop-if-true
          n1373 = case shown="\"放置物料\"" w3209 {
            tunnel: w3208 -> [w3245 w3280]
            tunnel: w3207 -> [w3232 w3279]
            tunnel: w3206 -> [w3246 _]
            tunnel: w3205 -> [w3233 _]
            tunnel: w3204 -> [w3263 w3278]
            tunnel: w3203 -> [w3259 w3277]
            tunnel: w3202 -> [w3258 w3276]
            tunnel: w3201 -> [w3256 w3275]
            tunnel: w3200 -> [w3239 w3274]
            tunnel: w3199 -> [w3238 w3273]
            tunnel: w3198 -> [w3237 w3272]
            tunnel: w3197 -> [w3219 w3271]
            tunnel: w3196 -> [w3218 w3270]
            tunnel: w3195 -> [w3214 _]
            tunnel: [w3211 w3265] -> w3194
            tunnel: w3193 -> [_ w3286]
            tunnel: w3192 -> [_ w3284]
            tunnel: w3191 -> [_ w3283]
            tunnel: w3190 -> [w3210 w3282]
            tunnel: w3189 -> [_ w3281]
            tunnel: w3188 -> [_ w3269]
            tunnel: w3187 -> [_ w3268]
            tunnel: w3186 -> [_ w3267]
            tunnel: [w3210 w3266] -> w3185
            frame "回取料点", Default {
              n1374 = call "SpeedControl.vi"("XPos"=w3246, "CurrentX"=w3245, "YPos"=w3233, "CurrentY"=w3232, "SelectPol"=w3263) -> ("1轴速度"=w3261:i32, "2轴速度"=w3250:i32, "错误输出"=w3262:errorcluster)  [unwired: 12 in]
              n1375 = call "SetSpeedQueue.vi"("MotorNum队列"=w3259, "MotorSpeed队列"=w3258, "MotorNum元素"=5, "MotorSpeed元素"=w3261, "错误输入（无错误）"=w3262) -> ("MotorNum队列输出"=w3254:refnum<queue>, "MotorSpeed队列输出"=w3253:refnum<queue>, "错误输出"=w3257:errorcluster)  [unwired: 8 in]
              n1376 = Enqueue Element(queue=w3256, element=T4."SetMotorSpeed" ("元素"), error in (no error)=w3257) -> (queue out=w3249:refnum<queue>, error out=w3252:errorcluster)  [unwired: 1 in, 1 out]
              n1377 = call "SetSpeedQueue.vi"("MotorNum队列"=w3254, "MotorSpeed队列"=w3253, "MotorNum元素"=6, "MotorSpeed元素"=w3250, "错误输入（无错误）"=w3252) -> ("错误输出"=w3248:errorcluster)  [unwired: 8 in, 2 out]
              n1378 = Enqueue Element(queue=w3249, element=T4."SetMotorSpeed" ("元素"), error in (no error)=w3248) -> (queue out=w3235:refnum<queue>, error out=w3244:errorcluster)  [unwired: 1 in, 1 out]
              n1379 = call "ThridPlatX.vi"("错误输入（无错误）"=w3244, "CurrentX引用"=w3245, "X引用"=w3246) -> ("错误输出"=w3243:errorcluster, "Direction"=w3240:i32, "Step"=w3241:i32, "MotorNum"=w3242:i32)  [unwired: 5 in]
              n1380 = call "QueueMotorStart.vi"("MotorNum"=w3239, "Step"=w3238, "Direction"=w3237, "错误输入（无错误）"=w3243, "MotorNum_Int"=w3242, "Step_Int"=w3241, "Direction_Int"=w3240) -> ("MotorNum_OUT"=w3229:refnum<queue>, "Step_OUT"=w3228:refnum<queue>, "Direction_OUT"=w3227:refnum<queue>, "错误输出"=w3236:errorcluster)  [unwired: 9 in]
              n1381 = Enqueue Element(queue=w3235, element=T4."MotorStart" ("元素"), error in (no error)=w3236) -> (queue out=w3222:refnum<queue>, error out=w3231:errorcluster)  [unwired: 1 in, 1 out]
              n1382 = call "ThridPlatY.vi"("错误输入（无错误）"=w3231, "CurrentY引用"=w3232, "Y引用"=w3233) -> ("错误输出"=w3230:errorcluster, "Direction"=w3224:i32, "Step"=w3225:i32, "MotorNum"=w3226:i32)  [unwired: 5 in]
              n1383 = call "QueueMotorStart.vi"("MotorNum"=w3229, "Step"=w3228, "Direction"=w3227, "错误输入（无错误）"=w3230, "MotorNum_Int"=w3226, "Step_Int"=w3225, "Direction_Int"=w3224) -> ("错误输出"=w3223:errorcluster)  [unwired: 9 in, 3 out]
              n1384 = Enqueue Element(queue=w3222, element=T4."MotorStart" ("元素"), error in (no error)=w3223) -> (error out=w3220:errorcluster)  [unwired: 1 in, 2 out]
              n1385 = call "Check.vi"("错误输入（无错误）"=w3220, "长度"=2, "索引"=4, "Array引用"=w3218, "Bool引用"=w3219) -> ("错误输出"=w3215:errorcluster)  [unwired: 6 in]
              n1386 = Enqueue Element(queue=w3214, element=enum16{"平台3放料机构已回到取料点", "NOPE"}."平台3放料机构已回到取料点" ("元素"), error in (no error)=w3215) -> (error out=w3212:errorcluster)  [unwired: 1 in, 2 out]
              n1387 = flat-sequence {
                tunnel: w3212 -> [_]
                tunnel: [enum16{"回取料点", "放置物料"}."放置物料"] -> w3211
                frame #0 {
                }
              }
            }
            frame "放置物料" {
              n1388 = Dequeue Element(queue=w3286) -> (element=w3285:enum16{"平台3机械手已完成放料动作", "NOPE"})  [unwired: 2 in, 3 out]
              n1389 = case shown="\"平台3机械手已完成放料动作\", 默认" w3285 {
                tunnel: w3284 -> [w3379 _]
                tunnel: w3283 -> [w3378 _]
                tunnel: w3282 -> [w3296 w3403]
                tunnel: w3281 -> [w3384 _]
                tunnel: w3280 -> [w3357 _]
                tunnel: w3279 -> [w3310 _]
                tunnel: w3278 -> [w3375 _]
                tunnel: w3277 -> [w3371 _]
                tunnel: w3276 -> [w3370 _]
                tunnel: w3275 -> [w3368 _]
                tunnel: w3274 -> [w3352 _]
                tunnel: w3273 -> [w3351 _]
                tunnel: w3272 -> [w3350 _]
                tunnel: w3271 -> [w3290 _]
                tunnel: w3270 -> [w3289 _]
                tunnel: w3269 -> [w3330 _]
                tunnel: w3268 -> [w3329 _]
                tunnel: w3267 -> [w3302 _]
                tunnel: [w3295 w3403] -> w3266
                tunnel: [w3294 enum16{"回取料点", "放置物料"}."放置物料"] -> w3265
                frame "平台3机械手已完成放料动作", Default {
                  n1390 = property class="CmbBox"(reference=w3384) -> ("Value"=w3383:string)  [unwired: 1 in, 2 out]
                  n1391 = Quotient & Remainder(x=w3296, y=4) -> (x-y*floor(x/y)=w3381:i32, floor(x/y)=w3386:i32)
                  n1392 = Decimal String To Number(string=w3383) -> (number=w3382:i32)  [unwired: 2 in, 1 out]
                  n1393 = Quotient & Remainder(x=w3386, y=4) -> (x-y*floor(x/y)=w3380:i32)  [unwired: 1 out]
                  n1394 = case shown="0, 默认" w3382 {
                    tunnel: w3381 -> [w3400 w3402]
                    tunnel: w3380 -> [w3399 w3401]
                    tunnel: [w3399 w3402] -> w3377
                    tunnel: [w3400 w3401] -> w3376
                    frame 0, Default {
                    }
                    frame 1 {
                    }
                  }
                  n1395 = Index Array(array=w3379, index=w3377) -> (element=w3358:refnum<vi>)
                  n1396 = Index Array(array=w3378, index=w3376) -> (element=w3345:refnum<vi>)
                  n1397 = call "SpeedControl.vi"("XPos"=w3358, "CurrentX"=w3357, "YPos"=w3345, "CurrentY"=w3310, "SelectPol"=w3375) -> ("1轴速度"=w3373:i32, "2轴速度"=w3363:i32, "错误输出"=w3374:errorcluster)  [unwired: 12 in]
                  n1398 = call "SetSpeedQueue.vi"("MotorNum队列"=w3371, "MotorSpeed队列"=w3370, "MotorNum元素"=5, "MotorSpeed元素"=w3373, "错误输入（无错误）"=w3374) -> ("MotorNum队列输出"=w3366:refnum<queue>, "MotorSpeed队列输出"=w3365:refnum<queue>, "错误输出"=w3369:errorcluster)  [unwired: 8 in]
                  n1399 = Enqueue Element(queue=w3368, element=T4."SetMotorSpeed" ("元素"), error in (no error)=w3369) -> (queue out=w3361:refnum<queue>, error out=w3364:errorcluster)  [unwired: 1 in, 1 out]
                  n1400 = call "SetSpeedQueue.vi"("MotorNum队列"=w3366, "MotorSpeed队列"=w3365, "MotorNum元素"=6, "MotorSpeed元素"=w3363, "错误输入（无错误）"=w3364) -> ("错误输出"=w3360:errorcluster)  [unwired: 8 in, 2 out]
                  n1401 = Enqueue Element(queue=w3361, element=T4."SetMotorSpeed" ("元素"), error in (no error)=w3360) -> (queue out=w3348:refnum<queue>, error out=w3293:errorcluster)  [unwired: 1 in, 1 out]
                  n1402 = call "ThridPlatX.vi"("错误输入（无错误）"=w3293, "CurrentX引用"=w3357, "X引用"=w3358) -> ("错误输出"=w3353:errorcluster, "Direction"=w3354:i32, "Step"=w3355:i32, "MotorNum"=w3356:i32)  [unwired: 5 in]
                  n1403 = call "QueueMotorStart.vi"("MotorNum"=w3352, "Step"=w3351, "Direction"=w3350, "错误输入（无错误）"=w3353, "MotorNum_Int"=w3356, "Step_Int"=w3355, "Direction_Int"=w3354) -> ("MotorNum_OUT"=w3340:refnum<queue>, "Step_OUT"=w3339:refnum<queue>, "Direction_OUT"=w3338:refnum<queue>, "错误输出"=w3349:errorcluster)  [unwired: 9 in]
                  n1404 = Enqueue Element(queue=w3348, element=T4."MotorStart" ("元素"), error in (no error)=w3349) -> (queue out=w3336:refnum<queue>, error out=w3346:errorcluster)  [unwired: 1 in, 1 out]
                  n1405 = call "ThridPlatY.vi"("错误输入（无错误）"=w3346, "CurrentY引用"=w3310, "Y引用"=w3345) -> ("错误输出"=w3341:errorcluster, "Direction"=w3342:i32, "Step"=w3343:i32, "MotorNum"=w3344:i32)  [unwired: 5 in]
                  n1406 = call "QueueMotorStart.vi"("MotorNum"=w3340, "Step"=w3339, "Direction"=w3338, "错误输入（无错误）"=w3341, "MotorNum_Int"=w3344, "Step_Int"=w3343, "Direction_Int"=w3342) -> ("MotorNum_OUT"=w3320:refnum<queue>, "Step_OUT"=w3319:refnum<queue>, "Direction_OUT"=w3318:refnum<queue>, "错误输出"=w3337:errorcluster)  [unwired: 9 in]
                  n1407 = Enqueue Element(queue=w3336, element=T4."MotorStart" ("元素"), error in (no error)=w3337) -> (queue out=w3325:refnum<queue>, error out=w3334:errorcluster)  [unwired: 1 in, 1 out]
                  n1408 = call "Check.vi"("错误输入（无错误）"=w3334, "长度"=2, "索引"=4, "Array引用"=w3289, "Bool引用"=w3290) -> ("错误输出"=w3331:errorcluster)  [unwired: 6 in]
                  n1409 = call "QueueSolenAct.vi"("SolenNum_IN"=w3330, "SolenStatue_IN"=w3329, "SolenNum_Value"=37, "SolenStatue_Value"=1, "错误输入（无错误）"=w3331) -> ("SolenNum_OUT"=w3308:refnum<queue>, "SolenStatue_OUT"=w3307:refnum<queue>, "错误输出"=w3326:errorcluster)  [unwired: 8 in]
                  n1410 = Enqueue Element(queue=w3325, element=T4."SolenAction" ("元素"), error in (no error)=w3326) -> (queue out=w3312:refnum<queue>, error out=w3323:errorcluster)  [unwired: 1 in, 1 out]
                  n1411 = call "Check.vi"("错误输入（无错误）"=w3323, "长度"=1, "索引"=5, "Array引用"=w3302, "Bool引用"=w3290) -> ("错误输出"=w3317:errorcluster)  [unwired: 6 in]
                  n1412 = call "QueueMotorStart.vi"("MotorNum"=w3320, "Step"=w3319, "Direction"=w3318, "错误输入（无错误）"=w3317, "MotorNum_Int"=6, "Step_Int"=500, "Direction_Int"=1) -> ("错误输出"=w3313:errorcluster)  [unwired: 9 in, 3 out]
                  n1413 = Enqueue Element(queue=w3312, element=T4."MotorStart" ("元素"), error in (no error)=w3313) -> (queue out=w3305:refnum<queue>, error out=w3292:errorcluster)  [unwired: 1 in, 1 out]
                  n1414 = call "Check.vi"("错误输入（无错误）"=w3292, "长度"=2, "索引"=4, "Array引用"=w3289, "Bool引用"=w3290) -> ("错误输出"=w3291:errorcluster)  [unwired: 6 in]
                  n1415 = flat-sequence {
                    tunnel: w3310 -> [w3398]
                    tunnel: w3291 -> [w3393]
                    tunnel: [w3391] -> w3309
                    frame #0 {
                      n1416 = property class="DigNum (严格)"(reference=w3398, error in=w3393) -> (reference out=w3395:refnum<vi>, error out=w3392:errorcluster, "Value"=w3397:i32)
                      n1417 = Add(x=w3397, y=500) -> (x+y=w3394:i32)
                      n1418 = property class="DigNum (严格)"(reference=w3395, error in=w3392, "Value"=w3394) -> (error out=w3391:errorcluster)  [unwired: 1 out]
                    }
                  }
                  n1419 = call "QueueSolenAct.vi"("SolenNum_IN"=w3308, "SolenStatue_IN"=w3307, "SolenNum_Value"=36, "SolenStatue_Value"=1, "错误输入（无错误）"=w3309) -> ("错误输出"=w3306:errorcluster)  [unwired: 8 in, 2 out]
                  n1420 = Enqueue Element(queue=w3305, element=T4."SolenAction" ("元素"), error in (no error)=w3306) -> (error out=w3303:errorcluster)  [unwired: 1 in, 2 out]
                  n1421 = call "Check.vi"("错误输入（无错误）"=w3303, "长度"=1, "索引"=4, "Array引用"=w3302, "Bool引用"=w3290) -> ("错误输出"=w3297:errorcluster)  [unwired: 6 in]
                  n1422 = flat-sequence {
                    tunnel: w3297 -> [_]
                    tunnel: w3296 -> [w3390]
                    tunnel: [w3389] -> w3295
                    tunnel: [enum16{"回取料点", "放置物料"}."回取料点"] -> w3294
                    frame #0 {
                      n1423 = Increment(x=w3390) -> (x+1=w3389:i32)
                    }
                  }
                }
                frame "NOPE" {
                }
              }
            }
          }
          n1424 = local read "TogStopBtn"() -> (w3184:bool)
        }
      }
    }
  }
  n1425 = case shown="真" w225 {
    tunnel: w224 -> [w4066 w4070]
    tunnel: w223 -> [w4065 w4069]
    tunnel: w222 -> [_ w4067]
    tunnel: [w4066 w4070] -> w202
    tunnel: [w4065 w4068] -> w201
    frame False {
    }
    frame True {
      n1426 = property on="Horizontal4" class="DigNum (严格)"(error in=w4069, "Value"=w4067) -> (error out=w4068:errorcluster)  [unwired: 1 in, 1 out]
    }
  }
  n1427 = call-poly <vilib>:"Read Key.vi"("section"=w146, "error in (no error)"=w201, "key"="SelectPol", "refnum"=w202) -> ("error out"=w197:errorcluster, "value"=w196:i32, "found?"=w199:bool, "refnum out"=w198:T5)  [unwired: 4 in]
  n1428 = case shown="真" w199 {
    tunnel: w198 -> [w4072 w4076]
    tunnel: w197 -> [w4071 w4074]
    tunnel: w196 -> [_ w4075]
    tunnel: [w4072 w4076] -> w195
    tunnel: [w4071 w4073] -> w194
    frame False {
    }
    frame True {
      n1429 = property on="SelectPolicy" class="RadioBtnsControl (严格)"(error in=w4074, "Value"=w4075) -> (error out=w4073:errorcluster)  [unwired: 1 in, 1 out]
    }
  }
  n1430 = call-poly <vilib>:"Read Key.vi"("section"=w146, "error in (no error)"=w194, "key"="MinSpeed", "refnum"=w195) -> ("error out"=w192:errorcluster, "value"=w190:i32, "found?"=w173:bool, "refnum out"=w193:T5)  [unwired: 4 in]
  n1431 = case shown="真" w173 {
    tunnel: w193 -> [w4078 w4082]
    tunnel: [w4078 w4082] -> w189
    tunnel: w192 -> [w4077 w4080]
    tunnel: w190 -> [_ w4079]
    tunnel: [w4077 w4081] -> w188
    frame False {
    }
    frame True {
      n1432 = property on="MinSpeed" class="DigNum (严格)"(error in=w4080, "Value"=w4079) -> (error out=w4081:errorcluster)  [unwired: 1 in, 1 out]
    }
  }
  n1433 = call-poly <vilib>:"Read Key.vi"("section"=w146, "error in (no error)"=w188, "key"="MaxSpeed", "refnum"=w189) -> ("error out"=w184:errorcluster, "value"=w183:i32, "found?"=w186:bool, "refnum out"=w185:T5)  [unwired: 4 in]
  n1434 = case shown="真" w186 {
    tunnel: w185 -> [w4084 w4088]
    tunnel: w184 -> [w4083 w4086]
    tunnel: w183 -> [_ w4085]
    tunnel: [w4083 w4087] -> w181
    tunnel: [w4084 w4088] -> w182
    frame False {
    }
    frame True {
      n1435 = property on="MaxSpeed" class="DigNum (严格)"(error in=w4086, "Value"=w4085) -> (error out=w4087:errorcluster)  [unwired: 1 in, 1 out]
    }
  }
  n1436 = call-poly <vilib>:"Read Key.vi"("section"=w146, "error in (no error)"=w181, "key"="ComboPol", "refnum"=w182) -> ("error out"=w178:errorcluster, "value"=w176:string, "found?"=w177:bool, "refnum out"=w179:T5)  [unwired: 4 in]
  n1437 = case shown="真" w177 {
    tunnel: w179 -> [w4090 w4091]
    tunnel: w178 -> [w4089 w4093]
    tunnel: w176 -> [_ w4094]
    tunnel: [w4089 w4092] -> w155
    tunnel: [w4090 w4091] -> w156
    frame False {
    }
    frame True {
      n1438 = property on="ComboPolicy" class="CmbBox"(error in=w4093, "Value"=w4094) -> (error out=w4092:errorcluster)  [unwired: 1 in, 1 out]
    }
  }
  n1439 = call-poly <vilib>:"Read Key.vi"("section"=w146, "error in (no error)"=w155, "key"="FirstPosX", "refnum"=w156) -> ("error out"=w151:errorcluster, "value"=w150:i32, "found?"=w153:bool, "refnum out"=w152:T5)  [unwired: 4 in]
  n1440 = case shown="真" w153 {
    tunnel: w152 -> [w4096 w4097]
    tunnel: w151 -> [w4095 w4099]
    tunnel: w150 -> [_ w4100]
    tunnel: [w4095 w4098] -> w147
    tunnel: [w4096 w4097] -> w148
    frame False {
    }
    frame True {
      n1441 = property on="FirstPosX" class="DigNum (严格)"(error in=w4099, "Value"=w4100) -> (error out=w4098:errorcluster)  [unwired: 1 in, 1 out]
    }
  }
  n1442 = call-poly <vilib>:"Read Key.vi"("section"=w146, "error in (no error)"=w147, "key"="FirstPosZ", "refnum"=w148) -> ("error out"=w143:errorcluster, "value"=w142:i32, "found?"=w145:bool, "refnum out"=w144:T5)  [unwired: 4 in]
  n1443 = case shown="真" w145 {
    tunnel: [w4102 w4106] -> w138
    tunnel: w144 -> [w4102 w4106]
    tunnel: w143 -> [w4101 w4104]
    tunnel: w142 -> [_ w4105]
    tunnel: [w4101 w4103] -> w137
    frame False {
    }
    frame True {
      n1444 = property on="FirstPosZ" class="DigNum (严格)"(error in=w4104, "Value"=w4105) -> (error out=w4103:errorcluster)  [unwired: 1 in, 1 out]
    }
  }
  n1445 = call-poly <vilib>:"Read Key.vi"("section"=w110, "error in (no error)"=w137, "key"="RecvX", "refnum"=w138) -> ("error out"=w133:errorcluster, "value"=w134:i32, "found?"=w135:bool, "refnum out"=w132:T5)  [unwired: 4 in]
  n1446 = case shown="真" w135 {
    tunnel: w134 -> [_ w4111]
    tunnel: w133 -> [w4107 w4110]
    tunnel: w132 -> [w4108 w4112]
    tunnel: [w4108 w4112] -> w131
    tunnel: [w4107 w4109] -> w130
    frame False {
    }
    frame True {
      n1447 = property on="Plat2RecvX" class="DigNum (严格)"(error in=w4110, "Value"=w4111) -> (error out=w4109:errorcluster)  [unwired: 1 in, 1 out]
    }
  }
  n1448 = call-poly <vilib>:"Read Key.vi"("section"=w110, "error in (no error)"=w130, "key"="RecvY", "refnum"=w131) -> ("error out"=w125:errorcluster, "value"=w127:i32, "found?"=w128:bool, "refnum out"=w126:T5)  [unwired: 4 in]
  n1449 = case shown="真" w128 {
    tunnel: w127 -> [_ w4118]
    tunnel: w126 -> [w4114 w4115]
    tunnel: w125 -> [w4113 w4117]
    tunnel: [w4113 w4116] -> w123
    tunnel: [w4114 w4115] -> w124
    frame False {
    }
    frame True {
      n1450 = property on="Plat2RecvY" class="DigNum (严格)"(error in=w4117, "Value"=w4118) -> (error out=w4116:errorcluster)  [unwired: 1 in, 1 out]
    }
  }
  n1451 = call-poly <vilib>:"Read Key.vi"("section"=w110, "error in (no error)"=w123, "key"="SendX", "refnum"=w124) -> ("error out"=w119:errorcluster, "value"=w118:i32, "found?"=w121:bool, "refnum out"=w120:T5)  [unwired: 4 in]
  n1452 = case shown="真" w121 {
    tunnel: w120 -> [w4120 w4122]
    tunnel: w119 -> [w4119 w4123]
    tunnel: w118 -> [_ w4124]
    tunnel: [w4120 w4122] -> w116
    tunnel: [w4119 w4121] -> w115
    frame False {
    }
    frame True {
      n1453 = property on="Plat2SendX" class="DigNum (严格)"(error in=w4123, "Value"=w4124) -> (error out=w4121:errorcluster)  [unwired: 1 in, 1 out]
    }
  }
  n1454 = call-poly <vilib>:"Read Key.vi"("section"=w110, "error in (no error)"=w115, "key"="SendY", "refnum"=w116) -> ("error out"=w111:errorcluster, "value"=w112:i32, "found?"=w114:bool, "refnum out"=w113:T5)  [unwired: 4 in]
  n1455 = case shown="真" w114 {
    tunnel: w113 -> [w4126 w4127]
    tunnel: w112 -> [_ w4130]
    tunnel: w111 -> [w4125 w4129]
    tunnel: [w4125 w4128] -> w104
    tunnel: [w4126 w4127] -> w105
    frame False {
    }
    frame True {
      n1456 = property on="Plat2SendY" class="DigNum (严格)"(error in=w4129, "Value"=w4130) -> (error out=w4128:errorcluster)  [unwired: 1 in, 1 out]
    }
  }
  n1457 = call-poly <vilib>:"Read Key.vi"("section"=w110, "error in (no error)"=w104, "key"="SelectPol", "refnum"=w105) -> ("error out"=w106:errorcluster, "value"=w108:i32, "found?"=w109:bool, "refnum out"=w107:T5)  [unwired: 4 in]
  n1458 = case shown="真" w109 {
    tunnel: w108 -> [_ w4136]
    tunnel: w107 -> [w4132 w4133]
    tunnel: w106 -> [w4131 w4135]
    tunnel: [w4131 w4134] -> w94
    tunnel: [w4132 w4133] -> w96
    frame False {
    }
    frame True {
      n1459 = property on="Plat2SelectPolicy" class="RadioBtnsControl (严格)"(error in=w4135, "Value"=w4136) -> (error out=w4134:errorcluster)  [unwired: 1 in, 1 out]
    }
  }
  n1460 = call-poly <vilib>:"Read Key.vi"("section"=w55, "error in (no error)"=w94, "key"="FeedMotorSpeed", "refnum"=w96) -> ("error out"=w91:errorcluster, "value"=w90:i32, "found?"=w92:bool, "refnum out"=w93:T5)  [unwired: 4 in]
  n1461 = case shown="真" w92 {
    tunnel: w93 -> [w4138 w4139]
    tunnel: w91 -> [w4137 w4141]
    tunnel: w90 -> [_ w4142]
    tunnel: [w4137 w4140] -> w88
    tunnel: [w4138 w4139] -> w89
    frame False {
    }
    frame True {
      n1462 = property on="Plat1_FeedMotorSpeed" class="DigNum (严格)"(error in=w4141, "Value"=w4142) -> (error out=w4140:errorcluster)  [unwired: 1 in, 1 out]
    }
  }
  n1463 = call-poly <vilib>:"Read Key.vi"("section"=w55, "error in (no error)"=w88, "key"="1to2Pos", "refnum"=w89) -> ("error out"=w84:errorcluster, "value"=w83:i32, "found?"=w86:bool, "refnum out"=w85:T5)  [unwired: 4 in]
  n1464 = case shown="真" w86 {
    tunnel: w85 -> [w4144 w4146]
    tunnel: w84 -> [w4143 w4148]
    tunnel: w83 -> [_ w4145]
    tunnel: [w4143 w4147] -> w81
    tunnel: [w4144 w4146] -> w82
    frame False {
    }
    frame True {
      n1465 = property on="1to2pos" class="DigNum (严格)"(error in=w4148, "Value"=w4145) -> (error out=w4147:errorcluster)  [unwired: 1 in, 1 out]
    }
  }
  n1466 = call-poly <vilib>:"Read Key.vi"("section"=w55, "error in (no error)"=w81, "key"="2to3Pos", "refnum"=w82) -> ("error out"=w77:errorcluster, "value"=w76:i32, "found?"=w79:bool, "refnum out"=w78:T5)  [unwired: 4 in]
  n1467 = case shown="真" w79 {
    tunnel: w78 -> [w4150 w4151]
    tunnel: w77 -> [w4149 w4154]
    tunnel: w76 -> [_ w4153]
    tunnel: [w4149 w4152] -> w74
    tunnel: [w4150 w4151] -> w75
    frame False {
    }
    frame True {
      n1468 = property on="2to3Pos" class="DigNum (严格)"(error in=w4154, "Value"=w4153) -> (error out=w4152:errorcluster)  [unwired: 1 in, 1 out]
    }
  }
  n1469 = call-poly <vilib>:"Read Key.vi"("section"=w55, "error in (no error)"=w74, "key"="Combo_SelectPolic1", "refnum"=w75) -> ("error out"=w70:errorcluster, "value"=w69:string, "found?"=w72:bool, "refnum out"=w71:T5)  [unwired: 4 in]
  n1470 = case shown="真" w72 {
    tunnel: w71 -> [w4156 w4157]
    tunnel: w70 -> [w4155 w4159]
    tunnel: w69 -> [_ w4160]
    tunnel: [w4155 w4158] -> w67
    tunnel: [w4156 w4157] -> w68
    frame False {
    }
    frame True {
      n1471 = property on="Plat1SelectPolic1" class="CmbBox"(error in=w4159, "Value"=w4160) -> (error out=w4158:errorcluster)  [unwired: 1 in, 1 out]
    }
  }
  n1472 = call-poly <vilib>:"Read Key.vi"("section"=w55, "error in (no error)"=w67, "key"="Combo_SelectPolic2", "refnum"=w68) -> ("error out"=w64:errorcluster, "value"=w63:string, "found?"=w66:bool, "refnum out"=w65:T5)  [unwired: 4 in]
  n1473 = case shown="真" w66 {
    tunnel: w65 -> [w4162 w4166]
    tunnel: w64 -> [w4161 w4164]
    tunnel: w63 -> [_ w4165]
    tunnel: [w4162 w4166] -> w54
    tunnel: [w4161 w4163] -> w53
    frame False {
    }
    frame True {
      n1474 = property on="Plat1SelectPolic2" class="CmbBox"(error in=w4164, "Value"=w4165) -> (error out=w4163:errorcluster)  [unwired: 1 in, 1 out]
    }
  }
  n1475 = call-poly <vilib>:"Read Key.vi"("section"=w55, "error in (no error)"=w53, "key"="SensorWait", "refnum"=w54) -> ("error out"=w50:errorcluster, "value"=w48:i32, "found?"=w51:bool, "refnum out"=w49:T5)  [unwired: 4 in]
  n1476 = case shown="真" w51 {
    tunnel: w50 -> [w4167 w4171]
    tunnel: w49 -> [w4168 w4170]
    tunnel: w48 -> [_ w4172]
    tunnel: [w4168 w4170] -> w46
    tunnel: [w4167 w4169] -> w47
    frame False {
    }
    frame True {
      n1477 = property on="SensorWait" class="DigNum (严格)"(error in=w4171, "Value"=w4172) -> (error out=w4169:errorcluster)  [unwired: 1 in, 1 out]
    }
  }
  n1478 = call <vilib>:"Close Config Data.vi"("error in (no error)"=w47, "refnum"=w46) -> ("error out"=w102:errorcluster)  [unwired: 8 in, 1 out]
  n1479 = property on="X2" class="DigNum (严格)"(error in=w102, "Value"=200.0 ("X2")) -> (error out=w292:errorcluster)  [unwired: 1 in, 1 out]
  n1480 = property on="ComboPolicy" class="CmbBox"("Value"="1" ("ComboPolicy")) -> (error out=w203:errorcluster)  [unwired: 2 in, 1 out]
  n1481 = property on="X1" class="DigNum (严格)"(error in=w292, "Value"=100.0 ("X1")) -> (error out=w294:errorcluster)  [unwired: 1 in, 1 out]
  n1482 = while {
    tunnel: w294 -> [_]
    tunnel: "SelectPolicy" -> [_]
    tunnel: "ComboPolicy" -> [_]
    tunnel: w203 -> [_]
    tunnel: "Plat1_FeedMotorSpeed" -> [_]
    tunnel: "1to2pos" -> [_]
    tunnel: "2to3Pos" -> [_]
    tunnel: "Plat1SelectPolic1" -> [_]
    tunnel: "Plat1SelectPolic2" -> [_]
    tunnel: "SensorWait" -> [_]
    stop <- FALSE stop-if-true
    n1483 = event shown="[9] \"Plat1SetResetConfig\": 值改变" {
      selector: _ -> [_ _ _ _ _ _ _ _ _ _ _]
      dyn-events: _ -> [_ _ _ _ _ _ _ _ _ _ _]
      timeout: _ -> [_ _ _ _ _ _ _ _ _ _ _]
      event Timeout {
        n1484 = event-data() -> ()  [unwired: 1 in, 2 out]
      }
      event "Set1": Value Change {
        n1485 = event-data() -> ()  [unwired: 1 in, 5 out]
        n1486 = property on="电桥电平_Event" class="DigNum (严格)"() -> (error out=w4174:errorcluster, "Value"=w4175:dbl)  [unwired: 2 in, 1 out]
        n1487 = property on="Volt1" class="DigNum (严格)"(error in=w4174, "Value"=w4175) -> ()  [unwired: 1 in, 2 out]
      }
      event "Set2": Value Change {
        n1488 = event-data() -> ()  [unwired: 1 in, 5 out]
        n1489 = property on="电桥电平_Event" class="DigNum (严格)"() -> (error out=w4177:errorcluster, "Value"=w4176:dbl)  [unwired: 2 in, 1 out]
        n1490 = property on="Volt2" class="DigNum (严格)"(error in=w4177, "Value"=w4176) -> ()  [unwired: 1 in, 2 out]
      }
      event "SetReset": Value Change {
        w4179 = 0 ("Horizontal1")
        n1491 = event-data() -> ()  [unwired: 1 in, 5 out]
        n1492 = property on="Horizontal1" class="DigNum (严格)"("Value"=w4179) -> (error out=w4185:errorcluster)  [unwired: 2 in, 1 out]
        n1493 = property on="FirstPosX" class="DigNum (严格)"("Value"=w4179) -> (error out=w4178:errorcluster)  [unwired: 2 in, 1 out]
        n1494 = property on="Vax1" class="DigNum (严格)"("Value"=w4179) -> (error out=w4182:errorcluster)  [unwired: 2 in, 1 out]
        n1495 = property on="FirstPosZ" class="DigNum (严格)"(error in=w4178, "Value"=w4179) -> ()  [unwired: 1 in, 2 out]
        n1496 = property on="Vax2" class="DigNum (严格)"(error in=w4182, "Value"=w4179) -> (error out=w4181:errorcluster)  [unwired: 1 in, 1 out]
        n1497 = property on="Horizontal2" class="DigNum (严格)"(error in=w4185, "Value"=w4179) -> (error out=w4184:errorcluster)  [unwired: 1 in, 1 out]
        n1498 = property on="Vax3" class="DigNum (严格)"(error in=w4181, "Value"=w4179) -> (error out=w4180:errorcluster)  [unwired: 1 in, 1 out]
        n1499 = property on="Vax4" class="DigNum (严格)"(error in=w4180, "Value"=w4179) -> ()  [unwired: 1 in, 2 out]
        n1500 = property on="Horizontal3" class="DigNum (严格)"(error in=w4184, "Value"=w4179) -> (error out=w4183:errorcluster)  [unwired: 1 in, 1 out]
        n1501 = property on="Horizontal4" class="DigNum (严格)"(error in=w4183, "Value"=w4179) -> ()  [unwired: 1 in, 2 out]
      }
      event "SaveParam": Value Change {
        w4192 = "ThridPlat" ("section")
        n1502 = event-data() -> ()  [unwired: 1 in, 5 out]
        n1503 = Current VI's Path() -> (path=w4200:path)
        n1504 = Build Path(base path=w4200, name or relative path="..\\Config.ini" ("名称或相对路径")) -> (appended path=w4198:path)
        n1505 = call <vilib>:"Open Config Data.vi"("create file if necessary (T)"=TRUE, "configuration file path"=w4198) -> ("error out"=w4195:errorcluster, "refnum"=w4196:T5)  [unwired: 7 in, 1 out]
        n1506 = property on="KCalcd" class="DigNum (严格)"() -> ("Value"=w4189:dbl)  [unwired: 2 in, 2 out]
        n1507 = call-poly <vilib>:"Write Key.vi"("section"=w4192, "error in (no error)"=w4195, "value"=w4189, "key"="KValue", "refnum"=w4196) -> ("error out"=w4193:errorcluster, "refnum out"=w4194:T5)  [unwired: 4 in, 1 out]
        n1508 = property on="BCalcd" class="DigNum (严格)"() -> ("Value"=w4188:dbl)  [unwired: 2 in, 2 out]
        n1509 = call-poly <vilib>:"Write Key.vi"("section"=w4192, "error in (no error)"=w4193, "value"=w4188, "key"="BValue", "refnum"=w4194) -> ("error out"=w4186:errorcluster, "refnum out"=w4187:T5)  [unwired: 4 in, 1 out]
        n1510 = call <vilib>:"Close Config Data.vi"("error in (no error)"=w4186, "refnum"=w4187) -> ()  [unwired: 8 in, 2 out]
      }
      event "SaveConfigXZ": Value Change {
        w4205 = "ThridPlat" ("section")
        w4246 = "ThridPlat" ("section")
        w4247 = "ThridPlat" ("section")
        n1511 = event-data() -> ()  [unwired: 1 in, 5 out]
        n1512 = Current VI's Path() -> (path=w4265:path)
        n1513 = Build Path(base path=w4265, name or relative path="..\\Config.ini" ("名称或相对路径")) -> (appended path=w4263:path)
        n1514 = call <vilib>:"Open Config Data.vi"("create file if necessary (T)"=TRUE, "configuration file path"=w4263) -> ("error out"=w4242:errorcluster, "refnum"=w4261:T5)  [unwired: 7 in, 1 out]
        n1515 = property on="Vax1" class="DigNum (严格)"() -> ("Value"=w4259:i32)  [unwired: 2 in, 2 out]
        n1516 = call-poly <vilib>:"Write Key.vi"("section"=w4247, "error in (no error)"=w4242, "value"=w4259, "key"="Z1Pos", "refnum"=w4261) -> ("error out"=w4255:errorcluster, "refnum out"=w4258:T5)  [unwired: 4 in, 1 out]
        n1517 = property on="Vax2" class="DigNum (严格)"() -> ("Value"=w4235:i32)  [unwired: 2 in, 2 out]
        n1518 = call-poly <vilib>:"Write Key.vi"("section"=w4247, "error in (no error)"=w4255, "value"=w4235, "key"="Z2Pos", "refnum"=w4258) -> ("error out"=w4254:errorcluster, "refnum out"=w4257:T5)  [unwired: 4 in, 1 out]
        n1519 = property on="Vax3" class="DigNum (严格)"() -> ("Value"=w4234:i32)  [unwired: 2 in, 2 out]
        n1520 = call-poly <vilib>:"Write Key.vi"("section"=w4247, "error in (no error)"=w4254, "value"=w4234, "key"="Z3Pos", "refnum"=w4257) -> ("error out"=w4253:errorcluster, "refnum out"=w4256:T5)  [unwired: 4 in, 1 out]
        n1521 = property on="Vax4" class="DigNum (严格)"() -> ("Value"=w4232:i32)  [unwired: 2 in, 2 out]
        n1522 = call-poly <vilib>:"Write Key.vi"("section"=w4247, "error in (no error)"=w4253, "value"=w4232, "key"="Z4Pos", "refnum"=w4256) -> ("error out"=w4248:errorcluster, "refnum out"=w4249:T5)  [unwired: 4 in, 1 out]
        n1523 = property on="Horizontal1" class="DigNum (严格)"() -> ("Value"=w4231:i32)  [unwired: 2 in, 2 out]
        n1524 = property on="Horizontal2" class="DigNum (严格)"() -> ("Value"=w4230:i32)  [unwired: 2 in, 2 out]
        n1525 = call-poly <vilib>:"Write Key.vi"("section"=w4246, "error in (no error)"=w4248, "value"=w4231, "key"="X1Pos", "refnum"=w4249) -> ("error out"=w4250:errorcluster, "refnum out"=w4245:T5)  [unwired: 4 in, 1 out]
        n1526 = property on="Horizontal3" class="DigNum (严格)"() -> ("Value"=w4229:i32)  [unwired: 2 in, 2 out]
        n1527 = call-poly <vilib>:"Write Key.vi"("section"=w4246, "error in (no error)"=w4250, "value"=w4230, "key"="X2Pos", "refnum"=w4245) -> ("error out"=w4251:errorcluster, "refnum out"=w4244:T5)  [unwired: 4 in, 1 out]
        n1528 = property on="Horizontal4" class="DigNum (严格)"() -> ("Value"=w4228:i32)  [unwired: 2 in, 2 out]
        n1529 = call-poly <vilib>:"Write Key.vi"("section"=w4246, "error in (no error)"=w4251, "value"=w4229, "key"="X3Pos", "refnum"=w4244) -> ("error out"=w4252:errorcluster, "refnum out"=w4243:T5)  [unwired: 4 in, 1 out]
        n1530 = property on="SelectPolicy" class="RadioBtnsControl (严格)"() -> ("Value"=w4215:enum32{"使用最短路径算法", "使用最短时间算法", "使用默认速度算法"})  [unwired: 2 in, 2 out]
        n1531 = call-poly <vilib>:"Write Key.vi"("section"=w4246, "error in (no error)"=w4252, "value"=w4228, "key"="X4Pos", "refnum"=w4243) -> ("error out"=w4226:errorcluster, "refnum out"=w4227:T5)  [unwired: 4 in, 1 out]
        n1532 = call-poly <vilib>:"Write Key.vi"("section"=w4205, "error in (no error)"=w4226, "value"=w4215, "key"="SelectPol", "refnum"=w4227) -> ("error out"=w4224:errorcluster, "refnum out"=w4225:T5)  [unwired: 4 in, 1 out]
        n1533 = property on="MinSpeed" class="DigNum (严格)"() -> ("Value"=w4214:i32)  [unwired: 2 in, 2 out]
        n1534 = call-poly <vilib>:"Write Key.vi"("section"=w4205, "error in (no error)"=w4224, "value"=w4214, "key"="MinSpeed", "refnum"=w4225) -> ("error out"=w4222:errorcluster, "refnum out"=w4223:T5)  [unwired: 4 in, 1 out]
        n1535 = property on="MaxSpeed" class="DigNum (严格)"() -> ("Value"=w4213:i32)  [unwired: 2 in, 2 out]
        n1536 = property on="ComboPolicy" class="CmbBox"() -> ("Value"=w4212:string)  [unwired: 2 in, 2 out]
        n1537 = call-poly <vilib>:"Write Key.vi"("section"=w4205, "error in (no error)"=w4222, "value"=w4213, "key"="MaxSpeed", "refnum"=w4223) -> ("error out"=w4220:errorcluster, "refnum out"=w4221:T5)  [unwired: 4 in, 1 out]
        n1538 = call-poly <vilib>:"Write Key.vi"("section"=w4205, "error in (no error)"=w4220, "value"=w4212, "key"="ComboPol", "refnum"=w4221) -> ("error out"=w4210:errorcluster, "refnum out"=w4211:T5)  [unwired: 4 in, 1 out]
        n1539 = property on="FirstPosZ" class="DigNum (严格)"() -> ("Value"=w4208:i32)  [unwired: 2 in, 2 out]
        n1540 = call-poly <vilib>:"Write Key.vi"("section"=w4205, "error in (no error)"=w4210, "value"=w4208, "key"="FirstPosZ", "refnum"=w4211) -> ("error out"=w4206:errorcluster, "refnum out"=w4207:T5)  [unwired: 4 in, 1 out]
        n1541 = property on="FirstPosX" class="DigNum (严格)"() -> ("Value"=w4203:i32)  [unwired: 2 in, 2 out]
        n1542 = call-poly <vilib>:"Write Key.vi"("section"=w4205, "error in (no error)"=w4206, "value"=w4203, "key"="FirstPosX", "refnum"=w4207) -> ("error out"=w4201:errorcluster, "refnum out"=w4202:T5)  [unwired: 4 in, 1 out]
        n1543 = call <vilib>:"Close Config Data.vi"("error in (no error)"=w4201, "refnum"=w4202) -> ()  [unwired: 8 in, 2 out]
      }
      event "Plat2SaveConfig": Value Change {
        n1544 = event-data() -> ()  [unwired: 1 in, 5 out]
        n1545 = Current VI's Path() -> (path=w4296:path)
        n1546 = Build Path(base path=w4296, name or relative path="..\\Config.ini" ("名称或相对路径")) -> (appended path=w4294:path)
        n1547 = property on="Plat2RecvX" class="DigNum (严格)"() -> ("Value"=w4272:i32)  [unwired: 2 in, 2 out]
        n1548 = call <vilib>:"Open Config Data.vi"("create file if necessary (T)"=TRUE, "configuration file path"=w4294) -> ("error out"=w4286:errorcluster, "refnum"=w4292:T5)  [unwired: 7 in, 1 out]
        n1549 = call-poly <vilib>:"Write Key.vi"("section"="SecondPlat", "error in (no error)"=w4286, "value"=w4272, "key"="RecvX", "refnum"=w4292) -> ("error out"=w4285:errorcluster, "refnum out"=w4287:T5)  [unwired: 4 in, 1 out]
        n1550 = property on="Plat2RecvY" class="DigNum (严格)"() -> ("Value"=w4271:i32)  [unwired: 2 in, 2 out]
        n1551 = call-poly <vilib>:"Write Key.vi"("section"="SecondPlat", "error in (no error)"=w4285, "value"=w4271, "key"="RecvY", "refnum"=w4287) -> ("error out"=w4281:errorcluster, "refnum out"=w4282:T5)  [unwired: 4 in, 1 out]
        n1552 = property on="Plat2SendX" class="DigNum (严格)"() -> ("Value"=w4270:i32)  [unwired: 2 in, 2 out]
        n1553 = property on="Plat2SendY" class="DigNum (严格)"() -> ("Value"=w4269:i32)  [unwired: 2 in, 2 out]
        n1554 = call-poly <vilib>:"Write Key.vi"("section"="SecondPlat", "error in (no error)"=w4281, "value"=w4270, "key"="SendX", "refnum"=w4282) -> ("error out"=w4277:errorcluster, "refnum out"=w4278:T5)  [unwired: 4 in, 1 out]
        n1555 = call-poly <vilib>:"Write Key.vi"("section"="SecondPlat", "error in (no error)"=w4277, "value"=w4269, "key"="SendY", "refnum"=w4278) -> ("error out"=w4273:errorcluster, "refnum out"=w4274:T5)  [unwired: 4 in, 1 out]
        n1556 = property on="Plat2SelectPolicy" class="RadioBtnsControl (严格)"() -> ("Value"=w4268:enum32{"使用最短路径算法", "使用最短时间算法", "使用默认速度算法"})  [unwired: 2 in, 2 out]
        n1557 = call-poly <vilib>:"Write Key.vi"("section"="SecondPlat", "error in (no error)"=w4273, "value"=w4268, "key"="SelectPol", "refnum"=w4274) -> ("error out"=w4266:errorcluster, "refnum out"=w4267:T5)  [unwired: 4 in, 1 out]
        n1558 = call <vilib>:"Close Config Data.vi"("error in (no error)"=w4266, "refnum"=w4267) -> ()  [unwired: 8 in, 2 out]
      }
      event "Plat2SetResetConfig": Value Change {
        w4297 = 0
        n1559 = event-data() -> ()  [unwired: 1 in, 5 out]
        n1560 = property on="Plat2RecvX" class="DigNum (严格)"("Value"=w4297) -> (error out=w4301:errorcluster)  [unwired: 2 in, 1 out]
        n1561 = property on="Plat2RecvY" class="DigNum (严格)"(error in=w4301, "Value"=w4297) -> (error out=w4300:errorcluster)  [unwired: 1 in, 1 out]
        n1562 = property on="Plat2SendX" class="DigNum (严格)"(error in=w4300, "Value"=w4297) -> (error out=w4299:errorcluster)  [unwired: 1 in, 1 out]
        n1563 = property on="Plat2SendY" class="DigNum (严格)"(error in=w4299, "Value"=w4297) -> (error out=w4298:errorcluster)  [unwired: 1 in, 1 out]
        n1564 = property on="Plat2SelectPolicy" class="RadioBtnsControl (严格)"(error in=w4298, "Value"=w4297) -> ()  [unwired: 1 in, 2 out]
      }
      event "Plat1SaveConfig": Value Change {
        w4304 = "FirstPlat" ("section")
        n1565 = event-data() -> ()  [unwired: 1 in, 5 out]
        n1566 = Current VI's Path() -> (path=w4332:path)
        n1567 = Build Path(base path=w4332, name or relative path="..\\Config.ini" ("名称或相对路径")) -> (appended path=w4330:path)
        n1568 = property on="Plat1_FeedMotorSpeed" class="DigNum (严格)"() -> ("Value"=w4325:i32)  [unwired: 2 in, 2 out]
        n1569 = call <vilib>:"Open Config Data.vi"("create file if necessary (T)"=TRUE, "configuration file path"=w4330) -> ("error out"=w4327:errorcluster, "refnum"=w4328:T5)  [unwired: 7 in, 1 out]
        n1570 = call-poly <vilib>:"Write Key.vi"("section"=w4304, "error in (no error)"=w4327, "value"=w4325, "key"="FeedMotorSpeed", "refnum"=w4328) -> ("error out"=w4323:errorcluster, "refnum out"=w4324:T5)  [unwired: 4 in, 1 out]
        n1571 = property on="1to2pos" class="DigNum (严格)"() -> ("Value"=w4321:i32)  [unwired: 2 in, 2 out]
        n1572 = call-poly <vilib>:"Write Key.vi"("section"=w4304, "error in (no error)"=w4323, "value"=w4321, "key"="1to2Pos", "refnum"=w4324) -> ("error out"=w4319:errorcluster, "refnum out"=w4320:T5)  [unwired: 4 in, 1 out]
        n1573 = property on="2to3Pos" class="DigNum (严格)"() -> ("Value"=w4317:i32)  [unwired: 2 in, 2 out]
        n1574 = property on="Plat1SelectPolic1" class="CmbBox"() -> ("Value"=w4310:string)  [unwired: 2 in, 2 out]
        n1575 = call-poly <vilib>:"Write Key.vi"("section"=w4304, "error in (no error)"=w4319, "value"=w4317, "key"="2to3Pos", "refnum"=w4320) -> ("error out"=w4315:errorcluster, "refnum out"=w4316:T5)  [unwired: 4 in, 1 out]
        n1576 = property on="Plat1SelectPolic2" class="CmbBox"() -> ("Value"=w4309:string)  [unwired: 2 in, 2 out]
        n1577 = call-poly <vilib>:"Write Key.vi"("section"=w4304, "error in (no error)"=w4315, "value"=w4310, "key"="Combo_SelectPolic1", "refnum"=w4316) -> ("error out"=w4311:errorcluster, "refnum out"=w4312:T5)  [unwired: 4 in, 1 out]
        n1578 = property on="SensorWait" class="DigNum (严格)"() -> ("Value"=w4302:i32)  [unwired: 2 in, 2 out]
        n1579 = call-poly <vilib>:"Write Key.vi"("section"=w4304, "error in (no error)"=w4311, "value"=w4309, "key"="Combo_SelectPolic2", "refnum"=w4312) -> ("error out"=w4307:errorcluster, "refnum out"=w4308:T5)  [unwired: 4 in, 1 out]
        n1580 = call-poly <vilib>:"Write Key.vi"("section"=w4304, "error in (no error)"=w4307, "value"=w4302, "key"="SensorWait", "refnum"=w4308) -> ("error out"=w4305:errorcluster, "refnum out"=w4306:T5)  [unwired: 4 in, 1 out]
        n1581 = call <vilib>:"Close Config Data.vi"("error in (no error)"=w4305, "refnum"=w4306) -> ()  [unwired: 1 in, 9 out]
      }
      event "Plat1SetResetConfig": Value Change {
        n1582 = event-data() -> ()  [unwired: 1 in, 5 out]
        n1583 = property on="Plat1_FeedMotorSpeed" class="DigNum (严格)"("Value"=1600) -> (error out=w4343:errorcluster)  [unwired: 2 in, 1 out]
        n1584 = property on="1to2pos" class="DigNum (严格)"(error in=w4343, "Value"=3250 ("1to2pos")) -> (error out=w4342:errorcluster)  [unwired: 1 in, 1 out]
        n1585 = property on="2to3Pos" class="DigNum (严格)"(error in=w4342, "Value"=2000 ("2to3Pos")) -> (error out=w4341:errorcluster)  [unwired: 1 in, 1 out]
        n1586 = property on="Plat1SelectPolic1" class="CmbBox"(error in=w4341, "Value"="5" ("Plat1SelectPolic1")) -> (error out=w4340:errorcluster)  [unwired: 1 in, 1 out]
        n1587 = property on="Plat1SelectPolic2" class="CmbBox"(error in=w4340, "Value"="5" ("Plat1SelectPolic2")) -> (error out=w4334:errorcluster)  [unwired: 1 in, 1 out]
        n1588 = property on="SensorWait" class="DigNum (严格)"(error in=w4334, "Value"=500 ("SensorWait")) -> ()  [unwired: 1 in, 2 out]
      }
      event "CalcKB": Value Change {
        n1589 = event-data() -> ()  [unwired: 1 in, 5 out]
        n1590 = property on="Volt1" class="DigNum (严格)"() -> ("Value"=w4345:dbl)  [unwired: 2 in, 2 out]
        n1591 = property on="Volt2" class="DigNum (严格)"() -> ("Value"=w4344:dbl)  [unwired: 2 in, 2 out]
        n1592 = Not Equal?(x=w4345, y=w4344) -> (x != y?=w4346:bool)
        n1593 = case shown="假" w4346 {
          tunnel: w4345 -> [_ w4356]
          tunnel: w4344 -> [_ w4351]
          frame False {
            n1594 = One Button Dialog(message="计算发生错误 !" ("消息")) -> ()  [unwired: 1 in, 1 out]
          }
          frame True {
            n1595 = property on="X2" class="DigNum (严格)"() -> ("Value"=w4349:dbl)  [unwired: 2 in, 2 out]
            n1596 = property on="X1" class="DigNum (严格)"() -> ("Value"=w4355:dbl)  [unwired: 2 in, 2 out]
            n1597 = Subtract(x=w4356, y=w4351) -> (x-y=w4353:dbl)
            n1598 = Subtract(x=w4355, y=w4349) -> (x-y=w4354:dbl)
            n1599 = Divide(x=w4354, y=w4353) -> (x/y=w4352:dbl)
            n1600 = property on="KCalcd" class="DigNum (严格)"("Value"=w4352) -> ()  [unwired: 2 in, 2 out]
            n1601 = Multiply(x=w4352, y=w4351) -> (x*y=w4350:dbl)
            n1602 = Subtract(x=w4349, y=w4350) -> (x-y=w4348:dbl)
            n1603 = property on="BCalcd" class="DigNum (严格)"("Value"=w4348) -> ()  [unwired: 2 in, 2 out]
          }
        }
      }
    }
  }
  "MaxSpeed 2" <- 1500 ("MaxSpeed 2")
  "MinSpeed 2" <- 50 ("MinSpeed 2")
